vi "myRIO_BRig_RT_v0,71__PortC.vi"() -> ()   [LabVIEW 2014]
uses:
  <vilib>/Platform/TimedLoop/XDataNode/XDataNode.xnode
  <vilib>/Platform/TimedLoop/XDataNode/nitl_modes.ctl
  <vilib>/Platform/TimedLoop/XDataNode/XDNodeRunTimeDep.lvlib
  <vilib>/Platform/TimedLoop/XDataNode/wakeup.ctl
  <vilib>/Platform/TimedLoop/XDataNode/timing_clust.ctl
  <vilib>/rvi/interface/nirviReadWriteControl/nirviReadWriteControl.xnode
  <vilib>/rvi/interface/Simulation/niFpgaSimulationCallBeginRW.vi
  <vilib>/rvi/errors/niLvFpgaAdjustHostInterfaceError.vi
  <vilib>/rvi/interface/nirviCloseFPGA/nirviCloseFPGA.xnode
  <vilib>/myRIO/Instrument Drivers/Utilities/Utilities.lvlib
  <vilib>/rvi/interface/nirviOpenFPGA/nirviOpenFPGA.xnode
  myRIO_BRig_RT__Case_Exp_stateList.ctl
  <vilib>/WebDAVClient/Advanced/SessionHandle.ctl
  <vilib>/WebDAVClient/NI_WebDAV.lvlib
  myRIO_BRig_RT__Case_NonExp_stateList.ctl
  NiFpgaLv.dll
  <vilib>/Utility/error.llb/Error Cluster From Error Code.vi
  myRIO_BRig_FPGA_v3,60__PortC__build.lvbitx
  myRIO_BRig_FPGA_v3,60__PortC.vi
  <vilib>/FPGAPlugInAG/myRIO-1900/niLvFpga_Open_myRIO-1900.vi
  <vilib>/rvi/interface/common/dynamic/niFpgaDynamicAddResources.vi
  <vilib>/FPGAPlugInAG/Dynamic/niLvFpga_Close_Dynamic.vi
panel:
  out "I_connect_TCP":bool
  out "tempAI0":i16
  out "error out 5":errorcluster
  in  "get_countPerMS":bool
  in  "count_warmup_R_reset":bool
  in  "count_warmup_L_reset":bool
  out "count_warmup_R":u16
  out "count_warmup_L":u16
  out "SolenoidReward":bool
  in  "SolenoidProbability_L":u16=50 caption="Reward Time [ms]" min=1 max=1000 step=1
  in  "SolenoidProbability_R":u16=50 caption="Reward Time [ms]" min=1 max=1000 step=1
  out "output_PortA":dbl caption="LaserPower"
  out "error out 4":errorcluster
  in  "laser_power_step":dbl
  in  "laser_power_max":dbl
  in  "Recording":bool
  out "error out 3":errorcluster
  out "error out 2":errorcluster
  in  "laser_power_min":dbl
  in  "f_millisec2count":dbl=159.0
  in  "laser_Tshutter":dbl=2.0
  in  "laser_Freq":dbl=10.0
  in  "laser_Tpeak":dbl=2.0
  in  "laser_duration":u16
  out "error out":errorcluster
  in  "LC_Cue1_All_Count":u16
  in  "LC_Cue1_First_Count":u16
  in  "LC_Cue1_All_delayOpt":bool
  in  "LC_ENL1_All_delayOpt":bool
  in  "LC_ENL1_All_Count":u16
  in  "LC_ENL1_First_Count":u16
  in  "LC_Cue1_First_delayOpt":bool
  in  "LC_ENL1_First_delayOpt":bool
  in  "Tcycle_Cue_max":u16=1000 caption="Max" min=5 max=5000 step=5
  in  "Tcycle_Cue_min":u16=1000 caption="Min" min=5 max=5000 step=5
  in  "SendData":bool
  out "cSpout":enum16{"Left", "Right"}(ring) caption="Left or Right Spout"
  out "A4":u32 caption="LickCounter_Right"
  out "A2":u32 caption="LickCounter_Left"
  in  "laserResponse_wrong_LED":bool
  out "error_initTrial":errorcluster
  out "error_Selection_pre":errorcluster
  out "error_Selection":errorcluster
  out "SelectWrong":bool
  out "SelectReward":bool
  in  "Left(F)_or_Right(T)":bool
  in  "ignoreWrong":bool
  in  "SelectionState":bool
  in  "laserResponse_wrong":bool
  in  "laserResponse_reward":bool
  in  "laserResponse_reward_LED":bool
  out "nRewards_Right":u16 caption="# Rewards Total (Right)"
  out "nRewards_Left":u16 caption="# Rewards Total (Left)"
  out "nRewards_cur":u16 caption="# Rewards in Current Block"
  out "TpB_target":u16 caption="Target Trials Per Block"
  out "cState_NonExp":T1 caption="WarmUp State"
  out "iBlock":u16 caption="Current Block"
  out "cState":T2 caption="Experimental State"
  out "iTrial":u16 caption="Current Trial"
  in  "warmupType":u8(slide) max=2 step=1 scale=0.0..2.0
  in  "TestConnection":bool
  in  "warmup":bool caption="WarmUp"
  in  "Data Set Prefix":string="Exp1_TM2"
  out "Connected To Host?":bool
  in  "Host Password":string="sabalab"
  in  "Host UserName":string="Test2"
  in  "sp_RightSpout":u16(slide)=2 max=2 step=1 scale=0.0..2.0
  in  "sp_LeftSpout":u16(slide)=2 max=2 step=1 scale=0.0..2.0
  in  "BUR_max":u16 caption="Count Reward Structure  (0 = off)"
  in  "LC_Wrong_Probability":u16
  in  "LC_Wrong_Trial":u16(slide) max=2 step=1 scale=0.0..2.0
  in  "LC_Wrong_Block":u16(slide) max=2 step=1 scale=0.0..2.0
  in  "LC_Wrong_OnOff":bool
  in  "LC_Reward_Probability":u16
  in  "LC_Reward_Trial":u16(slide) max=2 step=1 scale=0.0..2.0
  in  "LC_Reward_Block":u16(slide) max=2 step=1 scale=0.0..2.0
  in  "LC_Reward_OnOff":bool
  in  "LC_Cue1_All_Probability":u16
  in  "LC_Cue1_All_Block":u16(slide) max=2 step=1 scale=0.0..2.0
  in  "LC_Cue1_All_OnOff":bool
  in  "LC_Cue1_First_Probability":u16
  in  "LC_Cue1_First_Block":u16(slide) max=2 step=1 scale=0.0..2.0
  in  "LC_Cue1_First_OnOff":bool
  in  "LC_ENL1_All_Probability":u16 max=100 step=1
  in  "LC_ENL1_All_Block":u16(slide) max=2 step=1 scale=0.0..2.0
  in  "LC_ENL1_All_OnOff":bool
  in  "LC_ENL1_First_Probability":u16 max=100 step=1
  in  "LC_ENL1_First_Block":u16(slide) max=2 step=1 scale=0.0..2.0
  in  "Tcycle_Timeout":u16=1000 caption="Timeout Time [ms]" min=10 max=10000 step=1
  in  "Tcycle_Wrong":u16=1000 caption="Wrong Time [ms]" min=10 max=10000 step=1
  in  "Tcycle_Selection":u16=1000 caption="Answer Time [ms]" min=1 max=10000 step=1
  in  "Tcycle_RewardPost":u16=1000 caption="Consumption Time [ms]" min=250 max=10000 step=250
  in  "Tcycle_Reward_L":u16=500 caption="Reward Time [ms]" min=1 max=1000 step=1
  in  "Tcycle_Reward_R":u16=500 caption="Reward Time [ms]" min=1 max=1000 step=1
  in  "TpB_Max_R":u16=4 caption="Max TrialsPerBlock" min=1 max=12 step=1
  in  "TpB_Min_R":u16=4 caption="Min TrialsPerBlock" min=1 max=12 step=1
  in  "TpB_Max_L":u16=4 caption="Max TrialsPerBlock" min=1 max=12 step=1
  in  "TpB_Min_L":u16=4 caption="Min TrialsPerBlock" min=1 max=12 step=1
  in  "BUR_min":u16 caption="Count Reward Structure\n(0 = off)"
  in  "TrialUntilReward":bool caption="Ignore Wrong Selection"
  in  "CueCycles":u16=1 caption="Cue Structure" min=1 max=1 step=1
  in  "MTrig_Laser_Tcycle":u16=10 caption="Time [ms]"
  in  "MTrig_Laser_trig":bool
  in  "MTrig_Audio_trig__R":bool caption="Trigger Audio"
  in  "MTrig_Audio_trig__L":bool caption="Trigger Audio"
  in  "RewCalib_Trig_R":bool caption="Calibrate_R"
  in  "RewCalib_Trig_L":bool caption="Calibrate_L"
  in  "MTrig_Solenoid_Tcycle__R":u16=300 caption="Time [ms]"
  in  "MTrig_Solenoid_Tcycle__L":u16=300 caption="Time [ms]"
  in  "MTrig_Solenoid_trig__R":bool caption="Solenoid"
  in  "MTrig_Solenoid_trig__L":bool caption="Solenoid"
  in  "STOP_abort":bool caption="Stop LabView\n(Stops myRio and FPGA)"
  in  "STOP_endBlock":bool caption="Stop Experiment\n@ End of Block"
  in  "STOP_endTrial":bool caption="Stop Experiment\n@ End of Trial"
  in  "START":bool caption="Start Experiment"
  in  "Tcycle_CuePenalty":u16=1000 caption="Penalty" min=1 max=10000 step=1
  in  "Audio_Amp__R":u16=100 caption="Amp"
  in  "Audio_Freq__R":u8=5 caption="Freq [kHz]" max=14 step=1
  in  "Audio_Amp__L":u16=100 caption="Amp"
  in  "Audio_Freq__L":u8=5 caption="Freq [kHz]" max=14 step=1
  in  "LC_Wrong_Tdelay":u16
  in  "LC_Cue1_All_Tdelay":u16
  in  "LC_ENL1_All_Tdelay":u16
  in  "LC_Reward_Tdelay":u16
  in  "LC_Cue1_First_Tdelay":u16
  in  "LC_ENL1_First_Tdelay":u16
  in  "LC_ENL1_First_OnOff":bool
  in  "Tcycle_ENLPenalty":u16=100 caption="Penalty" min=10 max=10000 step=10
  in  "Tcycle_ENL_max":u16=1000 caption="Max" min=250 max=10000 step=250
  in  "Tcycle_ENL_min":u16=1000 caption="Min" min=250 max=10000 step=250
  # "Experimental Run"
  # "Experiment Task Structure"
  # "Current State"
  # "Timing [ms]"
  # "Global Parameters\n \n   WarmUp State                                            Lick Counter"
  # "Min            Max            Penalty"
  # "(1) = Switching\n(2) = Two Choice"
  # "Enforced\nNonLick"
  # "Left                    Right"
  # "Cue"
  # "Experimental State"
  # "Communication (Host PC)"
  # "WarmUp"
  # "Selection\n \n \nReward\n    Dispense\n    Time\n \n    Dispense\n    Probability\n \n    Consumption\n    Time\n \nWrong Choice\n \n \nTimeout Penalty"
  # "Trial Parameters\n \n   Left/Right        Give Reward?        Laser Power [V]"
  # "Left                  Right"
  # "Min"
  # "Max"
  # "Block                   Trial            Target Trials       # Rewards \n                                                            Per Block             Current"
  # "Trial Per Block Structure \n               Left                        Right"
  # "Min"
  # "# Rewards Total\n                                                                  Left                    Right"
  # "Recording Rig"
  # "FPGA Conv."
  # "Cue then reward (no lick)\n \nLeft                    Right"
  # "Max"
  # "FPGA count per ms"
  # "Laser Control\n\n                               On/Off      Block        Probability [%]   Delay [ms]                              Count"
  # "Manual Control"
  # "Enforced\nNonLick\n      1"
  # "Solenoid\n \nLeft              Right"
  # "Speaker\n \nLeft                    Right"
  # "Laser"
  # "from end"
  # "Switch\nTrial"
  # "from start"
  # "from end"
  # "NonSwitch\nTrials"
  # "Time\n[ms]"
  # "Time\n[ms]"
  # "from start"
  # "Time = Cue Min"
  # "Cue 1"
  # "Power = Min"
  # "from end"
  # "Switch\nTrial"
  # "from start"
  # "Speaker Parameters"
  # "Laser Parameters"
  # "Left                  Right"
  # "from end"
  # "Frequency\n[Hz]"
  # "NonSwitch\nTrials"
  # "Frequency\n[kHz]"
  # "from start"
  # "Timing [ms]\n Duration     Peak Width   Shutter"
  # "Selection Reward"
  # "Amp\n(0 - 32,000)"
  # "Laser Power [V]\nMin          Max              Step"
  # "Speaker\nPattern\nDuring Cue"
  # "Selection Wrong"
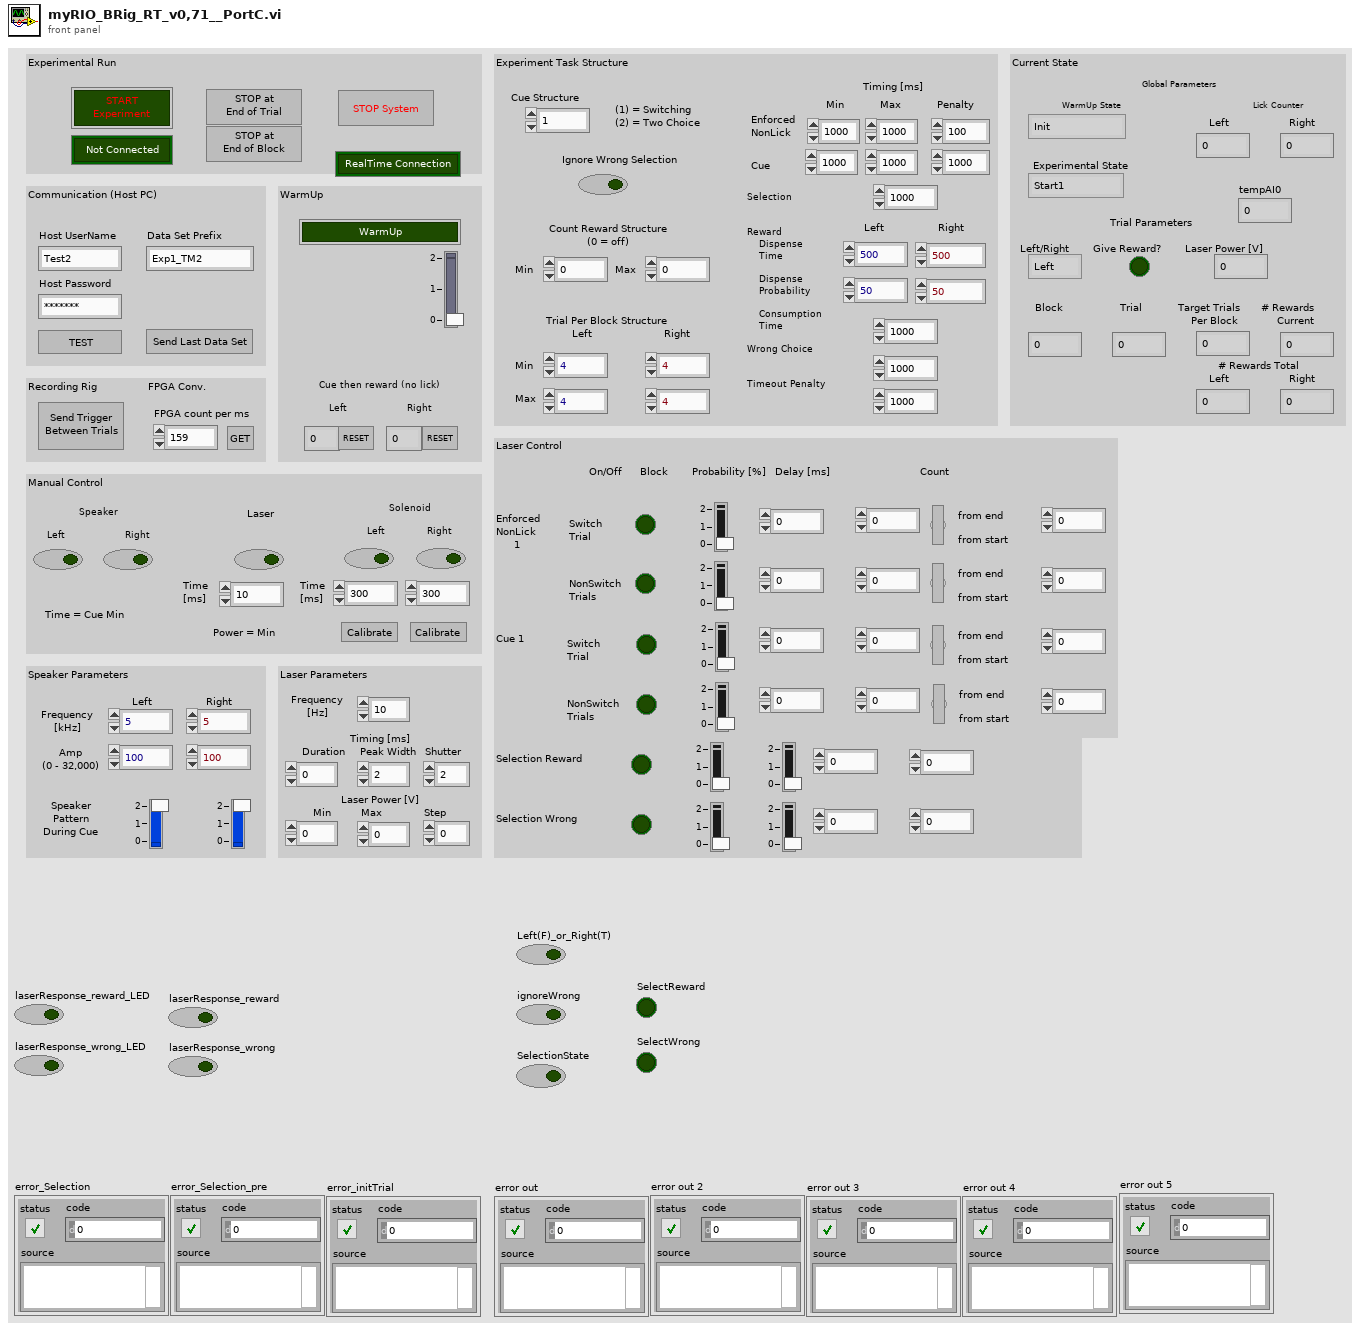
[diagram p1: front panel]
types:
  T1 = typedef "myRIO_BRig_RT__Case_NonExp_stateList.ctl" = enum16{"Init", "UploadSettings_pre", "UploadSettings_Read_dataExp", "UploadSettings_dataExp_1", "UploadSettings_Read_dataLC", "UploadSettings_dataLC_1", "UploadSettings_dataLC_2", "UploadSettings_Read_dataMTrig", "UploadSettings_dataMTrig_1", "UploadSettings_post", "Idle_pre", "IdleEmpty", "IdleEmpty2", "IdleEmpty3", "IdleEmpty4", "Idle", "Idle_2", "Idle_3", "Idle_4", "Idle_post", "Cue_pre__pre", "Cue_pre", "Cue", "Cue_post", "RewardCalibration_pre", "DispenseWater_pre__pre", "DispenseWater_pre", "DispenseWater", "DispenseWater_post", "TestConnection", "SendData", "Get_FPGA_count_per_ms", "End"}
  T2 = typedef "myRIO_BRig_RT__Case_Exp_stateList.ctl" = enum16{"Start1", "Start2", "Start3", "saveSettings1", "saveSettings2", "saveSettings3", "saveSettings4_LC_ENL", "saveSettings5_LC_Cue", "saveSettings6_LC_Other", "setSettings_Audio", "setSettings_Laser", "initBlock_pre", "initBlock", "initBlock2", "initBlock_post", "initTrial_pre", "initTrial", "initTrial2", "initTrial3", "initTrial4", "initTrial_LC_ENL1", "initTrial_LC_Cue1", "initTrial_LC_Sel", "initTrial_post", "ENL1_pre", "ENL1", "ENL1_post", "ENL1Penalty_pre", "ENL1Penalty", "ENL2_pre", "ENL2", "ENL2Penalty_pre", "ENL2Penalty", "Cue1_pre", "Cue1", "Cue1_post", "Cue1Penalty_pre", "Cue1Penalty", "Cue2_pre", "Cue2", "Cue2Penalty_pre", "Cue2Penalty", "Selection_pre", "Selection", "Select_post", "SelectReward_pre", "SelectReward", "SelectRewardPost_pre", "SelectRewardPost", "SelectWrong_pre", "SelectWrong", "SelectWrong_post", "SelectTimeout_pre", "SelectTimeout", "SelectTimeout_post", "endTrial_pre", "endTrial1", "endTrial2", "endTrial3", "endTrial_post", "endBlock_pre", "endBlock", "endBlock_post", "endExp", "commConnect", "commUpload_pre", "commUpload_dataBlock", "commUpload_dataCurrent", "commUpload_dataExp", "commUpload_dataLC", "commUpload_dataTrial", "commUpload_post", "saveData_pre", "saveData_dataBlock", "saveData_dataCurrent", "saveData_dataExp", "saveData_dataLC", "saveData_dataTrial", "saveData_post", "empty_endBlock1", "empty_endBlock2", "empty_endTrial1", "empty_endTrial2", "empty_endTrial3", "empty_endTrial4", "empty_endTrial5"}
  T3 = typedef "XDNodeRunTimeDep.lvlib/timing_clust.ctl" = cluster{"Expected End [f-1]":u64, "Actual End [f-1]":u64, "Finished Late? [f-1]":bool, "Expected End [i-1]":u64, "Actual End [i-1]":u64, "Finished Late? [i-1]":bool, "Expected Start [i]":u64, "Actual Start [i]":u64, "Expected Start [f]":u64, "Actual Start [f]":u64, "Source Name":string, "Structure Name":string, "Period":i64, "Deadline":i64, "Offset":i64, "Start":i64, "Priority":i32, "Timeout":i32, "Mode":T4, "Wakeup Reason":T5, "Error":errorcluster, "Source Type":string, "Secondary Source Type":string, "Global End Time":u64, "Global Start Time":u64, "Frame Duration":u64, "Iteration Duration":u64, "Assigned CPU":i32, "I/O Scan Engine Mode":u32}
  T4 = typedef "XDNodeRunTimeDep.lvlib/nitl_modes.ctl" = enum32{"No Change", "Process missed periods, maintain original phase", "Discard missed periods, maintain original phase", "Process missed periods, ignore original phase", "Discard missed periods, ignore original phase"}
  T5 = typedef "XDNodeRunTimeDep.lvlib/wakeup.ctl" = enum32{"Normal", "Aborted", "Asynchronous wakeup", "Timing source error", "Timed loop error", "Timeout"}
  T6 = typedef "NI_WebDAV.lvlib/SessionHandle.ctl" = refnum<k1>
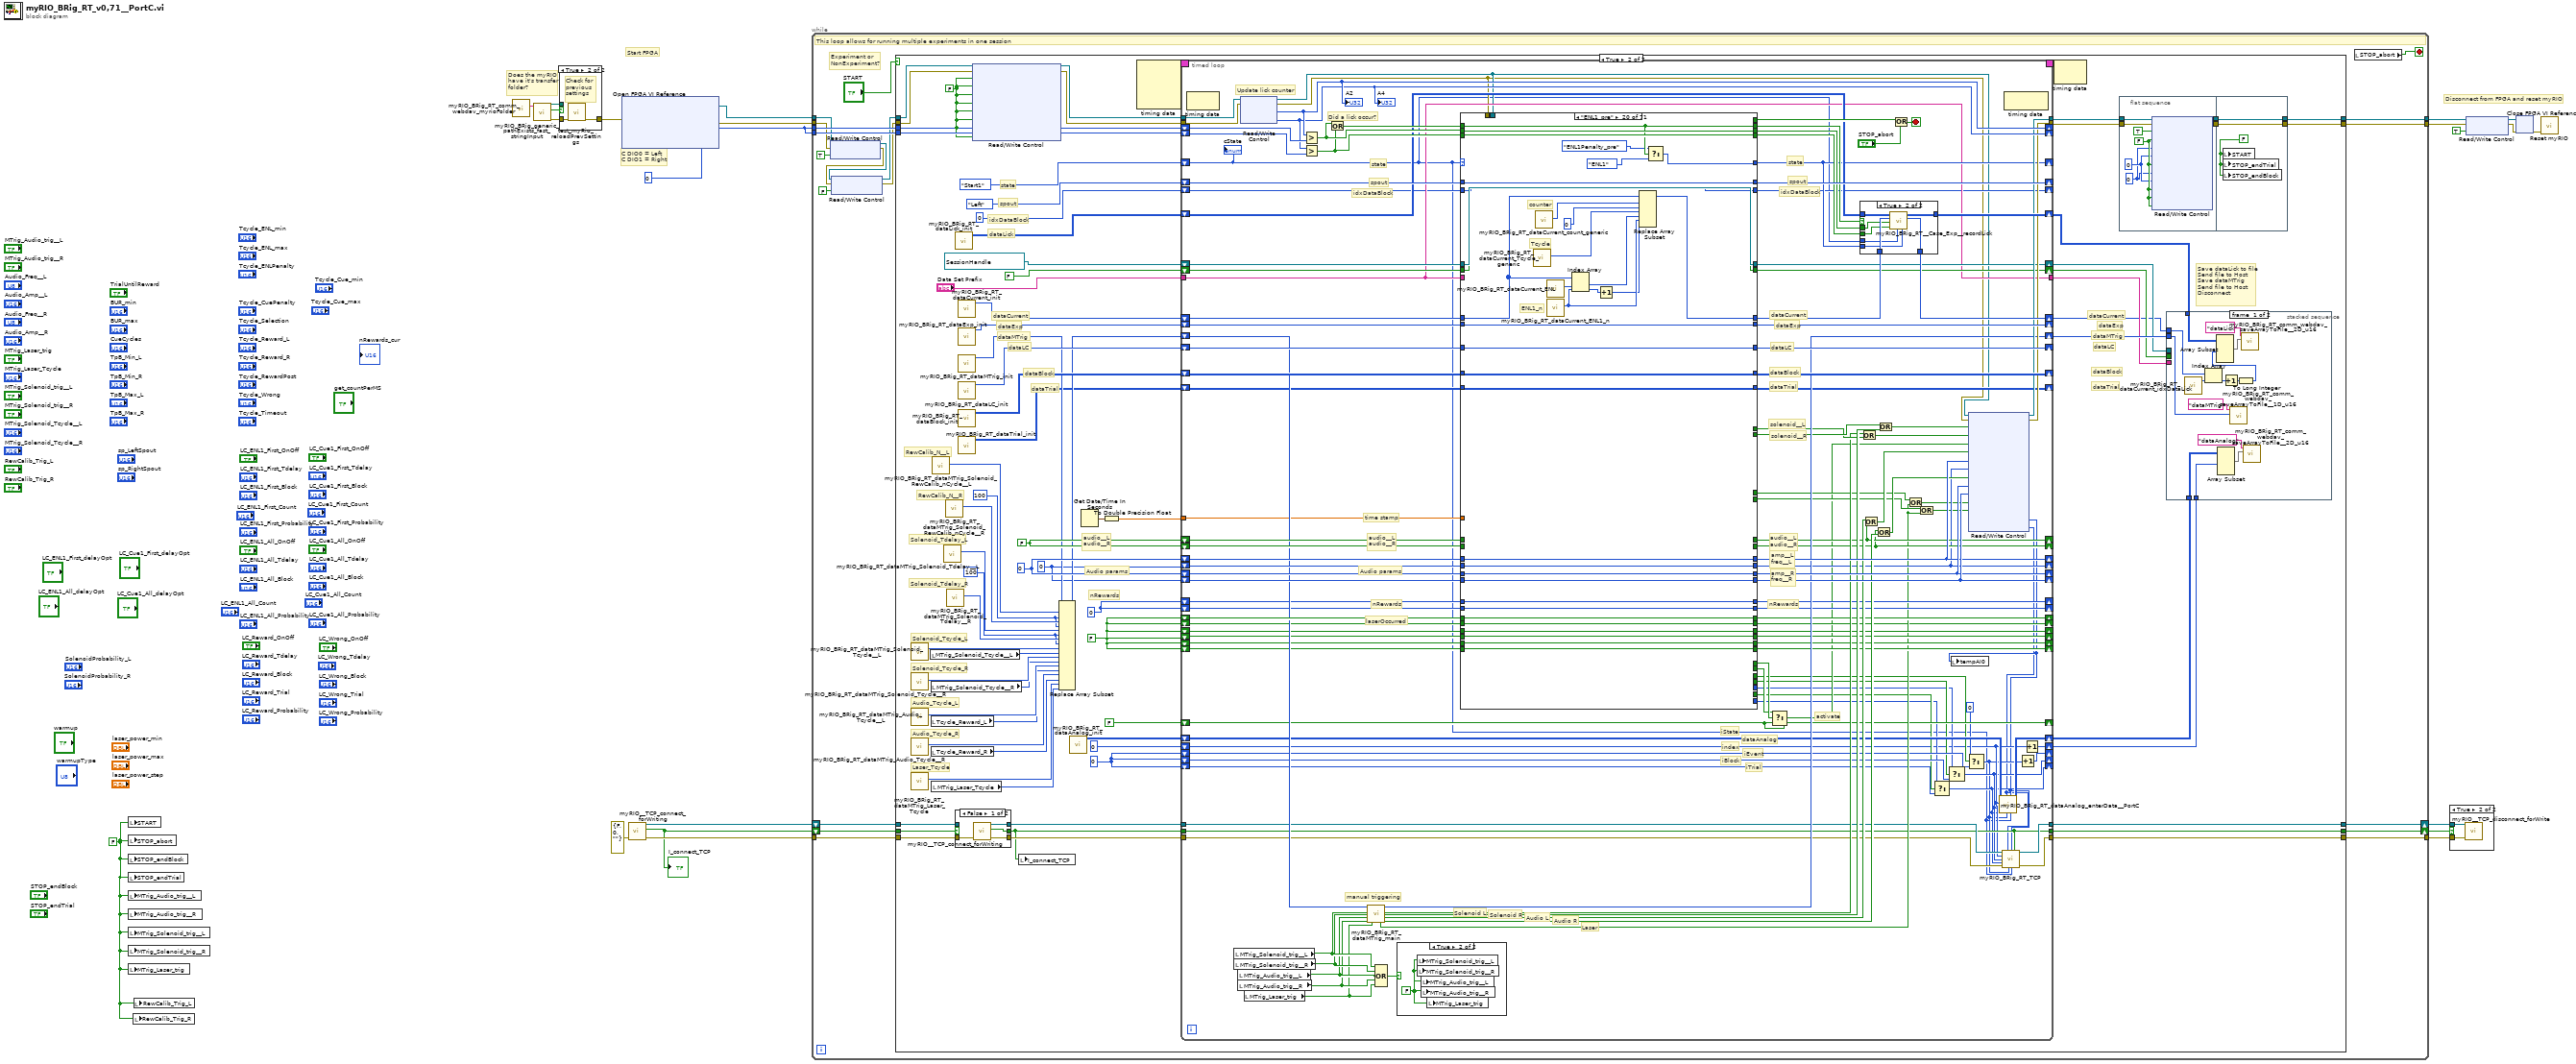
[diagram p0: block diagram]
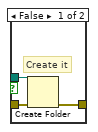
[diagram p3: hidden frame]
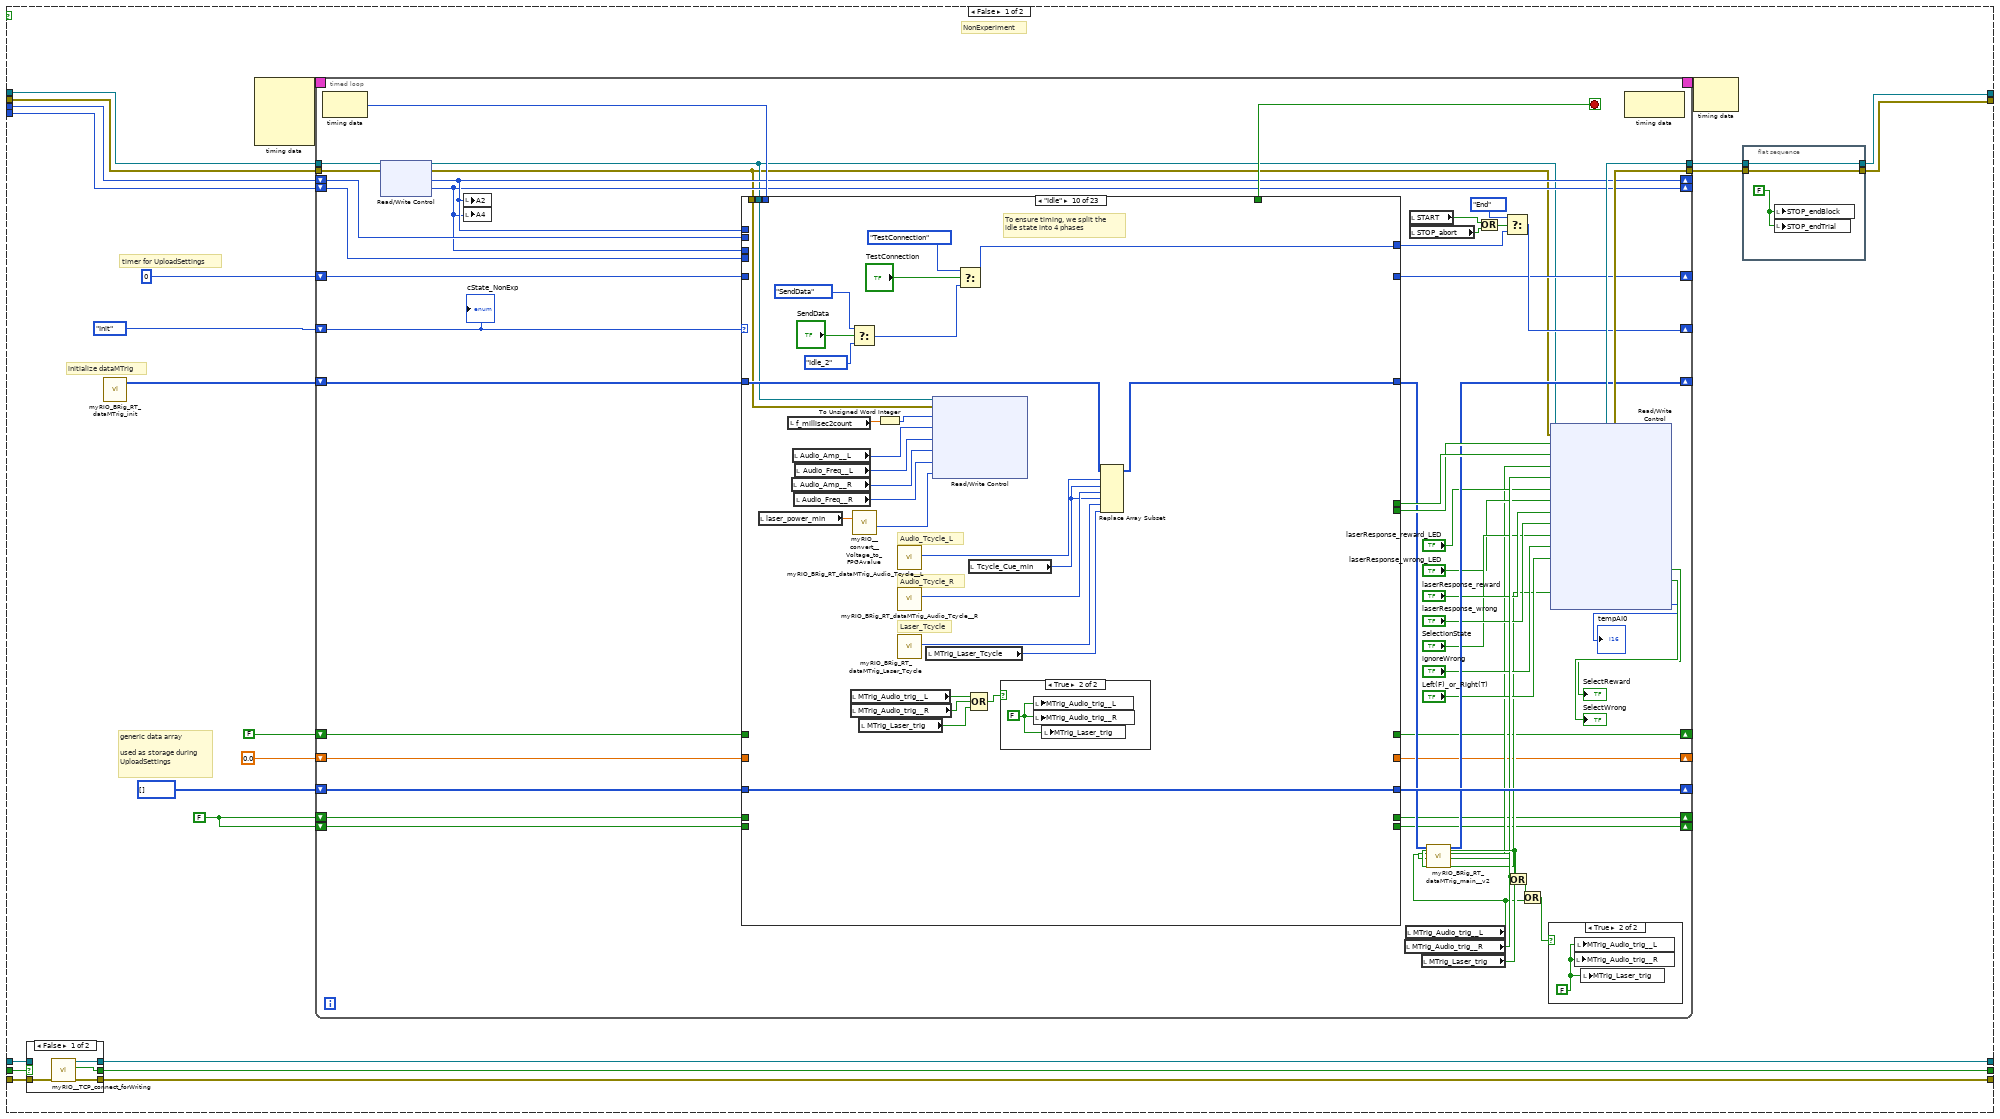
[diagram p4: hidden frame]
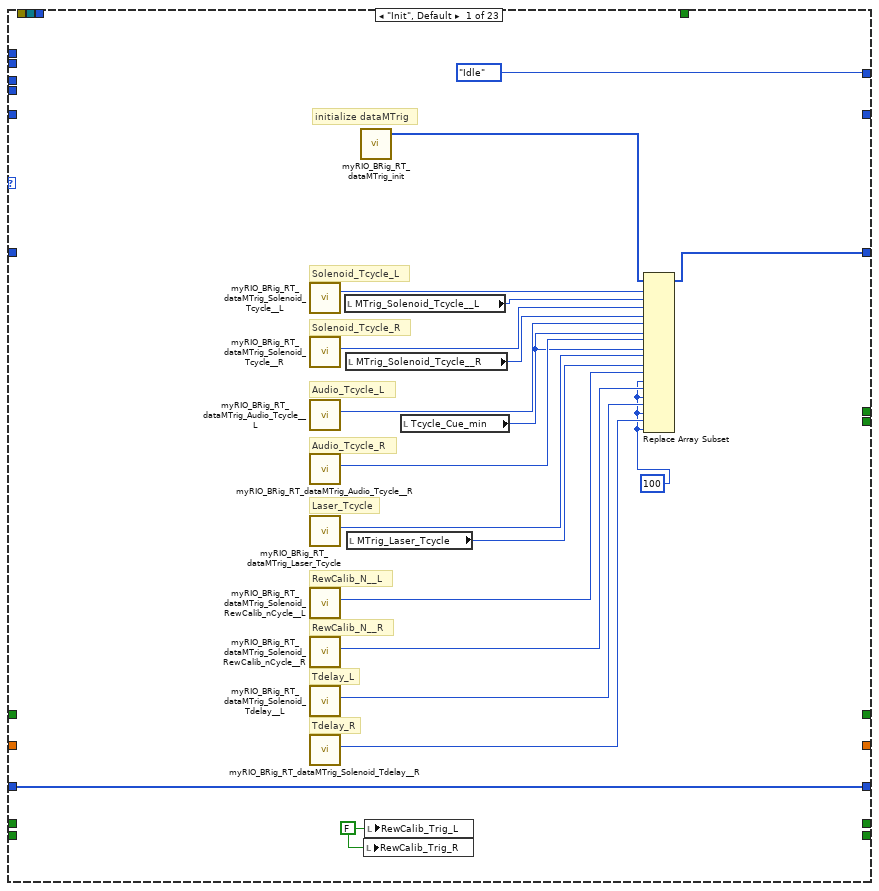
[diagram p7: hidden frame]
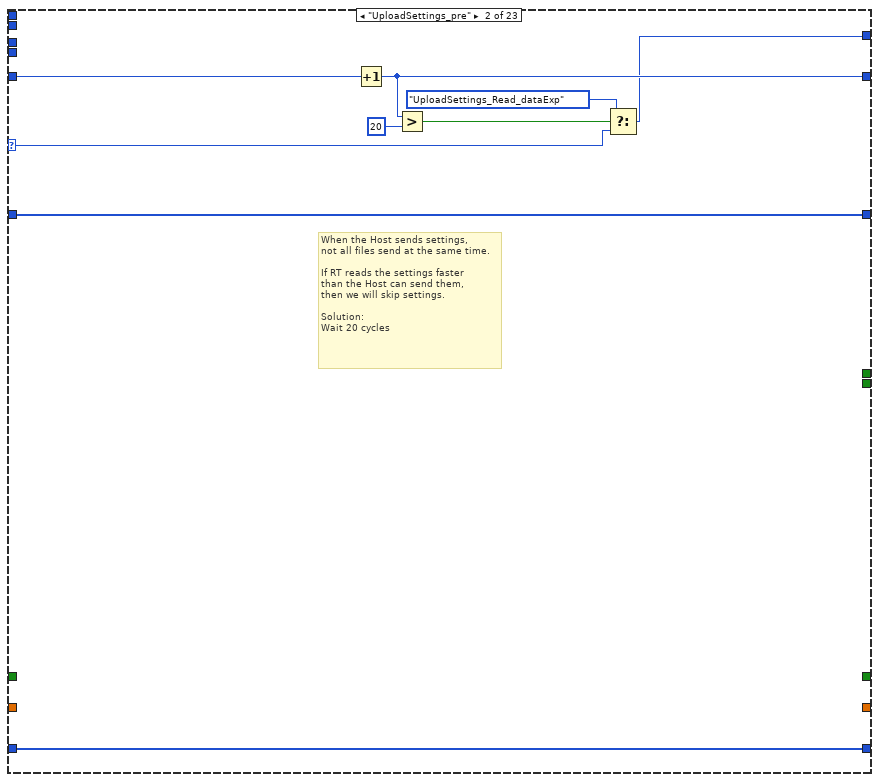
[diagram p8: hidden frame]
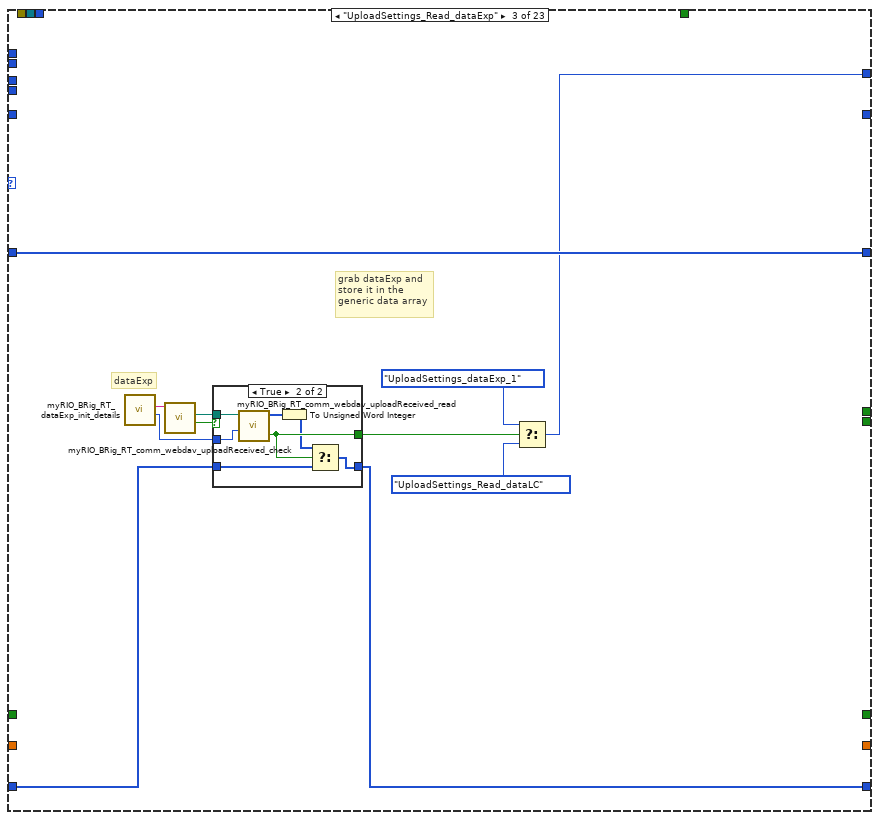
[diagram p9: hidden frame]
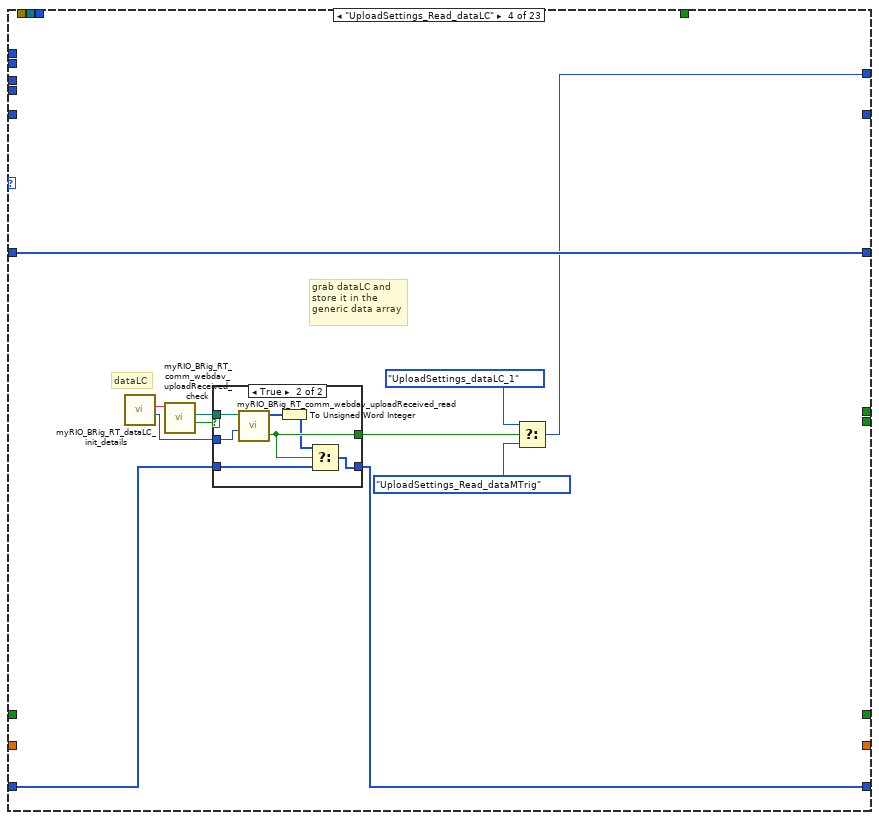
[diagram p11: hidden frame]
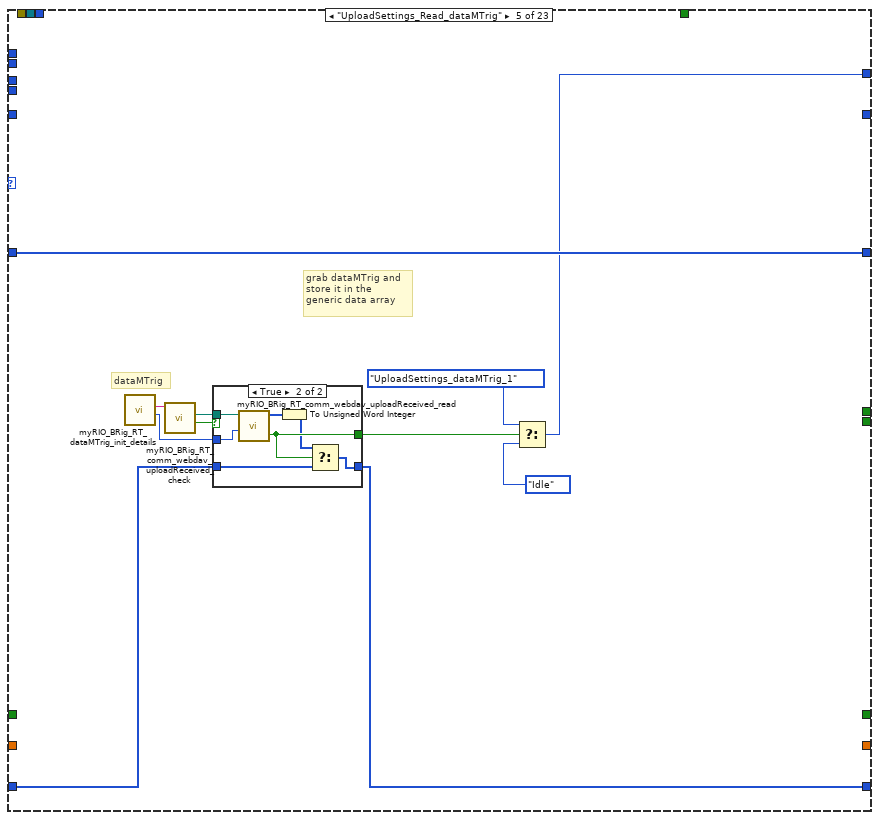
[diagram p13: hidden frame]
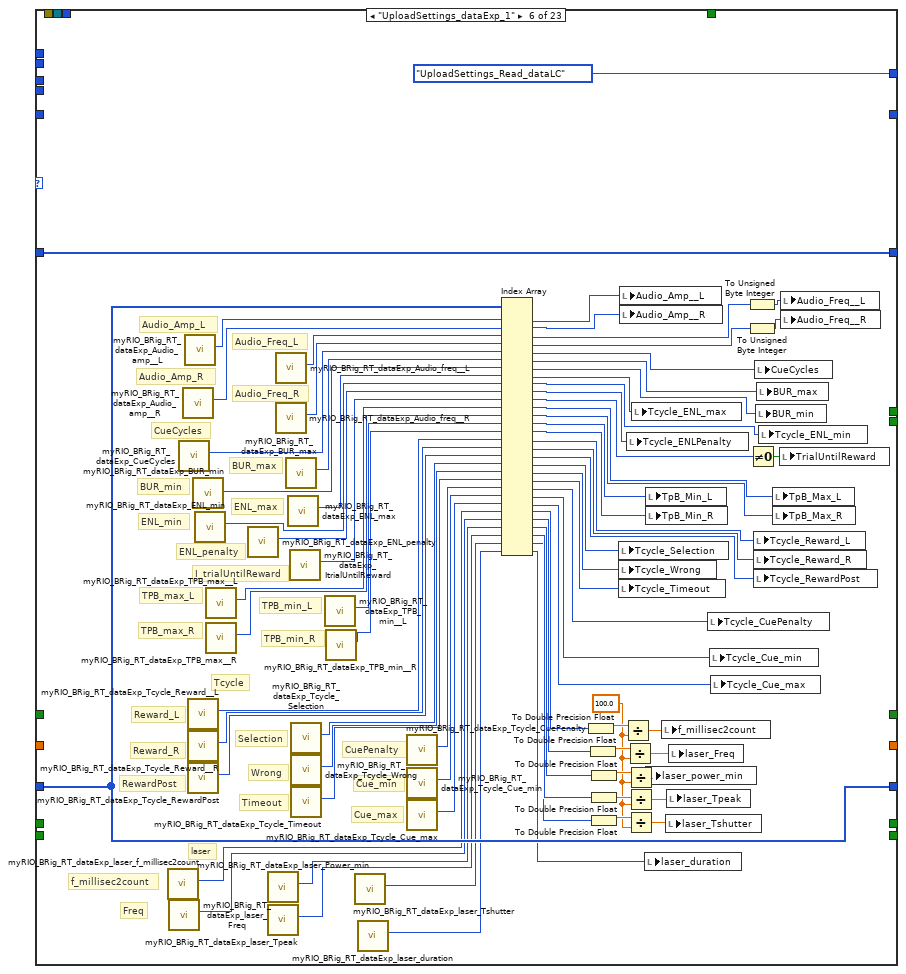
[diagram p15: hidden frame]
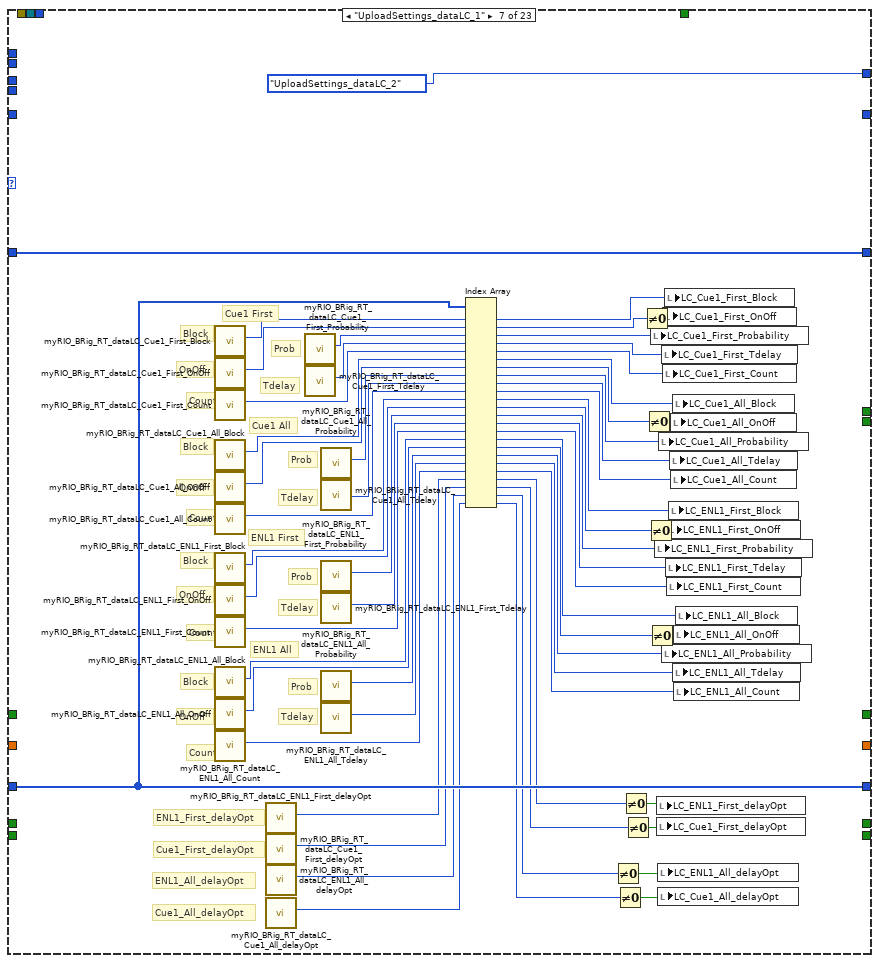
[diagram p16: hidden frame]
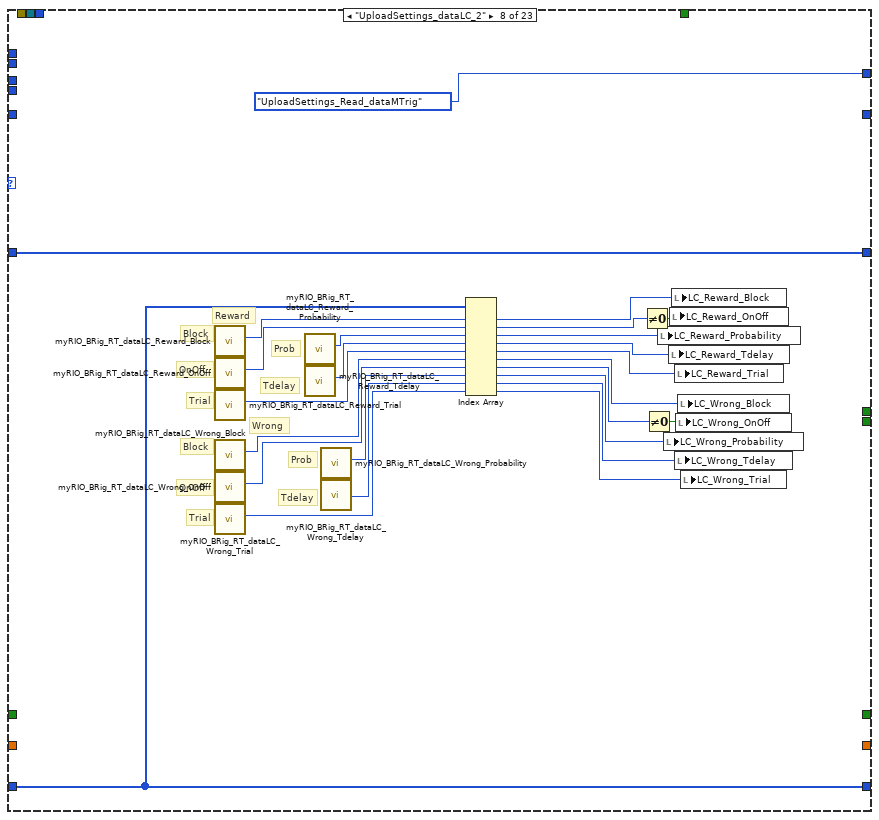
[diagram p17: hidden frame]
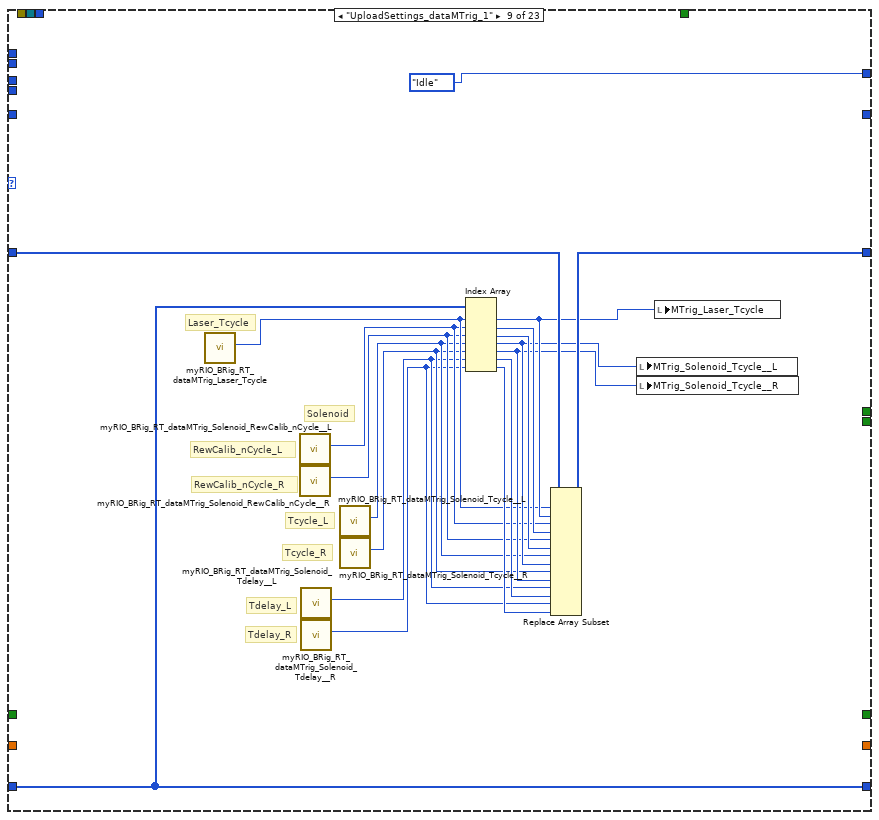
[diagram p18: hidden frame]
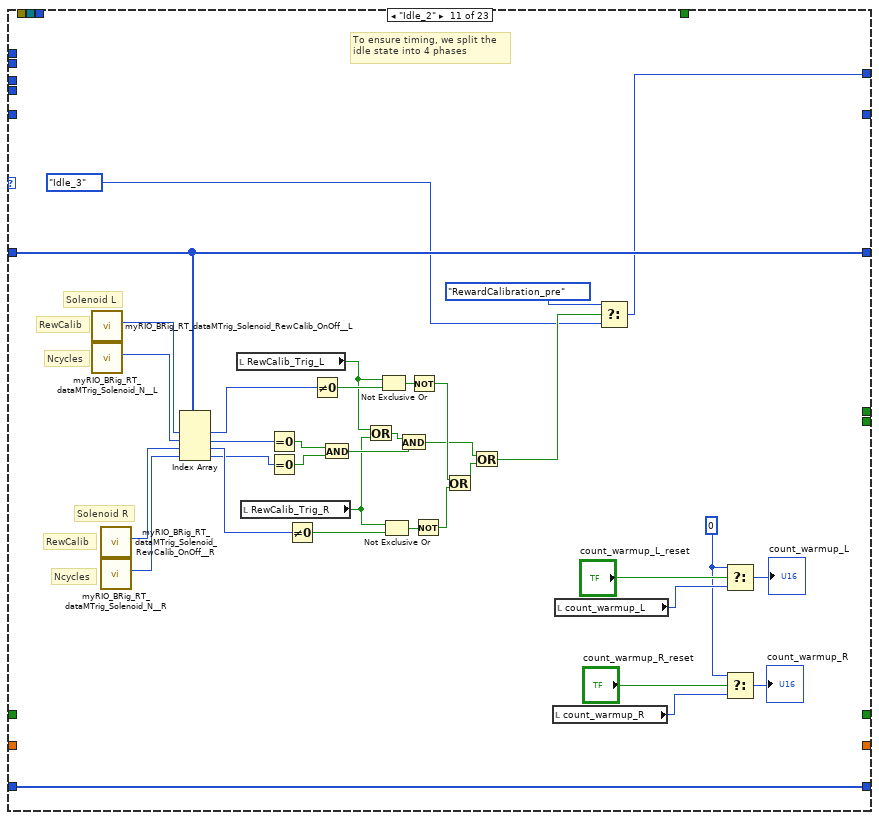
[diagram p20: hidden frame]
diagram:
  w16 = u32 0
  w13 = FALSE
  # "Does the myRIO\nhave it's transfer\nfolder?"
  # "C DIO0 = Left\nC DIO1 = Right"
  # "Start FPGA"
  # "Disconnect from FPGA and reset myRIO"
  n1 = local write "START"(w13) -> ()
  n2 = local write "STOP_abort"(w13) -> ()
  n3 = local write "STOP_endBlock"(w13) -> ()
  n4 = local write "STOP_endTrial"(w13) -> ()
  n5 = local write "MTrig_Audio_trig__L"(w13) -> ()
  n6 = local write "MTrig_Audio_trig__R"(w13) -> ()
  n7 = local write "MTrig_Solenoid_trig__L"(w13) -> ()
  n8 = local write "MTrig_Solenoid_trig__R"(w13) -> ()
  n9 = local write "MTrig_Laser_trig"(w13) -> ()
  n10 = local write "RewCalib_Trig_R"(w13) -> ()
  n11 = local write "RewCalib_Trig_L"(w13) -> ()
  n12 = call "myRIO_BRig_RT_comm_webdav_myrioFolder.vi"() -> ("output_myrioFolder"=w12:string)  [unwired: 11 in]
  n13 = call "myRIO_BRig_generic_pathExists_fast_stringInput.vi"("input_filePath"=w12) -> ("output_error"=w11:errorcluster, "output_Iexist"=w10:bool, "output_filePath"=w9:path)  [unwired: 8 in]
  n14 = case shown="True" w10 {
    tunnel: w9 -> [w25 _]
    tunnel: w11 -> [w24 w27]
    tunnel: [w23 w26] -> w7
    frame False {
      # "Create it"
      n15 = Create Folder(path (use dialog)=w25, error in=w24) -> (error out=w23:errorcluster)  [unwired: 1 in, 2 out]
    }
    frame True {
      # "Check for\nprevious\nsettings"
      n16 = call "test_myRio_reloadPrevSettings.vi"("input_error"=w27) -> ("output_error"=w26:errorcluster)  [unwired: 10 in]
    }
  }
  n17 = xnode "Open FPGA VI Reference"("error in"=w7) -> ("FPGA VI Reference Out"=w18:refnum<k20>, "error out"=w17:errorcluster)  [unwired: 1 in]
  n18 = call "myRIO__TCP_connect_forWriting.vi"("input_error"=errorcluster {"status"=FALSE, "code"=0, "source"=""}) -> ("output_error"=w5:errorcluster, "output_connected"=w4:bool, "output_hTCP"=w8:refnum<k5>)  [unwired: 8 in]
  "I_connect_TCP" <- w4
  n19 = while {
    tunnel: w18 -> [w37]
    tunnel: w17 -> [w42]
    tunnel: w16 -> [w45]
    tunnel: w16 -> [w44]
    tunnel: [w35] -> w15
    tunnel: [w34] -> w14
    shift-right: [w31] -> w3
    shift-left: w4 -> [w32]
    tunnel: w5 -> [w30]
    shift-right: [w29] -> w2
    shift-left: w8 -> [w33]
    tunnel: [w28] -> w1
    stop <- w43 stop-if-true
    # "Experiment or\nNonExperiment?"
    # "This loop allows for running multiple experiments in one session"
    n20 = xnode "Read/Write Control"("FPGA VI Reference In"=w37, "error in"=w42, "Counts_Reset"=TRUE) -> ("FPGA VI Reference Out"=w39:refnum<k20>, "error out"=w40:errorcluster)
    n21 = xnode "Read/Write Control"("FPGA VI Reference In"=w39, "error in"=w40, "Counts_Reset"=FALSE) -> ("FPGA VI Reference Out"=w36:refnum<k20>, "error out"=w38:errorcluster)
    n22 = case shown="True" "START" {
      tunnel: w45 -> [w66 w992]
      tunnel: w44 -> [w65 w991]
      tunnel: w38 -> [w63 w942]
      tunnel: w36 -> [w64 w941]
      tunnel: [w61 w988] -> w35
      tunnel: [w59 w983] -> w34
      tunnel: w33 -> [w52 w926]
      tunnel: [w50 w931] -> w29
      tunnel: w32 -> [w51 w929]
      tunnel: [w49 w930] -> w31
      tunnel: w30 -> [w53 w928]
      tunnel: [w48 w924] -> w28
      frame False {
        w56 = FALSE
        # "generic data array\n\nused as storage during\nUploadSettings"
        # "timer for UploadSettings"
        # "initialize dataMTrig"
        # "NonExperiment"
        n23 = case shown="False" w51 {
          selector: w51 -> [_ w75]
          tunnel: w53 -> [w72 w77]
          tunnel: [w73 w77] -> w48
          tunnel: w52 -> [_ w76]
          tunnel: [w74 w76] -> w50
          tunnel: [w71 w75] -> w49
          frame False {
            n24 = call "myRIO__TCP_connect_forWriting.vi"("input_error"=w72) -> ("output_error"=w73:errorcluster, "output_connected"=w71:bool, "output_hTCP"=w74:refnum<k5>)  [unwired: 8 in]
          }
          frame True {
          }
        }
        n25 = call "myRIO_BRig_RT_dataMTrig_init.vi"() -> ("output_dataMTrig"=w67:u16[])  [unwired: 5 in]
        n26 = node-c288() -> (w70:T3)  [unwired: 4 in]
        n27 = timed-loop {
          timing: w70 -> [_]
          timing-out: [_] -> w69
          shift-right: [w121] -> _
          shift-left: w67 -> [w133]
          shift-right: [w110] -> _
          shift-left: myRIO_BRig_RT__Case_NonExp_stateList."Init" ("Enum") -> [w127]
          shift-right: [w94] -> _
          shift-left: w66 -> [w95]
          shift-right: [w92] -> _
          shift-left: w65 -> [w93]
          tunnel: [w129] -> w62
          tunnel: [w128] -> w60
          tunnel: w63 -> [w131]
          tunnel: w64 -> [w130]
          shift-right: [w126] -> _
          shift-left: u16[] [] ("output_data") -> [w125]
          shift-right: [w96] -> _
          shift-left: u16 0 ("Audio_Amp__L") -> [w97]
          shift-right: [w89] -> _
          shift-left: w56 -> [w91]
          shift-right: [w88] -> _
          shift-left: w56 -> [w90]
          shift-right: [w84] -> _
          shift-left: FALSE -> [w85]
          shift-right: [w82] -> _
          shift-left: 0.0 -> [w83]
          stop <- w134 stop-if-true
          n28 = node-c288() -> (w132:i64)  [unwired: 1 in]
          n29 = xnode "Read/Write Control"("FPGA VI Reference In"=w130, "error in"=w131) -> ("FPGA VI Reference Out"=w87:refnum<k20>, "error out"=w86:errorcluster, "A2_LickL"=w94:u32, "A4_LickR"=w92:u32)
          n30 = local write "A2"(w94) -> ()
          n31 = local write "A4"(w92) -> ()
          n32 = case shown="\"Idle\"" w127 {
            selector: w127 -> [_ w159 _ _ _ _ _ _ _ _ _ _ _ _ w590 _ _ w798 _ _ _ w873 w917]
            tunnel: [myRIO_BRig_RT__Case_NonExp_stateList."Idle" ("Enum") w157 w164 w183 w202 myRIO_BRig_RT__Case_NonExp_stateList."UploadSettings_Read_dataLC" ("Enum") myRIO_BRig_RT__Case_NonExp_stateList."UploadSettings_dataLC_2" ("Enum") myRIO_BRig_RT__Case_NonExp_stateList."UploadSettings_Read_dataMTrig" ("f") myRIO_BRig_RT__Case_NonExp_stateList."Idle" ("Enum") w421 w438 w477 w558 myRIO_BRig_RT__Case_NonExp_stateList."Cue" ("t") w585 myRIO_BRig_RT__Case_NonExp_stateList."DispenseWater_pre" ("Enum") w743 w796 w819 myRIO_BRig_RT__Case_NonExp_stateList."Idle" ("Enum") myRIO_BRig_RT__Case_NonExp_stateList."Idle" ("Enum") w872 w917] -> w111
            tunnel: [w146 w156 w174 w193 w212 w297 w356 w381 w397 w425 w453 w482 w556 w574 w591 w653 w780 w803 w830 w865 w871 w884 w915] -> w122
            tunnel: [_ _ _ _ _ _ _ _ _ _ _ _ _ _ _ _ _ _ _ _ _ _ TRUE] -> w134
            tunnel: w133 -> [_ w156 w174 w193 w212 w297 w356 w381 w398 w424 w453 w483 w556 w575 w592 w639 w776 w804 w831 w865 w871 w884 w915]
            tunnel: w132 -> [_ _ _ _ _ _ _ _ _ _ _ _ _ _ _ _ _ w808 _ _ _ _ _]
            tunnel: [w139 w155 w165 w184 w203 w246 w312 w357 w382 w416 w437 w471 w555 w564 w599 w634 w728 w781 w812 w857 w869 w883 w914] -> w126
            tunnel: w125 -> [w139 w155 w166 w185 w204 w246 w312 w357 w382 w416 w437 w471 w555 w564 w599 w634 w728 w781 w812 w857 w869 w883 w914]
            tunnel: [_ _ _ _ _ _ _ _ _ _ _ _ _ _ _ _ _ w805 _ _ _ _ _] -> w124
            tunnel: [_ _ _ _ _ _ _ _ _ _ _ _ _ _ _ _ _ w787 _ _ _ _ _] -> w123
            tunnel: w97 -> [_ w163 _ _ _ _ _ _ _ _ _ _ _ _ _ _ _ _ _ _ _ _ _]
            tunnel: [_ w162 _ _ _ _ _ _ _ _ _ _ _ _ _ _ _ _ _ _ _ _ _] -> w96
            tunnel: w95 -> [_ _ _ _ _ _ _ _ _ _ _ _ _ _ w596 _ _ _ _ _ _ _ _]
            tunnel: w94 -> [_ _ _ _ _ _ _ _ _ _ _ _ _ _ w597 _ _ _ _ _ _ _ _]
            tunnel: w93 -> [_ _ _ _ _ _ _ _ _ _ _ _ _ _ w594 _ _ _ _ _ _ _ _]
            tunnel: w92 -> [_ _ _ _ _ _ _ _ _ _ _ _ _ _ w595 _ _ _ _ _ _ _ _]
            tunnel: w91 -> [_ _ _ _ _ _ _ _ _ _ _ _ _ _ w582 _ _ _ _ _ _ _ _]
            tunnel: w90 -> [_ _ _ _ _ _ _ _ _ _ _ _ _ _ w581 _ _ _ _ _ _ _ _]
            tunnel: [_ _ _ _ _ _ _ _ _ _ _ _ _ w563 w582 _ _ _ _ _ _ _ _] -> w89
            tunnel: [_ _ _ _ _ _ _ _ _ _ _ _ _ w562 w581 _ _ _ _ _ _ _ _] -> w88
            tunnel: w87 -> [_ _ _ _ _ _ _ _ _ w407 _ _ _ _ _ _ _ _ _ _ _ w878 _]
            tunnel: w86 -> [_ _ _ _ _ _ _ _ _ w406 _ _ _ _ _ _ _ _ _ _ _ w877 _]
            tunnel: w85 -> [_ _ _ _ _ _ _ _ _ _ _ _ _ _ _ _ _ _ _ _ _ w882 _]
            tunnel: [_ _ _ _ _ _ _ _ _ _ _ _ _ _ _ _ _ _ _ _ _ TRUE _] -> w84
            tunnel: w83 -> [_ _ _ _ _ _ _ _ _ _ _ _ _ _ _ _ _ _ _ _ _ w880 _]
            tunnel: [_ _ _ _ _ _ _ _ _ _ _ _ _ _ _ _ _ _ _ _ _ w879 _] -> w82
            frame "Init", Default {
              w140 = FALSE ("RewCalib_Trig_L")
              w136 = u16 100 ("new element/subarray")
              # "Tdelay_R"
              # "Tdelay_L"
              # "RewCalib_N__R"
              # "RewCalib_N__L"
              # "Solenoid_Tcycle_R"
              # "Solenoid_Tcycle_L"
              # "Laser_Tcycle"
              # "Audio_Tcycle_R"
              # "Audio_Tcycle_L"
              # "initialize dataMTrig"
              n33 = call "myRIO_BRig_RT_dataMTrig_Solenoid_Tcycle__L.vi"() -> ("output_Solenoid_Tcycle__L"=w148:i32)  [unwired: 11 in]
              n34 = call "myRIO_BRig_RT_dataMTrig_Solenoid_Tcycle__R.vi"() -> ("output_Solenoid_Tcycle__R"=w149:i32)  [unwired: 11 in]
              n35 = call "myRIO_BRig_RT_dataMTrig_Audio_Tcycle__L.vi"() -> ("output_Audio_Tcycle__L"=w150:i32)  [unwired: 11 in]
              n36 = call "myRIO_BRig_RT_dataMTrig_Audio_Tcycle__R.vi"() -> ("output_Audio_Tcycle__R"=w151:i32)  [unwired: 11 in]
              n37 = call "myRIO_BRig_RT_dataMTrig_Laser_Tcycle.vi"() -> ("output_Laser_Tcycle"=w152:i32)  [unwired: 11 in]
              n38 = call "myRIO_BRig_RT_dataMTrig_Solenoid_RewCalib_nCycle__L.vi"() -> ("output_Solenoid_RewCalib_nCycle__L"=w144:i32)  [unwired: 11 in]
              n39 = call "myRIO_BRig_RT_dataMTrig_Solenoid_RewCalib_nCycle__R.vi"() -> ("output_Solenoid_RewCalib_nCycle__R"=w143:i32)  [unwired: 11 in]
              n40 = call "myRIO_BRig_RT_dataMTrig_Solenoid_Tdelay__L.vi"() -> ("output_Solenoid_Tdelay__L"=w142:i32)  [unwired: 11 in]
              n41 = call "myRIO_BRig_RT_dataMTrig_Solenoid_Tdelay__R.vi"() -> ("output_Solenoid_Tdelay__R"=w141:i32)  [unwired: 11 in]
              n42 = local read "MTrig_Solenoid_Tcycle__L"() -> (w153:u16)
              n43 = local read "MTrig_Solenoid_Tcycle__R"() -> (w154:u16)
              n44 = local read "MTrig_Laser_Tcycle"() -> (w137:u16)
              n45 = call "myRIO_BRig_RT_dataMTrig_init.vi"() -> ("output_dataMTrig"=w147:u16[])  [unwired: 5 in]
              n46 = local write "RewCalib_Trig_R"(w140) -> ()
              n47 = local write "RewCalib_Trig_L"(w140) -> ()
              n48 = local read "Tcycle_Cue_min"() -> (w138:u16)
              n49 = Replace Array Subset(array=w147, new element #1=w153, index #1=w148, new element #2=w154, index #2=w149, new element #3=w138, index #3=w150, new element #4=w138, index #4=w151, new element #5=w137, index #5=w152, new element #6=w136, index #6=w144, new element #7=w136, index #7=w143, new element #8=w136, index #8=w142, new element #9=w136, index #9=w141) -> (w146:u16[])
            }
            frame "UploadSettings_pre" {
              # "When the Host sends settings,\nnot all files send at the same time.\n\nIf RT reads the settings faster\nthan the Host can send them,\nthen we will skip settings.\n\nSolution:\nWait 20 cycles"
              n50 = Increment(x=w163) -> (x+1=w162:u16)
              n51 = Greater?(x=w162, y=u16 20) -> (0:w160:bool)
              n52 = Select(t=myRIO_BRig_RT__Case_NonExp_stateList."UploadSettings_Read_dataExp", s=w160, f=w159) -> (s? t:f=w157:T1)
            }
            frame "UploadSettings_Read_dataExp" {
              # "grab dataExp and\nstore it in the\ngeneric data array"
              # "dataExp"
              n53 = call "myRIO_BRig_RT_dataExp_init_details.vi"() -> ("output_dataSize"=w170:i32, "output_dataName"=w173:string)  [unwired: 10 in]
              n54 = call "myRIO_BRig_RT_comm_webdav_uploadReceived_check.vi"("input_dataName"=w173) -> ("output_Iexist"=w172:bool, "output_dataPath"=w171:path)  [unwired: 9 in]
              n55 = case shown="True" w172 {
                tunnel: w171 -> [_ w182]
                tunnel: w170 -> [_ w181]
                tunnel: [_ w180] -> w169
                tunnel: w166 -> [w175 w179]
                tunnel: [w175 w176] -> w165
                frame False {
                }
                frame True {
                  n56 = call "myRIO_BRig_RT_comm_webdav_uploadReceived_read.vi"("input_dataSize"=w181, "input_filePath"=w182) -> ("output_Ivalid"=w180:bool, "output_data"=w178:i64[])  [unwired: 8 in]
                  n57 = To Unsigned Word Integer(number=w178) -> (unsigned 16bit integer=w177:u16[])
                  n58 = Select(t=w177, s=w180, f=w179) -> (s? t:f=w176:u16[])
                }
              }
              n59 = Select(t=myRIO_BRig_RT__Case_NonExp_stateList."UploadSettings_dataExp_1", s=w169, f=myRIO_BRig_RT__Case_NonExp_stateList."UploadSettings_Read_dataLC" ("t")) -> (s? t:f=w164:T1)
            }
            frame "UploadSettings_Read_dataLC" {
              # "grab dataLC and\nstore it in the\ngeneric data array"
              # "dataLC"
              n60 = call "myRIO_BRig_RT_dataLC_init_details.vi"() -> ("output_dataSize"=w189:i32, "output_dataName"=w192:string)  [unwired: 10 in]
              n61 = call "myRIO_BRig_RT_comm_webdav_uploadReceived_check.vi"("input_dataName"=w192) -> ("output_Iexist"=w191:bool, "output_dataPath"=w190:path)  [unwired: 9 in]
              n62 = case shown="True" w191 {
                tunnel: w190 -> [_ w201]
                tunnel: w189 -> [_ w200]
                tunnel: [_ w199] -> w188
                tunnel: w185 -> [w194 w198]
                tunnel: [w194 w195] -> w184
                frame False {
                }
                frame True {
                  n63 = call "myRIO_BRig_RT_comm_webdav_uploadReceived_read.vi"("input_dataSize"=w200, "input_filePath"=w201) -> ("output_Ivalid"=w199:bool, "output_data"=w197:i64[])  [unwired: 8 in]
                  n64 = To Unsigned Word Integer(number=w197) -> (unsigned 16bit integer=w196:u16[])
                  n65 = Select(t=w196, s=w199, f=w198) -> (s? t:f=w195:u16[])
                }
              }
              n66 = Select(t=myRIO_BRig_RT__Case_NonExp_stateList."UploadSettings_dataLC_1", s=w188, f=myRIO_BRig_RT__Case_NonExp_stateList."UploadSettings_Read_dataMTrig" ("t")) -> (s? t:f=w183:T1)
            }
            frame "UploadSettings_Read_dataMTrig" {
              # "grab dataMTrig and\nstore it in the\ngeneric data array"
              # "dataMTrig"
              n67 = call "myRIO_BRig_RT_dataMTrig_init_details.vi"() -> ("output_dataSize"=w208:i32, "output_dataName"=w211:string)  [unwired: 10 in]
              n68 = call "myRIO_BRig_RT_comm_webdav_uploadReceived_check.vi"("input_dataName"=w211) -> ("output_Iexist"=w210:bool, "output_dataPath"=w209:path)  [unwired: 9 in]
              n69 = case shown="True" w210 {
                tunnel: w209 -> [_ w220]
                tunnel: w208 -> [_ w219]
                tunnel: [_ w218] -> w207
                tunnel: w204 -> [w213 w217]
                tunnel: [w213 w214] -> w203
                frame False {
                }
                frame True {
                  n70 = call "myRIO_BRig_RT_comm_webdav_uploadReceived_read.vi"("input_dataSize"=w219, "input_filePath"=w220) -> ("output_Ivalid"=w218:bool, "output_data"=w216:i64[])  [unwired: 8 in]
                  n71 = To Unsigned Word Integer(number=w216) -> (unsigned 16bit integer=w215:u16[])
                  n72 = Select(t=w215, s=w218, f=w217) -> (s? t:f=w214:u16[])
                }
              }
              n73 = Select(t=myRIO_BRig_RT__Case_NonExp_stateList."UploadSettings_dataMTrig_1", s=w207, f=myRIO_BRig_RT__Case_NonExp_stateList."Idle" ("t")) -> (s? t:f=w202:T1)
            }
            frame "UploadSettings_dataExp_1" {
              w229 = 100.0 ("y")
              # "Freq"
              # "f_millisec2count"
              # "laser"
              # "Cue_max"
              # "Cue_min"
              # "CuePenalty"
              # "Timeout"
              # "Wrong"
              # "Selection"
              # "RewardPost"
              # "Reward_R"
              # "Reward_L"
              # "Tcycle"
              # "TPB_min_R"
              # "TPB_min_L"
              # "TPB_max_R"
              # "TPB_max_L"
              # "I_trialUntilReward"
              # "ENL_penalty"
              # "ENL_min"
              # "ENL_max"
              # "BUR_max"
              # "BUR_min"
              # "CueCycles"
              # "Audio_Freq_R"
              # "Audio_Freq_L"
              # "Audio_Amp_R"
              # "Audio_Amp_L"
              n74 = call "myRIO_BRig_RT_dataExp_laser_f_millisec2count.vi"() -> ("output_laser_f_millisec2count"=w243:i32)  [unwired: 11 in]
              n75 = call "myRIO_BRig_RT_dataExp_laser_Freq.vi"() -> ("output_laser_Freq"=w242:i32)  [unwired: 11 in]
              n76 = call "myRIO_BRig_RT_dataExp_CueCycles.vi"() -> ("output_CueCycles"=w289:i32)  [unwired: 11 in]
              n77 = call "myRIO_BRig_RT_dataExp_Audio_amp__R.vi"() -> ("output_Audio_amp__R"=w293:i32)  [unwired: 11 in]
              n78 = call "myRIO_BRig_RT_dataExp_Audio_amp__L.vi"() -> ("output_Audio_amp__L"=w295:i32)  [unwired: 11 in]
              n79 = call "myRIO_BRig_RT_dataExp_Tcycle_Reward__L.vi"() -> ("output_Tcycle_Reward__L"=w266:i32)  [unwired: 11 in]
              n80 = call "myRIO_BRig_RT_dataExp_Tcycle_Reward__R.vi"() -> ("output_Tcycle_Reward__R"=w265:i32)  [unwired: 11 in]
              n81 = call "myRIO_BRig_RT_dataExp_Tcycle_RewardPost.vi"() -> ("output_Tcycle_RewardPost"=w264:i32)  [unwired: 11 in]
              n82 = call "myRIO_BRig_RT_dataExp_BUR_min.vi"() -> ("output_BUR_min"=w286:i32)  [unwired: 11 in]
              n83 = call "myRIO_BRig_RT_dataExp_ENL_min.vi"() -> ("output_ENL_min"=w282:i32)  [unwired: 11 in]
              n84 = call "myRIO_BRig_RT_dataExp_TPB_max__L.vi"() -> ("output_TPB_max__L"=w274:i32)  [unwired: 11 in]
              n85 = call "myRIO_BRig_RT_dataExp_TPB_max__R.vi"() -> ("output_TPB_max__R"=w273:i32)  [unwired: 11 in]
              n86 = call "myRIO_BRig_RT_dataExp_ENL_penalty.vi"() -> ("output_ENL_penalty"=w281:i32)  [unwired: 11 in]
              n87 = call "myRIO_BRig_RT_dataExp_laser_Power_min.vi"() -> ("output_laser_Power_min"=w241:i32)  [unwired: 11 in]
              n88 = call "myRIO_BRig_RT_dataExp_laser_Tpeak.vi"() -> ("output_laser_Tpeak"=w240:i32)  [unwired: 11 in]
              n89 = call "myRIO_BRig_RT_dataExp_Audio_freq__L.vi"() -> ("output_Audio_freq__L"=w291:i32)  [unwired: 11 in]
              n90 = call "myRIO_BRig_RT_dataExp_Audio_freq__R.vi"() -> ("output_Audio_freq__R"=w290:i32)  [unwired: 11 in]
              n91 = call "myRIO_BRig_RT_dataExp_BUR_max.vi"() -> ("output_BUR_max"=w287:i32)  [unwired: 11 in]
              n92 = call "myRIO_BRig_RT_dataExp_ENL_max.vi"() -> ("output_ENL_max"=w283:i32)  [unwired: 11 in]
              n93 = call "myRIO_BRig_RT_dataExp_ItrialUntilReward.vi"() -> ("output_I_trialUntilReward"=w277:i32)  [unwired: 11 in]
              n94 = call "myRIO_BRig_RT_dataExp_Tcycle_Selection.vi"() -> ("output_Tcycle_Selection"=w263:i32)  [unwired: 11 in]
              n95 = call "myRIO_BRig_RT_dataExp_Tcycle_Wrong.vi"() -> ("output_Tcycle_Wrong"=w262:i32)  [unwired: 11 in]
              n96 = call "myRIO_BRig_RT_dataExp_Tcycle_Timeout.vi"() -> ("output_Tcycle_Timeout"=w261:i32)  [unwired: 11 in]
              n97 = call "myRIO_BRig_RT_dataExp_TPB_min__L.vi"() -> ("output_TPB_min__L"=w272:i32)  [unwired: 11 in]
              n98 = call "myRIO_BRig_RT_dataExp_TPB_min__R.vi"() -> ("output_TPB_min__R"=w271:i32)  [unwired: 11 in]
              n99 = call "myRIO_BRig_RT_dataExp_laser_Tshutter.vi"() -> ("output_laser_Tshutter"=w239:i32)  [unwired: 11 in]
              n100 = call "myRIO_BRig_RT_dataExp_laser_duration.vi"() -> ("output_laser_duration"=w238:i32)  [unwired: 11 in]
              n101 = call "myRIO_BRig_RT_dataExp_Tcycle_CuePenalty.vi"() -> ("output_Tcycle_CuePenalty"=w254:i32)  [unwired: 11 in]
              n102 = call "myRIO_BRig_RT_dataExp_Tcycle_Cue_min.vi"() -> ("output_Tcycle_Cue_min"=w253:i32)  [unwired: 11 in]
              n103 = call "myRIO_BRig_RT_dataExp_Tcycle_Cue_max.vi"() -> ("output_Tcycle_Cue_max"=w252:i32)  [unwired: 11 in]
              n104 = Index Array(array=w246, index #1=w295, index #2=w293, index #3=w291, index #4=w290, index #5=w289, index #6=w287, index #7=w286, index #8=w283, index #9=w282, index #10=w281, index #11=w277, index #12=w274, index #13=w273, index #14=w272, index #15=w271, index #16=w266, index #17=w265, index #18=w264, index #19=w263, index #20=w262, index #21=w261, index #22=w254, index #23=w253, index #24=w252, index #25=w243, index #26=w242, index #27=w241, index #28=w240, index #29=w239, index #30=w238) -> (element #1=w294:u16, element #2=w292:u16, element #3=w249:u16, element #4=w248:u16, element #5=w288:u16, element #6=w285:u16, element #7=w284:u16, element #8=w280:u16, element #9=w279:u16, element #10=w278:u16, element #11=w275:u16, element #12=w270:u16, element #13=w269:u16, element #14=w268:u16, element #15=w267:u16, element #16=w260:u16, element #17=w259:u16, element #18=w258:u16, element #19=w257:u16, element #20=w256:u16, element #21=w255:u16, element #22=w251:u16, element #23=w245:u16, element #24=w244:u16, element #25=w237:u16, element #26=w228:u16, element #27=w227:u16, element #28=w226:u16, element #29=w225:u16, element #30=w221:u16)
              n105 = To Double Precision Float(number=w237) -> (double precision float=w236:dbl)
              n106 = To Double Precision Float(number=w228) -> (double precision float=w234:dbl)
              n107 = To Double Precision Float(number=w227) -> (double precision float=w232:dbl)
              n108 = To Double Precision Float(number=w226) -> (double precision float=w231:dbl)
              n109 = To Double Precision Float(number=w225) -> (double precision float=w230:dbl)
              n110 = local write "Tcycle_Selection"(w257) -> ()
              n111 = local write "Tcycle_Wrong"(w256) -> ()
              n112 = local write "Tcycle_Timeout"(w255) -> ()
              n113 = local write "Audio_Amp__L"(w294) -> ()
              n114 = local write "Audio_Amp__R"(w292) -> ()
              n115 = Divide(x=w236, y=w229) -> (x/y=w235:dbl)
              n116 = Divide(x=w234, y=w229) -> (x/y=w233:dbl)
              n117 = Divide(x=w232, y=w229) -> (x/y=w224:dbl)
              n118 = Divide(x=w231, y=w229) -> (x/y=w223:dbl)
              n119 = Divide(x=w230, y=w229) -> (x/y=w222:dbl)
              n120 = local write "Tcycle_ENLPenalty"(w278) -> ()
              n121 = local write "Tcycle_ENL_max"(w280) -> ()
              n122 = local write "laser_duration"(w221) -> ()
              n123 = local write "TpB_Min_L"(w268) -> ()
              n124 = local write "TpB_Min_R"(w267) -> ()
              n125 = local write "laser_power_min"(w224) -> ()
              n126 = local write "f_millisec2count"(w235) -> ()
              n127 = local write "laser_Tshutter"(w222) -> ()
              n128 = local write "laser_Tpeak"(w223) -> ()
              n129 = local write "laser_Freq"(w233) -> ()
              n130 = local write "Tcycle_CuePenalty"(w251) -> ()
              n131 = local write "Tcycle_Cue_min"(w245) -> ()
              n132 = local write "Tcycle_Cue_max"(w244) -> ()
              n133 = To Unsigned Byte Integer(number=w249) -> (unsigned 8bit integer=w250:u8)
              n134 = To Unsigned Byte Integer(number=w248) -> (unsigned 8bit integer=w247:u8)
              n135 = Not Equal To 0?(x=w275) -> (x != 0?=w276:bool)
              n136 = local write "Tcycle_Reward_L"(w260) -> ()
              n137 = local write "Tcycle_Reward_R"(w259) -> ()
              n138 = local write "Tcycle_RewardPost"(w258) -> ()
              n139 = local write "CueCycles"(w288) -> ()
              n140 = local write "BUR_min"(w284) -> ()
              n141 = local write "BUR_max"(w285) -> ()
              n142 = local write "Tcycle_ENL_min"(w279) -> ()
              n143 = local write "TpB_Max_L"(w270) -> ()
              n144 = local write "TpB_Max_R"(w269) -> ()
              n145 = local write "TrialUntilReward"(w276) -> ()
              n146 = local write "Audio_Freq__L"(w250) -> ()
              n147 = local write "Audio_Freq__R"(w247) -> ()
            }
            frame "UploadSettings_dataLC_1" {
              # "Cue1_All_delayOpt"
              # "ENL1_All_delayOpt"
              # "Cue1_First_delayOpt"
              # "ENL1_First_delayOpt"
              # "ENL1 First"
              # "Cue1 All"
              # "Cue1 First"
              # "Count"
              # "Tdelay"
              # "Prob"
              # "OnOff"
              # "Block"
              # "ENL1 All"
              # "Count"
              # "Tdelay"
              # "Prob"
              # "OnOff"
              # "Block"
              # "Count"
              # "Tdelay"
              # "Prob"
              # "Block"
              # "OnOff"
              # "Count"
              # "Tdelay"
              # "Prob"
              # "OnOff"
              # "Block"
              n148 = call "myRIO_BRig_RT_dataLC_Cue1_First_Block.vi"() -> ("output_Cue1_First_Block"=w354:i32)  [unwired: 11 in]
              n149 = call "myRIO_BRig_RT_dataLC_Cue1_First_OnOff.vi"() -> ("output_Cue1_First_OnOff"=w352:i32)  [unwired: 11 in]
              n150 = call "myRIO_BRig_RT_dataLC_Cue1_First_Count.vi"() -> ("output_Cue1_First_Count"=w349:i32)  [unwired: 11 in]
              n151 = call "myRIO_BRig_RT_dataLC_Cue1_All_Block.vi"() -> ("output_Cue1_All_Block"=w336:i32)  [unwired: 11 in]
              n152 = call "myRIO_BRig_RT_dataLC_Cue1_All_OnOff.vi"() -> ("output_Cue1_All_OnOff"=w335:i32)  [unwired: 11 in]
              n153 = call "myRIO_BRig_RT_dataLC_Cue1_All_Count.vi"() -> ("output_Cue1_All_Count"=w346:i32)  [unwired: 11 in]
              n154 = call "myRIO_BRig_RT_dataLC_ENL1_First_Block.vi"() -> ("output_ENL1_First_Block"=w334:i32)  [unwired: 11 in]
              n155 = call "myRIO_BRig_RT_dataLC_ENL1_First_OnOff.vi"() -> ("output_ENL1_First_OnOff"=w345:i32)  [unwired: 11 in]
              n156 = call "myRIO_BRig_RT_dataLC_ENL1_First_Count.vi"() -> ("output_ENL1_First_Count"=w342:i32)  [unwired: 11 in]
              n157 = call "myRIO_BRig_RT_dataLC_ENL1_All_Block.vi"() -> ("output_ENL1_All_Block"=w341:i32)  [unwired: 11 in]
              n158 = call "myRIO_BRig_RT_dataLC_ENL1_All_OnOff.vi"() -> ("output_ENL1_All_OnOff"=w340:i32)  [unwired: 11 in]
              n159 = call "myRIO_BRig_RT_dataLC_ENL1_All_Count.vi"() -> ("output_ENL1_All_Count"=w337:i32)  [unwired: 11 in]
              n160 = call "myRIO_BRig_RT_dataLC_ENL1_First_delayOpt.vi"() -> ("output_ENL1_First_delayOpt"=w311:i32)  [unwired: 11 in]
              n161 = call "myRIO_BRig_RT_dataLC_Cue1_First_delayOpt.vi"() -> ("output_Cue1_First_delayOpt"=w310:i32)  [unwired: 11 in]
              n162 = call "myRIO_BRig_RT_dataLC_ENL1_All_delayOpt.vi"() -> ("output_ENL1_All_delayOpt"=w303:i32)  [unwired: 11 in]
              n163 = call "myRIO_BRig_RT_dataLC_Cue1_All_delayOpt.vi"() -> ("output_Cue1_All_delayOpt"=w302:i32)  [unwired: 11 in]
              n164 = call "myRIO_BRig_RT_dataLC_Cue1_First_Probability.vi"() -> ("output_Cue1_First_Probability"=w351:i32)  [unwired: 11 in]
              n165 = call "myRIO_BRig_RT_dataLC_Cue1_First_Tdelay.vi"() -> ("output_Cue1_First_Tdelay"=w350:i32)  [unwired: 11 in]
              n166 = call "myRIO_BRig_RT_dataLC_Cue1_All_Probability.vi"() -> ("output_Cue1_All_Probability"=w348:i32)  [unwired: 11 in]
              n167 = call "myRIO_BRig_RT_dataLC_Cue1_All_Tdelay.vi"() -> ("output_Cue1_All_Tdelay"=w347:i32)  [unwired: 11 in]
              n168 = call "myRIO_BRig_RT_dataLC_ENL1_First_Probability.vi"() -> ("output_ENL1_First_Probability"=w344:i32)  [unwired: 11 in]
              n169 = call "myRIO_BRig_RT_dataLC_ENL1_First_Tdelay.vi"() -> ("output_ENL1_First_Tdelay"=w343:i32)  [unwired: 11 in]
              n170 = call "myRIO_BRig_RT_dataLC_ENL1_All_Probability.vi"() -> ("output_ENL1_All_Probability"=w339:i32)  [unwired: 11 in]
              n171 = call "myRIO_BRig_RT_dataLC_ENL1_All_Tdelay.vi"() -> ("output_ENL1_All_Tdelay"=w338:i32)  [unwired: 11 in]
              n172 = Index Array(array=w312, index #1=w354, index #2=w352, index #3=w351, index #4=w350, index #5=w349, index #6=w336, index #7=w335, index #8=w348, index #9=w347, index #10=w346, index #11=w334, index #12=w345, index #13=w344, index #14=w343, index #15=w342, index #16=w341, index #17=w340, index #18=w339, index #19=w338, index #20=w337, index #21=w311, index #22=w310, index #23=w303, index #24=w302) -> (element #1=w353:u16, element #2=w332:u16, element #3=w331:u16, element #4=w330:u16, element #5=w329:u16, element #6=w325:u16, element #7=w324:u16, element #8=w323:u16, element #9=w322:u16, element #10=w321:u16, element #11=w320:u16, element #12=w319:u16, element #13=w318:u16, element #14=w317:u16, element #15=w304:u16, element #16=w316:u16, element #17=w315:u16, element #18=w314:u16, element #19=w313:u16, element #20=w305:u16, element #21=w308:u16, element #22=w306:u16, element #23=w299:u16, element #24=w298:u16)
              n173 = Not Equal To 0?(x=w299) -> (x != 0?=w301:bool)
              n174 = Not Equal To 0?(x=w298) -> (x != 0?=w300:bool)
              n175 = Not Equal To 0?(x=w308) -> (x != 0?=w309:bool)
              n176 = Not Equal To 0?(x=w306) -> (x != 0?=w307:bool)
              n177 = Not Equal To 0?(x=w332) -> (x != 0?=w333:bool)
              n178 = Not Equal To 0?(x=w324) -> (x != 0?=w328:bool)
              n179 = Not Equal To 0?(x=w319) -> (x != 0?=w327:bool)
              n180 = Not Equal To 0?(x=w315) -> (x != 0?=w326:bool)
              n181 = local write "LC_Cue1_First_Probability"(w331) -> ()
              n182 = local write "LC_ENL1_First_Probability"(w318) -> ()
              n183 = local write "LC_ENL1_First_delayOpt"(w309) -> ()
              n184 = local write "LC_Cue1_First_delayOpt"(w307) -> ()
              n185 = local write "LC_ENL1_All_delayOpt"(w301) -> ()
              n186 = local write "LC_Cue1_All_delayOpt"(w300) -> ()
              n187 = local write "LC_Cue1_All_Probability"(w323) -> ()
              n188 = local write "LC_Cue1_First_Tdelay"(w330) -> ()
              n189 = local write "LC_ENL1_All_Probability"(w314) -> ()
              n190 = local write "LC_Cue1_First_OnOff"(w333) -> ()
              n191 = local write "LC_Cue1_First_Count"(w329) -> ()
              n192 = local write "LC_Cue1_First_Block"(w353) -> ()
              n193 = local write "LC_ENL1_First_Tdelay"(w317) -> ()
              n194 = local write "LC_ENL1_First_OnOff"(w327) -> ()
              n195 = local write "LC_ENL1_First_Count"(w304) -> ()
              n196 = local write "LC_ENL1_First_Block"(w320) -> ()
              n197 = local write "LC_Cue1_All_Tdelay"(w322) -> ()
              n198 = local write "LC_Cue1_All_OnOff"(w328) -> ()
              n199 = local write "LC_Cue1_All_Count"(w321) -> ()
              n200 = local write "LC_Cue1_All_Block"(w325) -> ()
              n201 = local write "LC_ENL1_All_Tdelay"(w313) -> ()
              n202 = local write "LC_ENL1_All_OnOff"(w326) -> ()
              n203 = local write "LC_ENL1_All_Count"(w305) -> ()
              n204 = local write "LC_ENL1_All_Block"(w316) -> ()
            }
            frame "UploadSettings_dataLC_2" {
              # "Wrong"
              # "Reward"
              # "Trial"
              # "Tdelay"
              # "Prob"
              # "Block"
              # "OnOff"
              # "Trial"
              # "Tdelay"
              # "Prob"
              # "OnOff"
              # "Block"
              n205 = call "myRIO_BRig_RT_dataLC_Reward_Block.vi"() -> ("output_Reward_Block"=w379:i32)  [unwired: 11 in]
              n206 = call "myRIO_BRig_RT_dataLC_Reward_OnOff.vi"() -> ("output_Reward_OnOff"=w377:i32)  [unwired: 11 in]
              n207 = call "myRIO_BRig_RT_dataLC_Reward_Trial.vi"() -> ("output_Reward_Trial"=w374:i32)  [unwired: 11 in]
              n208 = call "myRIO_BRig_RT_dataLC_Wrong_Block.vi"() -> ("output_Wrong_Block"=w370:i32)  [unwired: 11 in]
              n209 = call "myRIO_BRig_RT_dataLC_Wrong_OnOff.vi"() -> ("output_Wrong_OnOff"=w369:i32)  [unwired: 11 in]
              n210 = call "myRIO_BRig_RT_dataLC_Wrong_Trial.vi"() -> ("output_Wrong_Trial"=w371:i32)  [unwired: 11 in]
              n211 = call "myRIO_BRig_RT_dataLC_Reward_Probability.vi"() -> ("output_Reward_Probability"=w376:i32)  [unwired: 11 in]
              n212 = call "myRIO_BRig_RT_dataLC_Reward_Tdelay.vi"() -> ("output_Reward_Tdelay"=w375:i32)  [unwired: 11 in]
              n213 = call "myRIO_BRig_RT_dataLC_Wrong_Probability.vi"() -> ("output_Wrong_Probability"=w373:i32)  [unwired: 11 in]
              n214 = call "myRIO_BRig_RT_dataLC_Wrong_Tdelay.vi"() -> ("output_Wrong_Tdelay"=w372:i32)  [unwired: 11 in]
              n215 = Index Array(array=w357, index #1=w379, index #2=w377, index #3=w376, index #4=w375, index #5=w374, index #6=w370, index #7=w369, index #8=w373, index #9=w372, index #10=w371) -> (element #1=w378:u16, element #2=w367:u16, element #3=w366:u16, element #4=w365:u16, element #5=w364:u16, element #6=w362:u16, element #7=w361:u16, element #8=w360:u16, element #9=w359:u16, element #10=w358:u16)
              n216 = Not Equal To 0?(x=w367) -> (x != 0?=w368:bool)
              n217 = Not Equal To 0?(x=w361) -> (x != 0?=w363:bool)
              n218 = local write "LC_Reward_Probability"(w366) -> ()
              n219 = local write "LC_Wrong_Probability"(w360) -> ()
              n220 = local write "LC_Reward_Tdelay"(w365) -> ()
              n221 = local write "LC_Reward_OnOff"(w368) -> ()
              n222 = local write "LC_Reward_Block"(w378) -> ()
              n223 = local write "LC_Reward_Trial"(w364) -> ()
              n224 = local write "LC_Wrong_Tdelay"(w359) -> ()
              n225 = local write "LC_Wrong_OnOff"(w363) -> ()
              n226 = local write "LC_Wrong_Block"(w362) -> ()
              n227 = local write "LC_Wrong_Trial"(w358) -> ()
            }
            frame "UploadSettings_dataMTrig_1" {
              # "Tdelay_R"
              # "Tdelay_L"
              # "Tcycle_R"
              # "Tcycle_L"
              # "RewCalib_nCycle_R"
              # "RewCalib_nCycle_L"
              # "Solenoid"
              # "Laser_Tcycle"
              n228 = call "myRIO_BRig_RT_dataMTrig_Laser_Tcycle.vi"() -> ("output_Laser_Tcycle"=w389:i32)  [unwired: 11 in]
              n229 = call "myRIO_BRig_RT_dataMTrig_Solenoid_RewCalib_nCycle__L.vi"() -> ("output_Solenoid_RewCalib_nCycle__L"=w388:i32)  [unwired: 11 in]
              n230 = call "myRIO_BRig_RT_dataMTrig_Solenoid_RewCalib_nCycle__R.vi"() -> ("output_Solenoid_RewCalib_nCycle__R"=w387:i32)  [unwired: 11 in]
              n231 = call "myRIO_BRig_RT_dataMTrig_Solenoid_Tdelay__L.vi"() -> ("output_Solenoid_Tdelay__L"=w384:i32)  [unwired: 11 in]
              n232 = call "myRIO_BRig_RT_dataMTrig_Solenoid_Tdelay__R.vi"() -> ("output_Solenoid_Tdelay__R"=w383:i32)  [unwired: 11 in]
              n233 = call "myRIO_BRig_RT_dataMTrig_Solenoid_Tcycle__L.vi"() -> ("output_Solenoid_Tcycle__L"=w386:i32)  [unwired: 11 in]
              n234 = call "myRIO_BRig_RT_dataMTrig_Solenoid_Tcycle__R.vi"() -> ("output_Solenoid_Tcycle__R"=w385:i32)  [unwired: 11 in]
              n235 = Index Array(array=w382, index #1=w389, index #2=w388, index #3=w387, index #4=w386, index #5=w385, index #6=w384, index #7=w383) -> (element #1=w396:u16, element #2=w395:u16, element #3=w394:u16, element #4=w393:u16, element #5=w392:u16, element #6=w391:u16, element #7=w390:u16)
              n236 = Replace Array Subset(array=w398, new element #1=w396, index #1=w389, new element #2=w395, index #2=w388, new element #3=w394, index #3=w387, new element #4=w393, index #4=w386, new element #5=w392, index #5=w385, new element #6=w391, index #6=w384, new element #7=w390, index #7=w383) -> (w397:u16[])
              n237 = local write "MTrig_Solenoid_Tcycle__L"(w393) -> ()
              n238 = local write "MTrig_Solenoid_Tcycle__R"(w392) -> ()
              n239 = local write "MTrig_Laser_Tcycle"(w396) -> ()
            }
            frame "Idle" {
              # "To ensure timing, we split the\nidle state into 4 phases"
              # "Laser_Tcycle"
              # "Audio_Tcycle_R"
              # "Audio_Tcycle_L"
              n240 = local read "laser_power_min"() -> (w401:dbl)
              n241 = local read "f_millisec2count"() -> (w409:dbl)
              n242 = local read "Audio_Amp__R"() -> (w403:u16)
              n243 = local read "Audio_Amp__L"() -> (w405:u16)
              n244 = local read "Audio_Freq__R"() -> (w402:u8)
              n245 = local read "Audio_Freq__L"() -> (w404:u8)
              n246 = local read "MTrig_Audio_trig__L"() -> (w417:bool)
              n247 = local read "MTrig_Audio_trig__R"() -> (w419:bool)
              n248 = Select(t=myRIO_BRig_RT__Case_NonExp_stateList."SendData" ("Enum"), s="SendData", f=myRIO_BRig_RT__Case_NonExp_stateList."Idle_2" ("Enum")) -> (s? t:f=w412:T1)
              n249 = call "myRIO__convert__Voltage_to_FPGAvalue.vi"("input_voltage"=w401) -> ("output_PortC"=w400:i16)  [unwired: 9 in, 1 out]
              n250 = local read "MTrig_Laser_trig"() -> (w418:bool)
              n251 = To Unsigned Word Integer(number=w409) -> (unsigned 16bit integer=w408:u16)
              n252 = call "myRIO_BRig_RT_dataMTrig_Audio_Tcycle__L.vi"() -> ("output_Audio_Tcycle__L"=w428:i32)  [unwired: 11 in]
              n253 = call "myRIO_BRig_RT_dataMTrig_Audio_Tcycle__R.vi"() -> ("output_Audio_Tcycle__R"=w427:i32)  [unwired: 11 in]
              n254 = call "myRIO_BRig_RT_dataMTrig_Laser_Tcycle.vi"() -> ("output_Laser_Tcycle"=w426:i32)  [unwired: 11 in]
              n255 = local read "MTrig_Laser_Tcycle"() -> (w410:u16)
              n256 = xnode "Read/Write Control"("FPGA VI Reference In"=w407, "error in"=w406, "k1__counter_per_ms"=w408, "audioAmp_L"=w405, "audioFreq_L_kHz"=w404, "audioAmp_R"=w403, "audioFreq_R_kHz"=w402, "AnaOut_0"=w400) -> ()  [unwired: 2 out]
              n257 = Select(t=myRIO_BRig_RT__Case_NonExp_stateList."TestConnection" ("Enum"), s="TestConnection", f=w412) -> (s? t:f=w421:T1)
              n258 = local read "Tcycle_Cue_min"() -> (w411:u16)
              n259 = Compound Arithmetic op=OR(w417, w419, w418) -> (w420:bool)
              n260 = case shown="True" w420 {
                frame False {
                }
                frame True {
                  w429 = FALSE
                  n261 = local write "MTrig_Audio_trig__L"(w429) -> ()
                  n262 = local write "MTrig_Audio_trig__R"(w429) -> ()
                  n263 = local write "MTrig_Laser_trig"(w429) -> ()
                }
              }
              n264 = Replace Array Subset(array=w424, new element #1=w411, index #1=w428, new element #2=w411, index #2=w427, new element #3=w410, index #3=w426) -> (w425:u16[])
            }
            frame "Idle_2" {
              w431 = u16 0 ("t")
              # "To ensure timing, we split the\nidle state into 4 phases"
              # "Ncycles"
              # "Ncycles"
              # "RewCalib"
              # "RewCalib"
              # "Solenoid R"
              # "Solenoid L"
              n265 = call "myRIO_BRig_RT_dataMTrig_Solenoid_RewCalib_OnOff__L.vi"() -> ("output_Solenoid_RewCalib_OnOff__L"=w462:i32)  [unwired: 11 in]
              n266 = call "myRIO_BRig_RT_dataMTrig_Solenoid_N__L.vi"() -> ("output_Solenoid_N__L"=w450:i32)  [unwired: 11 in]
              n267 = call "myRIO_BRig_RT_dataMTrig_Solenoid_RewCalib_OnOff__R.vi"() -> ("output_Solenoid_RewCalib_OnOff__R"=w447:i32)  [unwired: 11 in]
              n268 = call "myRIO_BRig_RT_dataMTrig_Solenoid_N__R.vi"() -> ("output_Solenoid_N__R"=w446:i32)  [unwired: 11 in]
              n269 = Index Array(array=w453, index #1=w462, index #2=w450, index #3=w447, index #4=w446) -> (element #1=w449:u16, element #2=w444:u16, element #3=w445:u16, element #4=w443:u16)
              n270 = local read "RewCalib_Trig_L"() -> (w442:bool)
              n271 = local read "RewCalib_Trig_R"() -> (w441:bool)
              n272 = Equal To 0?(x=w444) -> (x = 0?=w452:bool)
              n273 = Equal To 0?(x=w443) -> (x = 0?=w451:bool)
              n274 = Not Equal To 0?(x=w445) -> (x != 0?=w463:bool)
              n275 = Not Equal To 0?(x=w449) -> (x != 0?=w464:bool)
              n276 = And(x=w452, y=w451) -> (x .and. y?=w456:bool)
              n277 = Or(x=w442, y=w441) -> (x .or. y?=w457:bool)
              n278 = Not Exclusive Or(1:w464, 2:w442) -> (0:w459:bool)
              n279 = Not Exclusive Or(1:w463, 2:w441) -> (0:w461:bool)
              n280 = And(x=w457, y=w456) -> (x .and. y?=w439:bool)
              n281 = Not(x=w459) -> (.not. x?=w458:bool)
              n282 = Not(x=w461) -> (.not. x?=w460:bool)
              n283 = Or(x=w458, y=w460) -> (x .or. y?=w440:bool)
              n284 = Or(x=w439, y=w440) -> (x .or. y?=w455:bool)
              n285 = local read "count_warmup_R"() -> (w430:u16)
              n286 = local read "count_warmup_L"() -> (w435:u16)
              n287 = Select(t=myRIO_BRig_RT__Case_NonExp_stateList."RewardCalibration_pre" ("Enum"), s=w455, f=myRIO_BRig_RT__Case_NonExp_stateList."Idle_3" ("Enum")) -> (s? t:f=w438:T1)
              n288 = Select(t=w431, s="count_warmup_L_reset", f=w435) -> (s? t:f=→"count_warmup_L":u16)
              n289 = Select(t=w431, s="count_warmup_R_reset", f=w430) -> (s? t:f=→"count_warmup_R":u16)
            }
            frame "Idle_3" {
              w487 = u8 0 ("f")
              # "To ensure timing, we split the\nidle state into 4 phases"
              n290 = local read "MTrig_Solenoid_trig__L"() -> (w478:bool)
              n291 = local read "MTrig_Solenoid_trig__R"() -> (w488:bool)
              n292 = local read "warmupType"() -> (w470:u8)
              n293 = local read "warmup"() -> (w480:bool)
              n294 = Not Equal To 0?(x=w470) -> (x != 0?=w469:bool)
              n295 = Not(x=w469) -> (.not. x?=w481:bool)
              n296 = Select(t=u8 1, s=w478, f=w487) -> (s? t:f=w486:u8)
              n297 = Select(t=u8 2, s=w488, f=w487) -> (s? t:f=w485:u8)
              n298 = And(x=w480, y=w481) -> (x .and. y?=w479:bool)
              n299 = And(x=w480, y=w469) -> (x .and. y?=w474:bool)
              n300 = Add(x=w486, y=w485) -> (x+y=w484:u8)
              n301 = case shown="3" w484 {
                tunnel: w483 -> [w491 w495 w513 w531]
                tunnel: [w491 w494 w512 w530] -> w482
                tunnel: w479 -> [_ w493 w511 w529]
                tunnel: [_ TRUE TRUE TRUE] -> w476
                frame 0, Default {
                }
                frame 1 {
                  n302 = case shown="True" w493 {
                    tunnel: w495 -> [w504 w509]
                    tunnel: [w503 w508] -> w494
                    frame True {
                      # "Audio_L"
                      # "Solenoid_L"
                      n303 = call "myRIO_BRig_RT_dataMTrig_Solenoid_N__L.vi"() -> ("output_Solenoid_N__L"=w500:i32)  [unwired: 11 in]
                      n304 = call "myRIO_BRig_RT_dataMTrig_Audio_N__L.vi"() -> ("output_Audio_N__L"=w498:i32)  [unwired: 11 in]
                      n305 = Index Array(array=w504, index #1=w500, index #2=w498) -> (element #1=w502:u16, element #2=w501:u16)
                      n306 = Increment(x=w502) -> (x+1=w499:u16)
                      n307 = Increment(x=w501) -> (x+1=w497:u16)
                      n308 = Replace Array Subset(array=w504, new element #1=w499, index #1=w500, new element #2=w497, index #2=w498) -> (w503:u16[])
                    }
                    frame False {
                      # "Solenoid_L"
                      n309 = call "myRIO_BRig_RT_dataMTrig_Solenoid_N__L.vi"() -> ("output_Solenoid_N__L"=w506:i32)  [unwired: 11 in]
                      n310 = Index Array(array=w509, index=w506) -> (element=w507:u16)
                      n311 = Increment(x=w507) -> (x+1=w505:u16)
                      n312 = Replace Array Subset(array=w509, new element=w505, index=w506) -> (w508:u16[])
                    }
                  }
                  n313 = local write "MTrig_Solenoid_trig__L"(FALSE) -> ()
                }
                frame 2 {
                  n314 = case shown="True" w511 {
                    tunnel: w513 -> [w522 w527]
                    tunnel: [w521 w526] -> w512
                    frame True {
                      # "Audio_R"
                      # "Solenoid_R"
                      n315 = call "myRIO_BRig_RT_dataMTrig_Solenoid_N__R.vi"() -> ("output_Solenoid_N__R"=w518:i32)  [unwired: 11 in]
                      n316 = call "myRIO_BRig_RT_dataMTrig_Audio_N__R.vi"() -> ("output_Audio_N__R"=w517:i32)  [unwired: 11 in]
                      n317 = Index Array(array=w522, index #1=w518, index #2=w517) -> (element #1=w520:u16, element #2=w519:u16)
                      n318 = Increment(x=w519) -> (x+1=w515:u16)
                      n319 = Increment(x=w520) -> (x+1=w516:u16)
                      n320 = Replace Array Subset(array=w522, new element #1=w516, index #1=w518, new element #2=w515, index #2=w517) -> (w521:u16[])
                    }
                    frame False {
                      # "Solenoid_R"
                      n321 = call "myRIO_BRig_RT_dataMTrig_Solenoid_N__R.vi"() -> ("output_Solenoid_N__R"=w523:i32)  [unwired: 11 in]
                      n322 = Index Array(array=w527, index=w523) -> (element=w525:u16)
                      n323 = Increment(x=w525) -> (x+1=w524:u16)
                      n324 = Replace Array Subset(array=w527, new element=w524, index=w523) -> (w526:u16[])
                    }
                  }
                  n325 = local write "MTrig_Solenoid_trig__R"(FALSE) -> ()
                }
                frame 3 {
                  w532 = FALSE
                  n326 = case shown="True" w529 {
                    tunnel: w531 -> [w546 w554]
                    tunnel: [w545 w553] -> w530
                    frame True {
                      # "Audio_R"
                      # "Solenoid_R"
                      # "Audio_L"
                      # "Solenoid_L"
                      n327 = call "myRIO_BRig_RT_dataMTrig_Solenoid_N__L.vi"() -> ("output_Solenoid_N__L"=w540:i32)  [unwired: 11 in]
                      n328 = call "myRIO_BRig_RT_dataMTrig_Audio_N__L.vi"() -> ("output_Audio_N__L"=w538:i32)  [unwired: 11 in]
                      n329 = call "myRIO_BRig_RT_dataMTrig_Solenoid_N__R.vi"() -> ("output_Solenoid_N__R"=w536:i32)  [unwired: 11 in]
                      n330 = call "myRIO_BRig_RT_dataMTrig_Audio_N__R.vi"() -> ("output_Audio_N__R"=w535:i32)  [unwired: 11 in]
                      n331 = Index Array(array=w546, index #1=w540, index #2=w538, index #3=w536, index #4=w535) -> (element #1=w544:u16, element #2=w543:u16, element #3=w542:u16, element #4=w541:u16)
                      n332 = Increment(x=w541) -> (x+1=w533:u16)
                      n333 = Increment(x=w544) -> (x+1=w539:u16)
                      n334 = Increment(x=w543) -> (x+1=w537:u16)
                      n335 = Increment(x=w542) -> (x+1=w534:u16)
                      n336 = Replace Array Subset(array=w546, new element #1=w539, index #1=w540, new element #2=w537, index #2=w538, new element #3=w534, index #3=w536, new element #4=w533, index #4=w535) -> (w545:u16[])
                    }
                    frame False {
                      # "Solenoid_R"
                      # "Solenoid_L"
                      n337 = call "myRIO_BRig_RT_dataMTrig_Solenoid_N__L.vi"() -> ("output_Solenoid_N__L"=w550:i32)  [unwired: 11 in]
                      n338 = call "myRIO_BRig_RT_dataMTrig_Solenoid_N__R.vi"() -> ("output_Solenoid_N__R"=w547:i32)  [unwired: 11 in]
                      n339 = Index Array(array=w554, index #1=w550, index #2=w547) -> (element #1=w552:u16, element #2=w551:u16)
                      n340 = Increment(x=w552) -> (x+1=w549:u16)
                      n341 = Increment(x=w551) -> (x+1=w548:u16)
                      n342 = Replace Array Subset(array=w554, new element #1=w549, index #1=w550, new element #2=w548, index #2=w547) -> (w553:u16[])
                    }
                  }
                  n343 = local write "MTrig_Solenoid_trig__L"(w532) -> ()
                  n344 = local write "MTrig_Solenoid_trig__R"(w532) -> ()
                }
              }
              n345 = local read "get_countPerMS"() -> (w468:bool)
              n346 = Select(t=myRIO_BRig_RT__Case_NonExp_stateList."Get_FPGA_count_per_ms" ("Enum"), s=w468, f=myRIO_BRig_RT__Case_NonExp_stateList."Idle_4" ("Enum")) -> (s? t:f=w466:T1)
              n347 = Select(t=myRIO_BRig_RT__Case_NonExp_stateList."Cue_pre", s=w474, f=myRIO_BRig_RT__Case_NonExp_stateList."DispenseWater_pre" ("Enum")) -> (s? t:f=w472:T1)
              n348 = Select(t=w472, s=w476, f=w466) -> (s? t:f=w477:T1)
            }
            frame "Idle_4" {
              # "use dataMTrig as it is one of the last to transfer"
              # "To ensure timing, we split the\nidle state into 4 phases"
              n349 = call "myRIO_BRig_RT_comm_webdav_uploadReceived_check_v2,0.vi"("input_dataName"="dataMTrig") -> ("output_Iexist"=w560:bool)  [unwired: 9 in, 1 out]
              n350 = Select(t=myRIO_BRig_RT__Case_NonExp_stateList."UploadSettings_pre" ("Enum"), s=w560, f=myRIO_BRig_RT__Case_NonExp_stateList."Idle") -> (s? t:f=w558:T1)
            }
            frame "Cue_pre" {
              w570 = u16 1 ("t")
              w569 = u16 0 ("new element/subarray")
              w566 = u16 0 ("new element/subarray")
              # "Ncycle"
              # "count"
              # "Audio_R"
              # "Solenoid_R"
              # "Solenoid_L"
              # "Ncycle"
              # "count"
              # "Audio_L"
              n351 = call "myRIO_BRig_RT_dataMTrig_Solenoid_N__L.vi"() -> ("output_Solenoid_N__L"=w579:i32)  [unwired: 11 in]
              n352 = call "myRIO_BRig_RT_dataMTrig_Solenoid_N__R.vi"() -> ("output_Solenoid_N__R"=w578:i32)  [unwired: 11 in]
              n353 = Index Array(array=w575, index #1=w579, index #2=w578) -> (element #1=w577:u16, element #2=w576:u16)
              n354 = Not Equal To 0?(x=w576) -> (x != 0?=w562:bool)
              n355 = Not Equal To 0?(x=w577) -> (x != 0?=w563:bool)
              n356 = Select(t=w570, s=w563, f=w569) -> (s? t:f=w571:u16)
              n357 = Select(t=w570, s=w562, f=w569) -> (s? t:f=w565:u16)
              n358 = call "myRIO_BRig_RT_dataMTrig_Audio_c__L.vi"() -> ("output_Audio_c__L"=w573:i32)  [unwired: 11 in]
              n359 = call "myRIO_BRig_RT_dataMTrig_Audio_N__L.vi"() -> ("output_Audio_N__L"=w572:i32)  [unwired: 11 in]
              n360 = call "myRIO_BRig_RT_dataMTrig_Audio_c__R.vi"() -> ("output_Audio_c__R"=w568:i32)  [unwired: 11 in]
              n361 = call "myRIO_BRig_RT_dataMTrig_Audio_N__R.vi"() -> ("output_Audio_N__R"=w567:i32)  [unwired: 11 in]
              n362 = Replace Array Subset(array=w575, new element #1=w566, index #1=w573, new element #2=w571, index #2=w572, new element #3=w566, index #3=w568, new element #4=w565, index #4=w567) -> (w574:u16[])
            }
            frame "Cue" {
              # "lick did not occur or warmupType==1"
              # "lick occurred?"
              # "Ncycle"
              # "Audio_R"
              # "Ncycle"
              # "Audio_L"
              n363 = local read "warmupType"() -> (w589:u8)
              n364 = Greater?(x=w595, y=w594) -> (0:w598:bool)
              n365 = Greater?(x=w597, y=w596) -> (0:w593:bool)
              n366 = Or(x=w593, y=w598) -> (x .or. y?=w587:bool)
              n367 = Equal?(x=w589, y=u8 1) -> (x = y?=w583:bool)
              n368 = Not(x=w587) -> (.not. x?=w586:bool)
              n369 = call "myRIO_BRig_RT_dataMTrig_Audio_N__L.vi"() -> ("output_Audio_N__L"=w601:i32)  [unwired: 11 in]
              n370 = call "myRIO_BRig_RT_dataMTrig_Audio_N__R.vi"() -> ("output_Audio_N__R"=w600:i32)  [unwired: 11 in]
              n371 = Or(x=w586, y=w583) -> (x .or. y?=w584:bool)
              n372 = case shown="True" w584 {
                tunnel: w601 -> [w607 w625]
                tunnel: w600 -> [w606 w624]
                tunnel: w592 -> [w609 w619]
                tunnel: [w608 w619] -> w591
                tunnel: w590 -> [_ w617]
                tunnel: [myRIO_BRig_RT__Case_NonExp_stateList."Idle" ("t") w616] -> w585
                tunnel: w583 -> [_ w615]
                tunnel: w582 -> [_ w611]
                tunnel: w581 -> [_ w610]
                frame False {
                  w602 = u16 0 ("new element/subarray")
                  # "lick occurred and warmupType==2"
                  n373 = call "myRIO_BRig_RT_dataMTrig_Solenoid_N__R.vi"() -> ("output_Solenoid_N__R"=w603:i32)  [unwired: 11 in]
                  n374 = call "myRIO_BRig_RT_dataMTrig_Solenoid_N__L.vi"() -> ("output_Solenoid_N__L"=w604:i32)  [unwired: 11 in]
                  n375 = Replace Array Subset(array=w609, new element #1=w602, index #1=w607, new element #2=w602, index #2=w606, new element #3=w602, index #3=w604, new element #4=w602, index #4=w603) -> (w608:u16[])
                }
                frame True {
                  n376 = Not(x=w615) -> (.not. x?=w614:bool)
                  n377 = Index Array(array=w619, index #1=w625, index #2=w624) -> (element #1=w623:u16, element #2=w622:u16)
                  n378 = Equal To 0?(x=w623) -> (x = 0?=w621:bool)
                  n379 = Equal To 0?(x=w622) -> (x = 0?=w620:bool)
                  n380 = And(x=w621, y=w620) -> (x .and. y?=w613:bool)
                  n381 = And(x=w613, y=w614) -> (x .and. y?=w612:bool)
                  n382 = case shown="True" w612 {
                    tunnel: w611 -> [_ w633]
                    tunnel: w610 -> [_ w628]
                    frame False {
                    }
                    frame True {
                      n383 = local read "count_warmup_R"() -> (w626:u16)
                      n384 = local read "count_warmup_L"() -> (w631:u16)
                      n385 = Increment(x=w626) -> (x+1=w629:u16)
                      n386 = Increment(x=w631) -> (x+1=w632:u16)
                      n387 = Select(t=w629, s=w628, f=w626) -> (s? t:f=w627:u16)
                      n388 = Select(t=w632, s=w633, f=w631) -> (s? t:f=w630:u16)
                      n389 = local write "count_warmup_R"(w627) -> ()
                      n390 = local write "count_warmup_L"(w630) -> ()
                    }
                  }
                  n391 = Select(t=myRIO_BRig_RT__Case_NonExp_stateList."DispenseWater_pre", s=w613, f=w617) -> (s? t:f=w616:T1)
                }
              }
            }
            frame "RewardCalibration_pre" {
              (unwired) FALSE
              w635 = FALSE
              w646 = u8 0
              w662 = u8 0
              # "Are we starting a RewardCalibration?\nOr are we stopping a RewardCalibration?\nOr is a RewardCalibration over?"
              # "RewCalib\nOnOff"
              # "N"
              # "Solenoid R"
              # "RewCalib\nOnOff"
              # "N"
              # "Solenoid L"
              n392 = local read "RewCalib_Trig_L"() -> (w669:bool)
              n393 = local read "RewCalib_Trig_R"() -> (w638:bool)
              n394 = call "myRIO_BRig_RT_dataMTrig_Solenoid_N__R.vi"() -> ("output_Solenoid_N__R"=w640:i32)  [unwired: 11 in]
              n395 = call "myRIO_BRig_RT_dataMTrig_Solenoid_RewCalib_OnOff__R.vi"() -> ("output_Solenoid_RewCalib_OnOff__R"=w637:i32)  [unwired: 11 in]
              n396 = call "myRIO_BRig_RT_dataMTrig_Solenoid_N__L.vi"() -> ("output_Solenoid_N__L"=w655:i32)  [unwired: 11 in]
              n397 = call "myRIO_BRig_RT_dataMTrig_Solenoid_RewCalib_OnOff__L.vi"() -> ("output_Solenoid_RewCalib_OnOff__L"=w656:i32)  [unwired: 11 in]
              n398 = Index Array(array=w639, index #1=w640, index #2=w637) -> (element #1=w650:u16, element #2=w645:u16)
              n399 = Index Array(array=w639, index #1=w655, index #2=w656) -> (element #1=w666:u16, element #2=w661:u16)
              n400 = Equal To 0?(x=w650) -> (x = 0?=w651:bool)
              n401 = Not Equal To 0?(x=w645) -> (x != 0?=w648:bool)
              n402 = Equal To 0?(x=w666) -> (x = 0?=w667:bool)
              n403 = Not Equal To 0?(x=w661) -> (x != 0?=w664:bool)
              n404 = local write "MTrig_Solenoid_trig__L"(w635) -> ()
              n405 = local write "MTrig_Solenoid_trig__R"(w635) -> ()
              n406 = Select(t=u8 1, s=w638, f=w646) -> (s? t:f=w642:u8)
              n407 = Select(t=u8 1, s=w669, f=w662) -> (s? t:f=w658:u8)
              n408 = Select(t=u8 2, s=w651, f=w646) -> (s? t:f=w643:u8)
              n409 = Select(t=u8 4, s=w648, f=w646) -> (s? t:f=w644:u8)
              n410 = Select(t=u8 2, s=w667, f=w662) -> (s? t:f=w659:u8)
              n411 = Select(t=u8 4, s=w664, f=w662) -> (s? t:f=w660:u8)
              n412 = Compound Arithmetic op=ADD(w642, w643, w644) -> (w641:u8)
              n413 = Compound Arithmetic op=ADD(w658, w659, w660) -> (w657:u8)
              n414 = case shown="7" w657 {
                tunnel: w639 -> [w699 w704 w706 w711 w716 w718 w721 w726]
                tunnel: [w699 w705 w706 w712 w717 w718 w722 w727] -> w654
                tunnel: w656 -> [_ w702 _ w709 w714 _ w720 w725]
                tunnel: w655 -> [_ w703 _ w710 w715 _ _ _]
                frame 0, Default {
                }
                frame 1 {
                  n415 = Replace Array Subset(array=w704, new element #1=u16 100 ("new element/subarray"), index #1=w703, new element #2=u16 1 ("new element/subarray"), index #2=w702) -> (w705:u16[])
                }
                frame 2 {
                }
                frame 3 {
                  n416 = Replace Array Subset(array=w711, new element #1=u16 100 ("new element/subarray"), index #1=w710, new element #2=u16 1 ("new element/subarray"), index #2=w709) -> (w712:u16[])
                }
                frame 4 {
                  w713 = u16 0 ("new element/subarray")
                  n417 = Replace Array Subset(array=w716, new element #1=w713, index #1=w715, new element #2=w713, index #2=w714) -> (w717:u16[])
                }
                frame 5 {
                }
                frame 6 {
                  n418 = Replace Array Subset(array=w721, new element=u16 0 ("new element/subarray"), index=w720) -> (w722:u16[])
                }
                frame 7 {
                  n419 = local write "RewCalib_Trig_L"(FALSE ("RewCalib_Trig_L")) -> ()
                  n420 = Replace Array Subset(array=w726, new element=u16 0 ("new element/subarray"), index=w725) -> (w727:u16[])
                }
              }
              n421 = case shown="7" w641 {
                tunnel: w654 -> [w670 w675 w677 w682 w687 w689 w692 w697]
                tunnel: [w670 w676 w677 w683 w688 w689 w693 w698] -> w653
                tunnel: w637 -> [_ w673 _ w680 w685 _ w691 w696]
                tunnel: w640 -> [_ w674 _ w681 w686 _ _ _]
                frame 0, Default {
                }
                frame 1 {
                  n422 = Replace Array Subset(array=w675, new element #1=u16 100 ("new element/subarray"), index #1=w674, new element #2=u16 1 ("new element/subarray"), index #2=w673) -> (w676:u16[])
                }
                frame 2 {
                }
                frame 3 {
                  n423 = Replace Array Subset(array=w682, new element #1=u16 100 ("new element/subarray"), index #1=w681, new element #2=u16 1 ("new element/subarray"), index #2=w680) -> (w683:u16[])
                }
                frame 4 {
                  w684 = u16 0 ("new element/subarray")
                  n424 = Replace Array Subset(array=w687, new element #1=w684, index #1=w686, new element #2=w684, index #2=w685) -> (w688:u16[])
                }
                frame 5 {
                }
                frame 6 {
                  n425 = Replace Array Subset(array=w692, new element=u16 0 ("new element/subarray"), index=w691) -> (w693:u16[])
                }
                frame 7 {
                  n426 = local write "RewCalib_Trig_R"(FALSE ("RewCalib_Trig_L")) -> ()
                  n427 = Replace Array Subset(array=w697, new element=u16 0 ("new element/subarray"), index=w696) -> (w698:u16[])
                }
              }
            }
            frame "DispenseWater_pre" {
              w734 = u16 0 ("t")
              w777 = u16 0 ("new element/subarray")
              # "just trust me on this one"
              # "RewCalib\nOnOff"
              # "RewCalib\nOnOff"
              # "nCycle"
              # "Solenoid__R"
              # "Tdelay"
              # "delay"
              # "nCycle"
              # "Solenoid__L"
              # "Tdelay"
              # "delay"
              # "Solenoid__R"
              # "count"
              # "Solenoid_Tcycle_R"
              # "Solenoid_Tcycle_L"
              # "Solenoid__L"
              # "count"
              n428 = call "myRIO_BRig_RT_dataMTrig_Solenoid_RewCalib_OnOff__L.vi"() -> ("output_Solenoid_RewCalib_OnOff__L"=w741:i32)  [unwired: 11 in]
              n429 = call "myRIO_BRig_RT_dataMTrig_Solenoid_N__L.vi"() -> ("output_Solenoid_N__L"=w732:i32)  [unwired: 11 in]
              n430 = call "myRIO_BRig_RT_dataMTrig_Solenoid_delay__L.vi"() -> ("output_Solenoid_delay__L"=w775:i32)  [unwired: 11 in]
              n431 = call "myRIO_BRig_RT_dataMTrig_Solenoid_Tdelay__L.vi"() -> ("output_Solenoid_Tdelay__L"=w774:i32)  [unwired: 11 in]
              n432 = call "myRIO_BRig_RT_dataMTrig_Solenoid_N__R.vi"() -> ("output_Solenoid_N__R"=w730:i32)  [unwired: 11 in]
              n433 = call "myRIO_BRig_RT_dataMTrig_Solenoid_delay__R.vi"() -> ("output_Solenoid_delay__R"=w764:i32)  [unwired: 11 in]
              n434 = call "myRIO_BRig_RT_dataMTrig_Solenoid_Tdelay__R.vi"() -> ("output_Solenoid_Tdelay__R"=w763:i32)  [unwired: 11 in]
              n435 = call "myRIO_BRig_RT_dataMTrig_Solenoid_RewCalib_OnOff__R.vi"() -> ("output_Solenoid_RewCalib_OnOff__R"=w737:i32)  [unwired: 11 in]
              n436 = Index Array(array=w776, index #1=w732, index #2=w775, index #3=w774, index #4=w730, index #5=w764, index #6=w763, index #7=w741, index #8=w737) -> (element #1=w733:u16, element #2=w773:u16, element #3=w768:u16, element #4=w736:u16, element #5=w758:u16, element #6=w757:u16, element #7=w742:u16, element #8=w739:u16)
              n437 = Equal To 0?(x=w773) -> (x = 0?=w772:bool)
              n438 = Equal To 0?(x=w758) -> (x = 0?=w762:bool)
              n439 = local read "RewCalib_Trig_L"() -> (w753:bool)
              n440 = local read "RewCalib_Trig_R"() -> (w748:bool)
              n441 = Not Equal To 0?(x=w733) -> (x != 0?=w771:bool)
              n442 = Not Equal To 0?(x=w736) -> (x != 0?=w761:bool)
              n443 = local read "MTrig_Solenoid_Tcycle__L"() -> (w770:u16)
              n444 = local read "MTrig_Solenoid_Tcycle__R"() -> (w756:u16)
              n445 = Not Equal To 0?(x=w742) -> (x != 0?=w752:bool)
              n446 = Not Equal To 0?(x=w739) -> (x != 0?=w750:bool)
              n447 = Not(x=w753) -> (.not. x?=w751:bool)
              n448 = Not(x=w748) -> (.not. x?=w749:bool)
              n449 = And(x=w752, y=w751) -> (x .and. y?=w747:bool)
              n450 = And(x=w750, y=w749) -> (x .and. y?=w746:bool)
              n451 = call "myRIO_BRig_RT_dataMTrig_Solenoid_c__L.vi"() -> ("output_Solenoid_c__L"=w779:i32)  [unwired: 11 in]
              n452 = call "myRIO_BRig_RT_dataMTrig_Solenoid_c__R.vi"() -> ("output_Solenoid_c__R"=w778:i32)  [unwired: 11 in]
              n453 = Select(t=w770, s=w771, f=u16 0) -> (s? t:f=w767:u16)
              n454 = Or(x=w747, y=w746) -> (x .or. y?=w735:bool)
              n455 = Select(t=w756, s=w761, f=u16 0) -> (s? t:f=w759:u16)
              n456 = Select(t=w767, s=w772, f=w768) -> (s? t:f=w765:u16)
              n457 = Select(t=w759, s=w762, f=w757) -> (s? t:f=w754:u16)
              n458 = call "myRIO_BRig_RT_dataMTrig_Solenoid_Tcycle__L.vi"() -> ("output_Solenoid_Tcycle__L"=w766:i32)  [unwired: 11 in]
              n459 = call "myRIO_BRig_RT_dataMTrig_Solenoid_Tcycle__R.vi"() -> ("output_Solenoid_Tcycle__R"=w755:i32)  [unwired: 11 in]
              n460 = Select(t=w734, s=w735, f=w733) -> (s? t:f=w731:u16)
              n461 = Select(t=w734, s=w735, f=w736) -> (s? t:f=w729:u16)
              n462 = Select(t=myRIO_BRig_RT__Case_NonExp_stateList."Idle" ("Enum"), s=w735, f=myRIO_BRig_RT__Case_NonExp_stateList."DispenseWater" ("Enum")) -> (s? t:f=w743:T1)
              n463 = Select(t=w734, s=w735, f=w742) -> (s? t:f=w740:u16)
              n464 = Select(t=w734, s=w735, f=w739) -> (s? t:f=w738:u16)
              n465 = Replace Array Subset(array=w776, new element #1=w777, index #1=w779, new element #2=w777, index #2=w778, new element #3=w765, index #3=w766, new element #4=w754, index #4=w755, new element #5=w740, index #5=w741, new element #6=w738, index #6=w737, new element #7=w731, index #7=w732, new element #8=w729, index #8=w730) -> (w780:u16[])
            }
            frame "DispenseWater" {
              # "D"
              # "C"
              # "B"
              # "A"
              # "(A) Add COUNT and INCREMENT\n(B) Is (A) smaller than Tcycle?\n(C) Are we dispensing water or in the delay phase?\n(D) If (A) is smaller than Tcycle   AND   if we are dispensing water\n      then send TRUE to solenoid"
              # "delay"
              # "Tcycle"
              # "Solenoid__R"
              # "count"
              # "delay"
              # "Tcycle"
              # "Solenoid__L"
              # "count"
              n466 = To Unsigned Word Integer(number=w808) -> (unsigned 16bit integer=w790:u16)
              n467 = call "myRIO_BRig_RT_dataMTrig_Solenoid_delay__R.vi"() -> ("output_Solenoid_delay__R"=w794:i32)  [unwired: 11 in]
              n468 = call "myRIO_BRig_RT_dataMTrig_Solenoid_c__R.vi"() -> ("output_Solenoid_c__R"=w793:i32)  [unwired: 11 in]
              n469 = call "myRIO_BRig_RT_dataMTrig_Solenoid_Tcycle__R.vi"() -> ("output_Solenoid_Tcycle__R"=w795:i32)  [unwired: 11 in]
              n470 = call "myRIO_BRig_RT_dataMTrig_Solenoid_delay__L.vi"() -> ("output_Solenoid_delay__L"=w810:i32)  [unwired: 11 in]
              n471 = call "myRIO_BRig_RT_dataMTrig_Solenoid_c__L.vi"() -> ("output_Solenoid_c__L"=w802:i32)  [unwired: 11 in]
              n472 = call "myRIO_BRig_RT_dataMTrig_Solenoid_Tcycle__L.vi"() -> ("output_Solenoid_Tcycle__L"=w811:i32)  [unwired: 11 in]
              n473 = Index Array(array=w804, index #1=w802, index #2=w811, index #3=w810, index #4=w793, index #5=w795, index #6=w794) -> (element #1=w809:u16, element #2=w799:u16, element #3=w807:u16, element #4=w789:u16, element #5=w786:u16, element #6=w785:u16)
              n474 = Add(x=w809, y=w790) -> (x+y=w800:u16)
              n475 = Add(x=w789, y=w790) -> (x+y=w791:u16)
              n476 = Less?(x=w800, y=w799) -> (x < y?=w783:bool)
              n477 = Equal To 0?(x=w807) -> (x = 0?=w806:bool)
              n478 = Less?(x=w791, y=w786) -> (x < y?=w784:bool)
              n479 = Equal To 0?(x=w785) -> (x = 0?=w792:bool)
              n480 = And(x=w783, y=w806) -> (x .and. y?=w805:bool)
              n481 = Or(x=w783, y=w784) -> (x .or. y?=w782:bool)
              n482 = And(x=w784, y=w792) -> (x .and. y?=w787:bool)
              n483 = Select(t=w800, s=w783, f=w799) -> (s? t:f=w801:u16)
              n484 = Select(t=w791, s=w784, f=w786) -> (s? t:f=w788:u16)
              n485 = Replace Array Subset(array=w804, new element #1=w801, index #1=w802, new element #2=w788, index #2=w793) -> (w803:u16[])
              n486 = Select(t=w798, s=w782, f=myRIO_BRig_RT__Case_NonExp_stateList."DispenseWater_post" ("Enum")) -> (s? t:f=w796:T1)
            }
            frame "DispenseWater_post" {
              # "nCycle"
              # "delay"
              # "Solenoid__R"
              # "nCycle"
              # "delay"
              # "Solenoid__L"
              n487 = call "myRIO_BRig_RT_dataMTrig_Solenoid_N__L.vi"() -> ("output_Solenoid_N__L"=w829:i32)  [unwired: 11 in]
              n488 = call "myRIO_BRig_RT_dataMTrig_Solenoid_delay__L.vi"() -> ("output_Solenoid_delay__L"=w828:i32)  [unwired: 11 in]
              n489 = call "myRIO_BRig_RT_dataMTrig_Solenoid_N__R.vi"() -> ("output_Solenoid_N__R"=w825:i32)  [unwired: 11 in]
              n490 = call "myRIO_BRig_RT_dataMTrig_Solenoid_delay__R.vi"() -> ("output_Solenoid_delay__R"=w824:i32)  [unwired: 11 in]
              n491 = Index Array(array=w831, index #1=w829, index #2=w828, index #3=w825, index #4=w824) -> (element #1=w833:u16, element #2=w832:u16, element #3=w816:u16, element #4=w818:u16)
              n492 = Not Equal To 0?(x=w833) -> (x != 0?=w834:bool)
              n493 = Not Equal To 0?(x=w816) -> (x != 0?=w817:bool)
              n494 = case shown="True" w817 {
                selector: w817 -> [_ w838]
                tunnel: w816 -> [w836 w844]
                tunnel: w818 -> [_ w845]
                tunnel: [w836 w842] -> w815
                tunnel: [u16 0 w841] -> w814
                tunnel: [_ w838] -> w813
                frame False {
                }
                frame True {
                  n495 = Equal To 0?(x=w845) -> (x = 0?=w837:bool)
                  n496 = Decrement(x=w844) -> (x-1=w843:u16)
                  n497 = Select(t=w843, s=w837, f=w844) -> (s? t:f=w842:u16)
                  n498 = Select(t=u16 1, s=w837, f=u16 0) -> (s? t:f=w841:u16)
                }
              }
              n499 = case shown="True" w834 {
                selector: w834 -> [_ w849]
                tunnel: w833 -> [w847 w855]
                tunnel: w832 -> [_ w856]
                tunnel: [w847 w853] -> w827
                tunnel: [u16 0 w852] -> w826
                tunnel: [_ w849] -> w823
                frame False {
                }
                frame True {
                  n500 = Equal To 0?(x=w856) -> (x = 0?=w848:bool)
                  n501 = Decrement(x=w855) -> (x-1=w854:u16)
                  n502 = Select(t=w854, s=w848, f=w855) -> (s? t:f=w853:u16)
                  n503 = Select(t=u16 1, s=w848, f=u16 0) -> (s? t:f=w852:u16)
                }
              }
              n504 = Or(x=w823, y=w813) -> (x .or. y?=w822:bool)
              n505 = Replace Array Subset(array=w831, new element #1=w827, index #1=w829, new element #2=w826, index #2=w828, new element #3=w815, index #3=w825, new element #4=w814, index #4=w824) -> (w830:u16[])
              n506 = Select(t=myRIO_BRig_RT__Case_NonExp_stateList."DispenseWater_pre" ("Enum"), s=w822, f=myRIO_BRig_RT__Case_NonExp_stateList."Idle" ("Enum")) -> (s? t:f=w819:T1)
            }
            frame "TestConnection" {
              n507 = local read "Host Password"() -> (w863:string)
              n508 = local read "Host UserName"() -> (w864:string)
              n509 = call "myRIO_BRig_RT_comm_webdav_testConnect.vi"("input_password"=w863, "input_username"=w864) -> ("output_Iconnected"=w861:bool)  [unwired: 9 in]
              n510 = Select(t="Connection accepted!" ("message"), s=w861, f="Error!") -> (s? t:f=w859:string)
              n511 = One Button Dialog(message=w859) -> ()  [unwired: 1 in, 1 out]
            }
            frame "SendData" {
              n512 = local read "Data Set Prefix"() -> (w866:string)
              n513 = local read "Host Password"() -> (w867:string)
              n514 = local read "Host UserName"() -> (w868:string)
              n515 = call "myRIO_BRig_RT_comm_webdav_sendData_all.vi"("Host Filename Prefix"=w866, "Host Password"=w867, "Host UserName"=w868) -> ()  [unwired: 9 in]
            }
            frame "Get_FPGA_count_per_ms" {
              n516 = case shown="False" w882 {
                selector: w882 -> [w885 _]
                tunnel: w880 -> [_ w898]
                tunnel: [w889 w898] -> w879
                tunnel: w878 -> [w888 w896]
                tunnel: w877 -> [w887 w895]
                tunnel: [w886 w893] -> w876
                tunnel: [w885 w892] -> w875
                frame False {
                  n517 = Get Date/Time In Seconds() -> (seconds since 1Jan1904=w890:timestamp)
                  n518 = xnode "Read/Write Control"("FPGA VI Reference In"=w888, "error in"=w887, "timeTrial"=TRUE) -> ("error out"=w886:errorcluster)  [unwired: 1 out]
                  n519 = To Double Precision Float(number=w890) -> (double precision float=w889:dbl)
                  n520 = local write "get_countPerMS"(w885) -> ()
                }
                frame True {
                  w894 = 1.0
                  n521 = Get Date/Time In Seconds() -> (seconds since 1Jan1904=w899:timestamp)
                  n522 = To Double Precision Float(number=w899) -> (double precision float=w900:dbl)
                  n523 = Subtract(x=w900, y=w898) -> (x-y=w897:dbl)
                  n524 = Less Or Equal?(x=w894, y=w897) -> (x <= y?=w892:bool)
                  n525 = case shown="True" w892 {
                    tunnel: w896 -> [_ w913]
                    tunnel: w895 -> [w901 w912]
                    tunnel: w894 -> [_ w903]
                    tunnel: [w901 w902] -> w893
                    frame False {
                    }
                    frame True {
                      n526 = xnode "Read/Write Control"("FPGA VI Reference In"=w913, "error in"=w912) -> ("FPGA VI Reference Out"=w910:refnum<k20>, "error out"=w909:errorcluster, "count_timeTrial"=w904:u32)
                      n527 = Multiply(x=w903, y=1000.0) -> (x*y=w907:dbl)
                      n528 = To Double Precision Float(number=w904) -> (double precision float=w906:dbl)
                      n529 = Divide(x=w906, y=w907) -> (x/y=w908:dbl)
                      n530 = local write "f_millisec2count"(w908) -> ()
                      n531 = xnode "Read/Write Control"("FPGA VI Reference In"=w910, "error in"=w909, "timeTrial"=FALSE) -> ("error out"=w902:errorcluster)  [unwired: 1 out]
                    }
                  }
                }
              }
              "error out 5" <- w876
              n532 = Select(t=myRIO_BRig_RT__Case_NonExp_stateList."Idle" ("Enum"), s=w875, f=w873) -> (s? t:f=w872:T1)
            }
            frame "End" {
            }
          }
          n533 = local read "MTrig_Audio_trig__R"() -> (w119:bool)
          n534 = local read "MTrig_Audio_trig__L"() -> (w118:bool)
          n535 = local read "START"() -> (w114:bool)
          n536 = local read "STOP_abort"() -> (w113:bool)
          n537 = local read "MTrig_Laser_trig"() -> (w120:bool)
          n538 = call "myRIO_BRig_RT_dataMTrig_main__v2.vi"("input_dataMTrig"=w122, "input_Audio_trig_L"=w118, "input_Audio_trig_R"=w119, "input_Laser_trig"=w120) -> ("output_dataMTrig"=w121:u16[], "output_Audio_L"=w98:bool, "output_Audio_R"=w109:bool, "output_Laser"=w101:bool)  [unwired: 12 in]
          n539 = Or(x=w114, y=w113) -> (x .or. y?=w112:bool)
          n540 = Select(t=myRIO_BRig_RT__Case_NonExp_stateList."End" ("Enum"), s=w112, f=w111) -> (s? t:f=w110:T1)
          n541 = Or(x=w119, y=w120) -> (x .or. y?=w117:bool)
          n542 = Or(x=w117, y=w118) -> (x .or. y?=w116:bool)
          n543 = case shown="True" w116 {
            frame False {
            }
            frame True {
              w135 = FALSE
              n544 = local write "MTrig_Audio_trig__R"(w135) -> ()
              n545 = local write "MTrig_Audio_trig__L"(w135) -> ()
              n546 = local write "MTrig_Laser_trig"(w135) -> ()
            }
          }
          n547 = xnode "Read/Write Control"("FPGA VI Reference In"=w87, "error in"=w86, "A1_SR"=w123, "A3_SL"=w124, "audioTrigger_L"=w98, "audioTrigger_R"=w109, "laserResponse_reward_LED"="laserResponse_reward_LED", "laserResponse_wrong_LED"="laserResponse_wrong_LED", "laserResponse_reward"="laserResponse_reward", "laserResponse_wrong"="laserResponse_wrong", "SelectionState"="SelectionState", "ignoreWrong"="ignoreWrong", "Left(F)_or_Right(T)"="Left(F)_or_Right(T)", "laserMTrig"=w101) -> ("FPGA VI Reference Out"=w129:refnum<k20>, "error out"=w128:errorcluster, "SelectReward"=→"SelectReward":bool, "SelectWrong"=→"SelectWrong":bool, "AnaIn_0"=→"tempAI0":i16)
          n548 = node-c288() -> ()  [unwired: 1 in, 1 out]
          "cState_NonExp" <- w127
        }
        n549 = node-c288(w69) -> ()  [unwired: 1 out]
        n550 = flat-sequence {
          tunnel: w62 -> [w80]
          tunnel: [w80] -> w61
          tunnel: w60 -> [w79]
          tunnel: [w79] -> w59
          frame #0 {
            w78 = FALSE
            n551 = local write "STOP_endBlock"(w78) -> ()
            n552 = local write "STOP_endTrial"(w78) -> ()
          }
        }
      }
      frame True {
        w935 = u16 0
        w938 = u8 0
        w940 = FALSE ("SelectionState")
        w945 = u16 0 ("idxDataBlock")
        w947 = u16 100 ("new element/subarray")
        w948 = u16 100 ("new element/subarray")
        w968 = T6 refnum items=["Session NI_WebDAV"] ("output_hSession")
        w977 = FALSE
        w978 = u16 0
        w939 = FALSE
        # "audio__L\naudio__R"
        # "Audio params"
        # "nRewards"
        # "idxDataBlock"
        # "Solenoid_Tdelay_R"
        # "Solenoid_Tdelay_L"
        # "RewCalib_N__R"
        # "RewCalib_N__L"
        # "Save dataLick to file\nSend file to Host\nSave dataMTrig\nSend file to Host\nDisconnect"
        # "dataTrial"
        # "dataTrial"
        # "Solenoid_Tcycle_R"
        # "Solenoid_Tcycle_L"
        # "Laser_Tcycle"
        # "Audio_Tcycle_R"
        # "Audio_Tcycle_L"
        # "dataLick"
        # "dataLC"
        # "dataLC"
        # "dataBlock"
        # "dataBlock"
        # "dataMTrig"
        # "dataMTrig"
        # "dataExp"
        # "dataCurrent"
        # "dataExp"
        # "dataCurrent"
        # "spout"
        # "state"
        n553 = call "myRIO_BRig_RT_dataMTrig_Solenoid_Tcycle__L.vi"() -> ("output_Solenoid_Tcycle__L"=w974:i32)  [unwired: 11 in]
        n554 = call "myRIO_BRig_RT_dataMTrig_Solenoid_Tcycle__R.vi"() -> ("output_Solenoid_Tcycle__R"=w973:i32)  [unwired: 11 in]
        n555 = call "myRIO_BRig_RT_dataMTrig_Audio_Tcycle__L.vi"() -> ("output_Audio_Tcycle__L"=w972:i32)  [unwired: 11 in]
        n556 = call "myRIO_BRig_RT_dataMTrig_Audio_Tcycle__R.vi"() -> ("output_Audio_Tcycle__R"=w971:i32)  [unwired: 11 in]
        n557 = call "myRIO_BRig_RT_dataMTrig_Laser_Tcycle.vi"() -> ("output_Laser_Tcycle"=w970:i32)  [unwired: 11 in]
        n558 = local read "MTrig_Solenoid_Tcycle__L"() -> (w953:u16)
        n559 = local read "MTrig_Solenoid_Tcycle__R"() -> (w952:u16)
        n560 = local read "Tcycle_Reward_L"() -> (w949:u16)
        n561 = local read "Tcycle_Reward_R"() -> (w950:u16)
        n562 = local read "MTrig_Laser_Tcycle"() -> (w951:u16)
        n563 = call "myRIO_BRig_RT_dataMTrig_Solenoid_RewCalib_nCycle__L.vi"() -> ("output_Solenoid_RewCalib_nCycle__L"=w956:i32)  [unwired: 11 in]
        n564 = call "myRIO_BRig_RT_dataMTrig_Solenoid_Tdelay__L.vi"() -> ("output_Solenoid_Tdelay__L"=w958:i32)  [unwired: 11 in]
        n565 = call "myRIO_BRig_RT_dataMTrig_Solenoid_RewCalib_nCycle__R.vi"() -> ("output_Solenoid_RewCalib_nCycle__R"=w957:i32)  [unwired: 11 in]
        n566 = call "myRIO_BRig_RT_dataMTrig_Solenoid_Tdelay__R.vi"() -> ("output_Solenoid_Tdelay__R"=w959:i32)  [unwired: 11 in]
        n567 = case shown="False" w929 {
          selector: w929 -> [_ w1000]
          tunnel: w928 -> [w997 w1002]
          tunnel: [w998 w1002] -> w927
          tunnel: w926 -> [_ w1001]
          tunnel: [w999 w1001] -> w925
          tunnel: [w996 w1000] -> w923
          frame False {
            n568 = call "myRIO__TCP_connect_forWriting.vi"("input_error"=w997) -> ("output_error"=w998:errorcluster, "output_connected"=w996:bool, "output_hTCP"=w999:refnum<k5>)  [unwired: 8 in]
          }
          frame True {
          }
        }
        n569 = call "myRIO_BRig_RT_dataLick_init.vi"() -> ("output_dataLick"=w980:u16[][])  [unwired: 11 in]
        n570 = call "myRIO_BRig_RT_dataCurrent_init.vi"() -> ("output_dataCurrent"=w987:u16[])  [unwired: 11 in]
        n571 = call "myRIO_BRig_RT_dataExp_init.vi"() -> ("output_dataExp"=w986:u16[])  [unwired: 11 in]
        n572 = call "myRIO_BRig_RT_dataMTrig_init.vi"() -> ("output_dataMTrig"=w976:u16[])  [unwired: 5 in]
        n573 = call "myRIO_BRig_RT_dataLC_init.vi"() -> ("output_dataLC"=w984:u16[])  [unwired: 11 in]
        n574 = call "myRIO_BRig_RT_dataBlock_init.vi"() -> ("output_dataBlock"=w985:u16[][])  [unwired: 11 in]
        n575 = call "myRIO_BRig_RT_dataTrial_init.vi"() -> ("output_dataTrial"=w969:u16[][])  [unwired: 11 in]
        n576 = xnode "Read/Write Control"("FPGA VI Reference In"=w941, "error in"=w942, "SelectionState"=w940, "laserResponse_reward"=w940, "laserResponse_wrong"=w940, "laserResponse_reward_LED"=w940, "laserResponse_wrong_LED"=w940, "Left(F)_or_Right(T)"=w940, "ignoreWrong"=w940, "SelectionState"=w940) -> ("FPGA VI Reference Out"=w943:refnum<k20>, "error out"=w944:errorcluster)
        n577 = local write "I_connect_TCP"(w923) -> ()
        n578 = Replace Array Subset(array=w976, new element #1=w948, index #1=w956, new element #2=w948, index #2=w957, new element #3=w947, index #3=w958, new element #4=w947, index #4=w959, new element #5=w953, index #5=w974, new element #6=w952, index #6=w973, new element #7=w949, index #7=w972, new element #8=w950, index #8=w971, new element #9=w951, index #9=w970) -> (w975:u16[])
        n579 = call "myRIO_BRig_RT_dataAnalog_init.vi"() -> ("output_dataAnalog"=w934:u16[][])  [unwired: 11 in]
        n580 = Get Date/Time In Seconds() -> (seconds since 1Jan1904=w955:timestamp)
        n581 = To Double Precision Float(number=w955) -> (double precision float=w954:dbl)
        n582 = node-c288() -> (w995:T3)  [unwired: 4 in]
        n583 = timed-loop {
          timing: w995 -> [_]
          timing-out: [_] -> w994
          shift-right: [w1113] -> _
          shift-left: myRIO_BRig_RT__Case_Exp_stateList."Start1" ("Enum") -> [w1046]
          shift-right: [w1164] -> _
          shift-left: enum16{"Left", "Right"}."Left" -> [w1166]
          tunnel: w943 -> [w1163]
          tunnel: w944 -> [w1162]
          shift-right: [w1157] -> _
          shift-left: w992 -> [w1161]
          shift-right: [w1156] -> _
          shift-left: w991 -> [w1160]
          tunnel: [w1138] -> w989
          tunnel: [w1139] -> w990
          shift-right: [w1140] -> w960
          shift-left: w987 -> [w1105]
          shift-right: [w1155] -> _
          shift-left: w986 -> [w1100]
          shift-right: [w1127] -> w964
          shift-left: w975 -> [w1128]
          shift-right: [w1153] -> _
          shift-left: w985 -> [w1154]
          shift-right: [w1151] -> _
          shift-left: w984 -> [w1152]
          shift-right: [w1086] -> _
          shift-left: w939 -> [w1150]
          shift-right: [w1142] -> w966
          shift-left: w980 -> [w1143]
          shift-right: [w1129] -> _
          shift-left: w978 -> [w1137]
          shift-right: [w1097] -> _
          shift-left: w938 -> [w1136]
          shift-right: [w1130] -> _
          shift-left: w978 -> [w1135]
          shift-right: [w1131] -> _
          shift-left: w938 -> [w1134]
          shift-right: [w1098] -> _
          shift-left: w977 -> [w1132]
          shift-right: [w1099] -> _
          shift-left: w977 -> [w1133]
          shift-right: [w1111] -> _
          shift-left: w969 -> [w1112]
          shift-right: [w1110] -> w962
          shift-left: w968 -> [w1108]
          shift-right: [w1109] -> w963
          shift-left: FALSE ("output_Iconnected") -> [w1107]
          tunnel: "Data Set Prefix" -> [w1106]
          tunnel: [w1106] -> w961
          shift-right: [w1081] -> _
          shift-left: w939 -> [w1104]
          tunnel: w954 -> [w1101]
          shift-right: [w1095] -> _
          shift-left: 0 ("idxDataBlock") -> [w1096]
          shift-right: [w1092] -> _
          shift-left: w945 -> [w1094]
          shift-right: [w1091] -> _
          shift-left: w945 -> [w1093]
          shift-right: [w1080] -> _
          shift-left: w939 -> [w1087]
          shift-right: [w1083] -> _
          shift-left: w939 -> [w1085]
          shift-right: [w1082] -> _
          shift-left: w939 -> [w1084]
          shift-right: [w1073] -> _
          shift-left: w939 -> [w1074]
          shift-right: [w1066] -> w932
          shift-left: 0 -> [w1050]
          shift-right: [w1049] -> _
          shift-left: w935 -> [w1061]
          shift-right: [w1048] -> _
          shift-left: w935 -> [w1057]
          shift-right: [w1070] -> _
          shift-left: FALSE -> [w1070]
          shift-right: [w1056] -> _
          shift-left: w935 -> [w1064]
          shift-right: [w1067] -> w933
          shift-left: w934 -> [w1068]
          tunnel: w925 -> [w1055]
          tunnel: [w1054] -> w931
          tunnel: w923 -> [w1051]
          tunnel: [w1051] -> w930
          tunnel: w927 -> [w1053]
          tunnel: [w1052] -> w924
          stop <- w1149 stop-if-true
          # "iState"
          # "dataAnalog"
          # "index"
          # "iEvent"
          # "iBlock"
          # "iTrial"
          # "Laser"
          # "Audio R"
          # "Audio L"
          # "Solenoid R"
          # "Solenoid L"
          # "manual triggering"
          # "dataTrial"
          # "dataBlock"
          # "nRewards"
          # "laserOccurred"
          # "dataExp"
          # "dataCurrent"
          # "audio__L\naudio__R"
          # "time stamp"
          # "Audio params"
          # "nRewards"
          # "idxDataBlock"
          # "idxDataBlock"
          # "activate"
          # "audio__L\naudio__R"
          # "amp__R\nfreq__R"
          # "amp__L\nfreq__L"
          # "dataLC"
          # "solenoid__R"
          # "solenoid__L"
          # "Did a lick occur?"
          # "Update lick counter"
          # "spout"
          # "spout"
          # "state"
          # "state"
          n584 = node-c288() -> ()  [unwired: 1 in, 1 out]
          n585 = local read "MTrig_Solenoid_trig__L"() -> (w1125:bool)
          n586 = local read "MTrig_Solenoid_trig__R"() -> (w1124:bool)
          n587 = local read "MTrig_Audio_trig__L"() -> (w1123:bool)
          n588 = local read "MTrig_Audio_trig__R"() -> (w1122:bool)
          n589 = xnode "Read/Write Control"("FPGA VI Reference In"=w1163, "error in"=w1162) -> ("FPGA VI Reference Out"=w1090:refnum<k20>, "error out"=w1089:errorcluster, "A2_LickL"=w1157:u32, "A4_LickR"=w1156:u32)
          "A2" <- w1157
          "A4" <- w1156
          n590 = local read "MTrig_Laser_trig"() -> (w1121:bool)
          n591 = Greater?(x=w1157, y=w1161) -> (0:w1159:bool)
          n592 = Greater?(x=w1156, y=w1160) -> (0:w1158:bool)
          n593 = Or(x=w1159, y=w1158) -> (x .or. y?=w1165:bool)
          n594 = call "myRIO_BRig_RT_dataMTrig_main.vi"("input_dataMTrig"=w1128, "input_Solenoid_trig_L"=w1125, "input_Solenoid_trig_R"=w1124, "input_Audio_trig_L"=w1123, "input_Audio_trig_R"=w1122, "input_Laser_trig"=w1121) -> ("output_Laser"=w1078:bool, "output_dataMTrig"=w1127:u16[], "output_Solenoid_L"=w1115:bool, "output_Solenoid_R"=w1117:bool, "output_Audio_L"=w1119:bool, "output_Audio_R"=w1120:bool)  [unwired: 8 in]
          n595 = Compound Arithmetic op=OR(w1125, w1124, w1123, w1122, w1121) -> (w1126:bool)
          n596 = case shown="True" w1126 {
            frame False {
            }
            frame True {
              w1167 = FALSE
              n597 = local write "MTrig_Solenoid_trig__L"(w1167) -> ()
              n598 = local write "MTrig_Solenoid_trig__R"(w1167) -> ()
              n599 = local write "MTrig_Audio_trig__L"(w1167) -> ()
              n600 = local write "MTrig_Audio_trig__R"(w1167) -> ()
              n601 = local write "MTrig_Laser_trig"(w1167) -> ()
            }
          }
          n602 = case shown="\"ENL1_pre\"" w1046 {
            selector: w1046 -> [_ _ _ _ _ _ _ _ _ _ _ _ _ _ _ _ _ _ _ _ w1908 _ w1973 _ _ _ _ _ w2115 _ w2190 _ _ _ _ _ w2319 _ w2395 _ w2459 _ w2503 _ _ w2573 _ _ _ _ _ w2745 _ _ _ _ _ _ _ _ _ _ _ _ _ _ _ _ _ _ _]
            tunnel: [myRIO_BRig_RT__Case_Exp_stateList."Start2" ("Enum") myRIO_BRig_RT__Case_Exp_stateList."Start3" ("Enum") myRIO_BRig_RT__Case_Exp_stateList."saveSettings1" ("Enum") myRIO_BRig_RT__Case_Exp_stateList."saveSettings2" ("Enum") myRIO_BRig_RT__Case_Exp_stateList."saveSettings3" ("Enum") myRIO_BRig_RT__Case_Exp_stateList."saveSettings4_LC_ENL" ("Enum") myRIO_BRig_RT__Case_Exp_stateList."saveSettings5_LC_Cue" ("Enum") myRIO_BRig_RT__Case_Exp_stateList."saveSettings6_LC_Other" ("Enum") myRIO_BRig_RT__Case_Exp_stateList."setSettings_Audio" ("Enum") myRIO_BRig_RT__Case_Exp_stateList."setSettings_Laser" ("Enum") myRIO_BRig_RT__Case_Exp_stateList."commConnect" ("Enum") w1666 myRIO_BRig_RT__Case_Exp_stateList."initTrial" ("Enum") w1711 myRIO_BRig_RT__Case_Exp_stateList."initTrial3" ("Enum") myRIO_BRig_RT__Case_Exp_stateList."initTrial_LC_ENL1" ("Enum") myRIO_BRig_RT__Case_Exp_stateList."ENL1_pre" ("Enum") myRIO_BRig_RT__Case_Exp_stateList."initTrial_LC_Cue1" ("Enum") myRIO_BRig_RT__Case_Exp_stateList."initTrial4" ("Enum") w1867 w1905 myRIO_BRig_RT__Case_Exp_stateList."ENL1Penalty" ("Enum") w1974 myRIO_BRig_RT__Case_Exp_stateList."endExp" ("Enum") myRIO_BRig_RT__Case_Exp_stateList."endExp" ("Enum") myRIO_BRig_RT__Case_Exp_stateList."endExp" ("Enum") myRIO_BRig_RT__Case_Exp_stateList."endExp" ("Enum") w2069 w2114 myRIO_BRig_RT__Case_Exp_stateList."Cue1Penalty" ("Enum") w2188 myRIO_BRig_RT__Case_Exp_stateList."endExp" ("Enum") myRIO_BRig_RT__Case_Exp_stateList."endExp" ("Enum") myRIO_BRig_RT__Case_Exp_stateList."endExp" ("Enum") myRIO_BRig_RT__Case_Exp_stateList."endExp" ("Enum") w2276 w2327 myRIO_BRig_RT__Case_Exp_stateList."SelectReward" ("Enum") w2396 myRIO_BRig_RT__Case_Exp_stateList."SelectRewardPost" ("Enum") w2460 myRIO_BRig_RT__Case_Exp_stateList."SelectWrong" ("Enum") w2499 myRIO_BRig_RT__Case_Exp_stateList."endTrial1" ("Enum") myRIO_BRig_RT__Case_Exp_stateList."SelectTimeout" ("Enum") w2575 myRIO_BRig_RT__Case_Exp_stateList."endTrial1" ("Enum") myRIO_BRig_RT__Case_Exp_stateList."endTrial2" ("Enum") myRIO_BRig_RT__Case_Exp_stateList."saveData_dataBlock" ("Enum") w2658 w2728 w2745 myRIO_BRig_RT__Case_Exp_stateList."initBlock" ("Enum") w2772 myRIO_BRig_RT__Case_Exp_stateList."commUpload_dataCurrent" ("Enum") myRIO_BRig_RT__Case_Exp_stateList."commUpload_dataExp" ("Enum") myRIO_BRig_RT__Case_Exp_stateList."commUpload_dataLC" ("Enum") myRIO_BRig_RT__Case_Exp_stateList."commUpload_dataTrial" ("Enum") myRIO_BRig_RT__Case_Exp_stateList."endTrial3" ("Enum") myRIO_BRig_RT__Case_Exp_stateList."saveData_dataCurrent" ("Enum") myRIO_BRig_RT__Case_Exp_stateList."saveData_dataExp" ("Enum") myRIO_BRig_RT__Case_Exp_stateList."saveData_dataLC" ("Enum") myRIO_BRig_RT__Case_Exp_stateList."saveData_dataTrial" ("Enum") myRIO_BRig_RT__Case_Exp_stateList."commUpload_pre" ("Enum") myRIO_BRig_RT__Case_Exp_stateList."empty_endBlock2" ("Enum") myRIO_BRig_RT__Case_Exp_stateList."initBlock" ("Enum") myRIO_BRig_RT__Case_Exp_stateList."empty_endTrial2" ("Enum") myRIO_BRig_RT__Case_Exp_stateList."empty_endTrial3" ("Enum") myRIO_BRig_RT__Case_Exp_stateList."empty_endTrial4" ("Enum") myRIO_BRig_RT__Case_Exp_stateList."empty_endTrial5" ("Enum") myRIO_BRig_RT__Case_Exp_stateList."initTrial" ("Enum")] -> w1113
            tunnel: [w1193 w1212 w1234 w1289 w1337 w1404 w1456 w1508 w1552 w1578 w1637 w1643 w1674 w1693 w1727 w1757 w1790 w1815 w1842 w1883 w1921 w1951 w1978 w1994 w2016 w2035 w2054 w2088 w2136 w2161 w2187 w2208 w2229 w2248 w2267 w2287 w2345 w2370 w2393 w2407 w2457 w2481 w2513 w2534 w2554 w2586 w2609 w2621 w2640 w2682 w2701 w2744 w2761 w2775 w2809 w2830 w2851 w2872 w2893 w2921 w2941 w2968 w2988 w3013 w3032 w3051 w3070 w3089 w3108 w3127 w3146] -> w1164
            tunnel: w1166 -> [w1193 w1212 w1234 w1289 w1337 w1404 w1456 w1508 w1552 w1578 w1637 w1665 w1674 w1693 w1727 w1757 w1790 w1815 w1842 w1883 w1921 w1951 w1978 w1994 w2016 w2035 w2054 w2088 w2136 w2161 w2187 w2208 w2229 w2248 w2267 w2287 w2345 w2370 w2393 w2407 w2457 w2481 w2513 w2534 w2554 w2586 w2609 w2621 w2640 w2682 w2701 w2744 w2761 w2775 w2809 w2830 w2851 w2872 w2893 w2921 w2941 w2968 w2988 w3013 w3032 w3051 w3070 w3089 w3108 w3127 w3146]
            tunnel: w1165 -> [w1196 w1215 w1231 w1292 w1340 w1407 w1459 w1511 w1555 w1581 w1640 w1659 w1685 w1712 w1745 w1773 w1804 w1828 w1855 w1870 w1902 w1954 w1981 w2000 w2019 w2038 w2057 w2068 w2113 w2169 w2194 w2213 w2232 w2251 w2270 w2285 w2343 w2380 w2403 w2438 w2465 w2492 w2516 w2533 w2566 w2591 w2606 w2629 w2639 w2693 w2727 w2748 w2758 w2784 w2812 w2833 w2854 w2875 w2896 w2924 w2944 w2971 w2991 w3016 w3035 w3054 w3073 w3092 w3111 w3130 w3149]
            tunnel: w1159 -> [w1195 w1214 w1232 w1291 w1339 w1406 w1458 w1510 w1554 w1580 w1639 w1658 w1684 w1713 w1744 w1774 w1805 w1829 w1856 w1893 w1923 w1953 w1980 w1999 w2018 w2037 w2056 w2102 w2137 w2168 w2193 w2212 w2231 w2250 w2269 w2286 w2342 w2379 w2402 w2437 w2464 w2491 w2515 w2532 w2565 w2590 w2607 w2630 w2638 w2692 w2726 w2747 w2759 w2785 w2811 w2832 w2853 w2874 w2895 w2923 w2943 w2970 w2990 w3015 w3034 w3053 w3072 w3091 w3110 w3129 w3148]
            tunnel: w1158 -> [w1194 w1213 w1233 w1290 w1338 w1405 w1457 w1509 w1553 w1579 w1638 w1657 w1683 w1714 w1743 w1775 w1806 w1830 w1857 w1892 w1922 w1952 w1979 w1998 w2017 w2036 w2055 w2101 w2138 w2167 w2192 w2211 w2230 w2249 w2268 w2305 w2346 w2378 w2401 w2436 w2463 w2490 w2514 w2531 w2564 w2589 w2608 w2631 w2637 w2691 w2725 w2746 w2760 w2786 w2810 w2831 w2852 w2873 w2894 w2922 w2942 w2969 w2989 w3014 w3033 w3052 w3071 w3090 w3109 w3128 w3147]
            tunnel: [w1196 w1215 w1231 w1292 w1340 w1407 w1459 w1511 w1555 w1581 w1640 w1659 w1685 w1712 w1745 w1773 w1804 w1828 w1855 w1870 w1902 w1954 w1981 w2000 w2019 w2038 w2057 w2068 w2113 w2169 w2194 w2213 w2232 w2251 w2270 w2285 w2343 w2380 w2403 w2438 w2465 w2492 w2516 w2533 w2566 w2591 w2606 w2629 w2639 w2693 w2727 w2748 w2758 w2784 w2812 w2833 w2854 w2875 w2896 w2924 w2944 w2971 w2991 w3016 w3035 w3054 w3073 w3092 w3111 w3130 w3149] -> w1146
            tunnel: [w1195 w1214 w1232 w1291 w1339 w1406 w1458 w1510 w1554 w1580 w1639 w1658 w1684 w1713 w1744 w1774 w1805 w1829 w1856 w1893 w1923 w1953 w1980 w1999 w2018 w2037 w2056 w2102 w2137 w2168 w2193 w2212 w2231 w2250 w2269 w2286 w2342 w2379 w2402 w2437 w2464 w2491 w2515 w2532 w2565 w2590 w2607 w2630 w2638 w2692 w2726 w2747 w2759 w2785 w2811 w2832 w2853 w2874 w2895 w2923 w2943 w2970 w2990 w3015 w3034 w3053 w3072 w3091 w3110 w3129 w3148] -> w1145
            tunnel: [w1194 w1213 w1233 w1290 w1338 w1405 w1457 w1509 w1553 w1579 w1638 w1657 w1683 w1714 w1743 w1775 w1806 w1830 w1857 w1892 w1922 w1952 w1979 w1998 w2017 w2036 w2055 w2101 w2138 w2167 w2192 w2211 w2230 w2249 w2268 w2305 w2346 w2378 w2401 w2436 w2463 w2490 w2514 w2531 w2564 w2589 w2608 w2631 w2637 w2691 w2725 w2746 w2760 w2786 w2810 w2831 w2852 w2873 w2894 w2922 w2942 w2969 w2989 w3014 w3033 w3052 w3071 w3090 w3109 w3128 w3147] -> w1144
            tunnel: w1105 -> [w1192 w1211 w1230 w1256 w1313 w1381 w1455 w1507 w1551 w1576 w1597 w1664 w1673 w1710 w1716 w1758 w1785 w1812 w1841 w1882 w1907 w1945 w1977 w1995 w2015 w2034 w2053 w2072 w2133 w2160 w2191 w2209 w2228 w2247 w2266 w2296 w2323 w2362 w2398 w2409 w2462 w2482 w2512 w2530 w2555 w2588 w2605 w2618 w2642 w2662 w2699 w2743 w2762 w2787 w2806 w2827 w2848 w2869 w2880 w2910 w2929 w2953 w2985 w3002 w3022 w3041 w3060 w3079 w3098 w3117 w3136]
            tunnel: w1100 -> [w1191 w1210 w1229 w1287 w1335 w1401 w1453 w1505 w1549 w1569 w1633 w1663 w1682 w1709 w1724 w1756 w1792 w1818 w1845 w1885 w1920 w1944 w1975 w1997 w2014 w2033 w2052 w2090 w2135 w2158 w2186 w2210 w2227 w2246 w2265 w2298 w2344 w2376 w2400 w2430 w2458 w2483 w2510 w2529 w2557 w2585 w2604 w2628 w2645 w2661 w2718 w2742 w2763 w2788 w2805 w2826 w2847 w2868 w2881 w2918 w2938 w2949 w2984 w3010 w3029 w3048 w3067 w3086 w3105 w3124 w3143]
            tunnel: [w1192 w1211 w1230 w1256 w1313 w1380 w1455 w1507 w1551 w1576 w1619 w1648 w1673 w1698 w1716 w1758 w1785 w1811 w1840 w1886 w1906 w1946 w1976 w1995 w2015 w2034 w2053 w2097 w2132 w2159 w2189 w2209 w2228 w2247 w2266 w2299 w2318 w2377 w2397 w2431 w2461 w2484 w2511 w2530 w2558 w2587 w2605 w2617 w2641 w2662 w2697 w2743 w2762 w2787 w2806 w2827 w2848 w2869 w2880 w2910 w2929 w2953 w2985 w3002 w3022 w3041 w3060 w3079 w3098 w3117 w3136] -> w1141
            tunnel: [w1191 w1210 w1229 w1286 w1334 w1396 w1453 w1505 w1549 w1569 w1633 w1662 w1682 w1708 w1724 w1756 w1792 w1818 w1845 w1885 w1920 w1944 w1975 w1997 w2014 w2033 w2052 w2090 w2135 w2158 w2186 w2210 w2227 w2246 w2265 w2298 w2344 w2376 w2400 w2430 w2458 w2483 w2510 w2529 w2557 w2585 w2604 w2628 w2645 w2661 w2718 w2742 w2763 w2788 w2805 w2826 w2847 w2868 w2881 w2918 w2938 w2952 w2984 w3010 w3029 w3048 w3067 w3086 w3105 w3124 w3143] -> w1155
            tunnel: [_ _ _ _ _ _ _ _ _ _ _ _ _ _ _ _ _ _ _ _ _ _ _ _ _ _ _ _ _ _ _ _ _ _ _ _ _ _ w2391 _ _ _ _ _ _ _ _ _ _ _ _ _ _ _ _ _ _ _ _ _ _ _ _ _ _ _ _ _ _ _ _] -> w1116
            tunnel: [_ _ _ _ _ _ _ _ _ _ _ _ _ _ _ _ _ _ _ _ _ _ _ _ _ _ _ _ _ _ _ _ _ _ _ _ _ _ w2392 _ _ _ _ _ _ _ _ _ _ _ _ _ _ _ _ _ _ _ _ _ _ _ _ _ _ _ _ _ _ _ _] -> w1118
            tunnel: w1154 -> [w1189 w1208 w1227 w1258 w1315 w1402 w1454 w1506 w1550 w1574 w1634 w1660 w1675 w1706 w1736 w1771 w1802 w1808 w1837 w1884 w1919 w1941 w1971 w1996 w2012 w2031 w2050 w2096 w2134 w2157 w2184 w2206 w2225 w2244 w2263 w2297 w2340 w2368 w2399 w2411 w2455 w2480 w2508 w2527 w2556 w2584 w2602 w2620 w2647 w2689 w2710 w2740 w2765 w2790 w2803 w2824 w2845 w2866 w2890 w2904 w2931 w2959 w2978 w3004 w3023 w3042 w3061 w3080 w3099 w3118 w3137]
            tunnel: [w1189 w1208 w1227 w1258 w1315 w1402 w1454 w1506 w1550 w1574 w1634 w1660 w1672 w1706 w1736 w1771 w1802 w1808 w1837 w1884 w1919 w1941 w1971 w1996 w2012 w2031 w2050 w2096 w2134 w2157 w2184 w2206 w2225 w2244 w2263 w2297 w2340 w2368 w2399 w2410 w2455 w2480 w2508 w2527 w2556 w2584 w2602 w2619 w2647 w2689 w2710 w2740 w2765 w2790 w2803 w2824 w2845 w2866 w2890 w2904 w2931 w2959 w2978 w3004 w3023 w3042 w3061 w3080 w3099 w3118 w3137] -> w1153
            tunnel: w1152 -> [w1190 w1209 w1228 w1257 w1314 w1403 w1451 w1503 w1547 w1575 w1635 w1661 w1681 w1707 w1715 w1772 w1803 w1816 w1843 w1881 w1901 w1942 w1972 w1993 w2013 w2032 w2051 w2095 w2112 w2156 w2185 w2207 w2226 w2245 w2264 w2295 w2341 w2369 w2394 w2428 w2456 w2479 w2509 w2528 w2553 w2582 w2603 w2627 w2646 w2690 w2717 w2741 w2764 w2789 w2804 w2825 w2846 w2867 w2891 w2917 w2937 w2965 w2976 w3009 w3028 w3047 w3066 w3085 w3104 w3123 w3142]
            tunnel: [w1190 w1209 w1228 w1257 w1314 w1403 w1452 w1504 w1548 w1575 w1635 w1661 w1681 w1707 w1715 w1772 w1803 w1816 w1843 w1881 w1901 w1942 w1972 w1993 w2013 w2032 w2051 w2095 w2112 w2156 w2185 w2207 w2226 w2245 w2264 w2295 w2341 w2369 w2394 w2428 w2456 w2479 w2509 w2528 w2553 w2582 w2603 w2627 w2646 w2690 w2717 w2741 w2764 w2789 w2804 w2825 w2846 w2867 w2891 w2917 w2937 w2965 w2976 w3009 w3028 w3047 w3066 w3085 w3104 w3123 w3142] -> w1151
            tunnel: w1150 -> [_ _ _ _ _ _ _ _ _ _ _ _ _ _ _ _ _ _ _ w1866 w1894 w1927 w1960 _ _ _ _ _ w2106 w2143 _ _ _ _ _ _ _ _ _ _ _ _ _ _ _ w2583 _ _ _ _ _ _ _ _ _ _ _ _ _ _ _ _ _ _ _ _ _ _ _ _ _]
            tunnel: [_ _ _ _ _ _ _ _ _ _ _ _ _ _ _ _ _ _ _ _ _ _ _ _ _ _ _ _ _ _ _ _ _ _ _ _ _ _ _ _ _ _ _ _ _ _ _ _ _ _ _ TRUE _ _ _ _ _ _ _ _ _ _ _ _ _ _ _ _ _ _ _] -> w1147
            tunnel: w1137 -> [w1187 w1206 w1225 w1248 w1308 w1391 w1438 w1490 w1519 _ w1625 w1656 w1680 w1705 w1735 w1770 w1801 w1827 w1854 w1880 w1918 w1939 w1970 w1991 w2010 w2029 w2048 w2094 w2129 w2154 w2183 w2204 w2223 w2242 w2261 w2294 w2339 w2358 w2390 w2426 w2454 w2477 w2507 w2526 w2551 w2581 w2601 w2625 w2651 w2688 w2714 w2738 w2756 w2783 w2801 w2822 w2843 w2864 w2888 w2915 w2935 w2963 w2982 w3008 w3027 w3046 w3065 w3084 w3103 w3122 w3141]
            tunnel: w1136 -> [w1186 w1205 w1224 w1247 w1307 w1390 w1437 w1489 w1520 _ w1624 w1655 w1679 w1704 w1734 w1769 w1800 w1826 w1853 w1879 w1917 w1938 w1969 w1990 w2009 w2028 w2047 w2093 w2128 w2153 w2182 w2203 w2222 w2241 w2260 w2293 w2338 w2357 w2389 w2425 w2453 w2476 w2506 w2525 w2550 w2580 w2600 w2624 w2650 w2687 w2713 w2737 w2755 w2782 w2800 w2821 w2842 w2863 w2887 w2914 w2934 w2962 w2981 w3007 w3026 w3045 w3064 w3083 w3102 w3121 w3140]
            tunnel: w1135 -> [w1185 w1204 w1223 w1246 w1306 w1389 w1436 w1488 w1521 _ w1623 w1654 w1678 w1703 w1733 w1768 w1799 w1825 w1852 w1878 w1916 w1937 w1968 w1989 w2008 w2027 w2046 w2092 w2127 w2152 w2181 w2202 w2221 w2240 w2259 w2292 w2337 w2356 w2388 w2424 w2452 w2475 w2505 w2524 w2549 w2579 w2599 w2623 w2649 w2686 w2712 w2736 w2754 w2781 w2799 w2820 w2841 w2862 w2886 w2913 w2933 w2961 w2980 w3006 w3025 w3044 w3063 w3082 w3101 w3120 w3139]
            tunnel: w1134 -> [w1184 w1203 w1222 w1245 w1305 w1388 w1435 w1487 w1522 _ w1622 w1653 w1677 w1702 w1732 w1767 w1798 w1824 w1851 w1877 w1915 w1936 w1967 w1988 w2007 w2026 w2045 w2091 w2126 w2151 w2180 w2201 w2220 w2239 w2258 w2291 w2336 w2355 w2387 w2423 w2451 w2474 w2504 w2523 w2548 w2578 w2598 w2622 w2648 w2685 w2711 w2735 w2753 w2780 w2798 w2819 w2840 w2861 w2885 w2912 w2932 w2960 w2979 w3005 w3024 w3043 w3062 w3081 w3100 w3119 w3138]
            tunnel: w1133 -> [_ _ _ _ _ _ _ _ _ _ _ _ _ _ _ _ _ _ _ _ _ _ _ _ _ _ _ _ w2131 _ _ _ _ _ _ _ _ _ _ _ _ _ _ _ _ _ _ _ _ _ _ _ _ _ _ _ _ _ _ _ _ _ _ _ _ _ _ _ _ _ _]
            tunnel: w1132 -> [_ _ _ _ _ _ _ _ _ _ _ _ _ _ _ _ _ _ _ _ _ _ _ _ _ _ _ _ w2130 _ _ _ _ _ _ _ _ _ _ _ _ _ _ _ _ _ _ _ _ _ _ _ _ _ _ _ _ _ _ _ _ _ _ _ _ _ _ _ _ _ _]
            tunnel: [w1187 w1206 w1225 w1248 w1308 w1391 w1438 w1490 w1519 w1568 w1625 w1656 w1680 w1705 w1735 w1770 w1801 w1827 w1854 w1880 w1918 w1939 w1970 w1991 w2010 w2029 w2048 w2094 w2129 w2154 w2183 w2204 w2223 w2242 w2261 w2294 w2339 w2358 w2390 w2426 w2454 w2477 w2507 w2526 w2551 w2581 w2601 w2625 w2651 w2688 w2714 w2738 w2756 w2783 w2801 w2822 w2843 w2864 w2888 w2915 w2935 w2963 w2982 w3008 w3027 w3046 w3065 w3084 w3103 w3122 w3141] -> w1129
            tunnel: [w1186 w1205 w1224 w1247 w1307 w1390 w1437 w1489 w1520 w1559 w1624 w1655 w1679 w1704 w1734 w1769 w1800 w1826 w1853 w1879 w1917 w1938 w1969 w1990 w2009 w2028 w2047 w2093 w2128 w2153 w2182 w2203 w2222 w2241 w2260 w2293 w2338 w2357 w2389 w2425 w2453 w2476 w2506 w2525 w2550 w2580 w2600 w2624 w2650 w2687 w2713 w2737 w2755 w2782 w2800 w2821 w2842 w2863 w2887 w2914 w2934 w2962 w2981 w3007 w3026 w3045 w3064 w3083 w3102 w3121 w3140] -> w1097
            tunnel: [w1185 w1204 w1223 w1246 w1306 w1389 w1436 w1488 w1521 w1567 w1623 w1654 w1678 w1703 w1733 w1768 w1799 w1825 w1852 w1878 w1916 w1937 w1968 w1989 w2008 w2027 w2046 w2092 w2127 w2152 w2181 w2202 w2221 w2240 w2259 w2292 w2337 w2356 w2388 w2424 w2452 w2475 w2505 w2524 w2549 w2579 w2599 w2623 w2649 w2686 w2712 w2736 w2754 w2781 w2799 w2820 w2841 w2862 w2886 w2913 w2933 w2961 w2980 w3006 w3025 w3044 w3063 w3082 w3101 w3120 w3139] -> w1130
            tunnel: [w1184 w1203 w1222 w1245 w1305 w1388 w1435 w1487 w1522 w1557 w1622 w1653 w1677 w1702 w1732 w1767 w1798 w1824 w1851 w1877 w1915 w1936 w1967 w1988 w2007 w2026 w2045 w2091 w2126 w2151 w2180 w2201 w2220 w2239 w2258 w2291 w2336 w2355 w2387 w2423 w2451 w2474 w2504 w2523 w2548 w2578 w2598 w2622 w2648 w2685 w2711 w2735 w2753 w2780 w2798 w2819 w2840 w2861 w2885 w2912 w2932 w2960 w2979 w3005 w3024 w3043 w3062 w3081 w3100 w3119 w3138] -> w1131
            tunnel: [_ _ _ _ _ _ _ _ _ _ _ _ _ _ _ _ _ _ _ _ _ _ _ _ _ _ _ w2081 w2131 _ _ _ _ _ _ _ _ _ _ _ _ _ _ _ _ _ _ _ _ _ _ _ _ _ _ _ _ _ _ _ _ _ _ _ _ _ _ _ _ _ _] -> w1099
            tunnel: [_ _ _ _ _ _ _ _ _ _ _ _ _ _ _ _ _ _ _ _ _ _ _ _ _ _ _ w2080 w2130 _ _ _ _ _ _ _ _ _ _ _ _ _ _ _ _ _ _ _ _ _ _ _ _ _ _ _ _ _ _ _ _ _ _ _ _ _ _ _ _ _ _] -> w1098
            tunnel: w1112 -> [w1183 w1202 w1221 w1244 w1304 w1387 w1434 w1486 w1518 w1566 w1632 w1652 w1676 w1701 w1718 w1760 w1784 w1810 w1839 w1876 w1914 w1935 w1966 w1987 w2006 w2025 w2044 w2079 w2125 w2150 w2179 w2200 w2219 w2238 w2257 w2290 w2335 w2352 w2386 w2422 w2450 w2471 w2498 w2522 w2545 w2572 w2597 w2616 w2644 w2678 w2709 w2734 w2766 w2791 w2802 w2823 w2844 w2865 w2889 w2916 w2936 w2964 w2983 w2999 w3021 w3040 w3059 w3078 w3097 w3116 w3135]
            tunnel: [w1183 w1202 w1221 w1244 w1304 w1387 w1434 w1486 w1518 w1566 w1632 w1652 w1676 w1701 w1717 w1759 w1777 w1809 w1838 w1876 w1914 w1935 w1966 w1987 w2006 w2025 w2044 w2079 w2125 w2150 w2179 w2200 w2219 w2238 w2257 w2290 w2335 w2352 w2386 w2422 w2450 w2471 w2498 w2522 w2545 w2572 w2597 w2616 w2643 w2678 w2709 w2734 w2766 w2791 w2802 w2823 w2844 w2865 w2889 w2916 w2936 w2964 w2983 w2999 w3021 w3040 w3059 w3078 w3097 w3116 w3135] -> w1111
            tunnel: [w1182 w1201 w1220 w1243 w1303 w1386 w1433 w1485 w1517 w1565 w1631 w1651 w1687 w1700 w1738 w1766 w1797 w1823 w1850 w1875 w1913 w1934 w1965 w1986 w2005 w2024 w2043 w2078 w2124 w2149 w2178 w2199 w2218 w2237 w2256 w2289 w2334 w2351 w2385 w2421 w2449 w2470 w2497 w2521 w2544 w2571 w2596 w2615 w2636 w2684 w2708 w2732 w2767 w2777 w2797 w2818 w2839 w2860 w2884 w2920 w2940 w2967 w2987 w3012 w3031 w3050 w3069 w3088 w3107 w3126 w3145] -> w1110
            tunnel: [w1181 w1200 w1219 w1242 w1302 w1385 w1432 w1484 w1516 w1564 w1630 w1650 w1686 w1699 w1737 w1765 w1796 w1822 w1849 w1874 w1912 w1933 w1964 w1985 w2004 w2023 w2042 w2077 w2123 w2148 w2177 w2198 w2217 w2236 w2255 w2288 w2333 w2350 w2384 w2420 w2448 w2469 w2496 w2520 w2543 w2570 w2595 w2614 w2635 w2683 w2707 w2733 w2749 w2774 w2807 w2828 w2849 w2870 w2892 w2919 w2939 w2966 w2986 w3011 w3030 w3049 w3068 w3087 w3106 w3125 w3144] -> w1109
            tunnel: w1108 -> [w1182 w1201 w1220 w1243 w1303 w1386 w1433 w1485 w1517 w1565 w1631 w1651 w1687 w1700 w1738 w1766 w1797 w1823 w1850 w1875 w1913 w1934 w1965 w1986 w2005 w2024 w2043 w2078 w2124 w2149 w2178 w2199 w2218 w2237 w2256 w2289 w2334 w2351 w2385 w2421 w2449 w2470 w2497 w2521 w2544 w2571 w2596 w2615 w2636 w2684 w2708 w2732 _ w2777 w2797 w2818 w2839 w2860 w2884 w2920 w2940 w2967 w2987 w3012 w3031 w3050 w3069 w3088 w3107 w3126 w3145]
            tunnel: w1107 -> [w1181 w1200 w1219 w1242 w1302 w1385 w1432 w1484 w1516 w1564 w1630 w1650 w1686 w1699 w1737 w1765 w1796 w1822 w1849 w1874 w1912 w1933 w1964 w1985 w2004 w2023 w2042 w2077 w2123 w2148 w2177 w2198 w2217 w2236 w2255 w2288 w2333 w2350 w2384 w2420 w2448 w2469 w2496 w2520 w2543 w2570 w2595 w2614 w2635 w2683 w2707 w2733 _ w2774 w2807 w2828 w2849 w2870 w2892 w2919 w2939 w2966 w2986 w3011 w3030 w3049 w3068 w3087 w3106 w3125 w3144]
            tunnel: w1106 -> [_ _ _ _ _ _ _ _ _ _ _ _ _ _ _ _ _ _ _ _ _ _ _ _ _ _ _ _ _ _ _ _ _ _ _ _ _ _ _ _ _ _ _ _ _ _ _ _ _ _ _ _ _ _ w2795 w2816 w2837 w2858 w2882 _ _ _ _ _ _ _ _ _ _ _ _]
            tunnel: w1104 -> [_ _ _ _ _ _ _ _ _ _ _ _ _ _ _ _ w1789 _ w1834 w1863 w1899 w1925 w1956 _ _ _ _ w2059 w2104 w2142 w2171 _ _ _ _ _ _ _ _ _ _ _ _ _ _ _ _ _ _ _ _ _ _ _ _ _ _ _ _ _ _ _ _ _ _ _ _ _ _ _ _]
            tunnel: w1101 -> [_ _ _ _ _ _ _ _ _ _ _ _ _ _ _ _ _ _ _ _ _ _ _ _ _ _ _ _ _ _ _ _ _ _ _ _ _ _ _ _ _ _ _ _ _ _ _ _ _ _ _ _ _ _ _ _ _ _ _ _ _ w2954 _ _ _ _ _ _ _ _ _]
            tunnel: [w1180 w1199 w1218 w1241 w1301 w1384 w1431 w1483 w1515 w1563 w1629 w1646 w1670 w1696 w1739 w1764 w1795 w1821 w1848 w1873 w1911 w1932 w1963 w1984 w2003 w2022 w2041 w2076 w2122 w2147 w2176 w2197 w2216 w2235 w2254 w2284 w2332 w2349 w2383 w2405 w2447 w2468 w2495 w2519 w2542 w2569 w2594 w2613 w2634 w2681 w2694 w2731 w2752 w2776 w2794 w2815 w2836 w2857 w2879 w2899 w2928 w2948 w2975 w2995 w3020 w3039 w3058 w3077 w3096 w3115 w3134] -> w1095
            tunnel: w1096 -> [w1180 w1199 w1218 w1241 w1301 w1384 w1431 w1483 w1515 w1563 w1629 w1646 _ w1696 w1739 w1764 w1795 w1821 w1848 w1873 w1911 w1932 w1963 w1984 w2003 w2022 w2041 w2076 w2122 w2147 w2176 w2197 w2216 w2235 w2254 w2284 w2332 w2349 w2383 w2405 w2447 w2468 w2495 w2519 w2542 w2569 w2594 w2613 w2634 w2681 w2695 w2731 w2752 w2776 w2794 w2815 w2836 w2857 w2879 w2899 w2928 w2948 w2975 w2995 w3020 w3039 w3058 w3077 w3096 w3115 w3134]
            tunnel: w1094 -> [w1179 w1198 w1217 w1240 w1300 w1383 w1430 w1482 w1514 w1562 w1628 w1645 w1669 w1695 w1731 w1763 w1794 w1820 w1847 w1872 w1910 w1931 w1962 w1983 w2002 w2021 w2040 w2075 w2121 w2146 w2175 w2196 w2215 w2234 w2253 w2283 w2331 w2348 w2382 w2419 w2446 w2467 w2494 w2518 w2541 w2568 w2593 w2612 w2633 w2680 w2706 w2730 w2751 w2779 w2793 w2814 w2835 w2856 w2878 w2898 w2927 w2947 w2974 w2994 w3019 w3038 w3057 w3076 w3095 w3114 w3133]
            tunnel: w1093 -> [w1178 w1197 w1216 w1239 w1299 w1382 w1429 w1481 w1513 w1561 w1627 w1644 w1668 w1694 w1730 w1762 w1793 w1819 w1846 w1871 w1909 w1930 w1961 w1982 w2001 w2020 w2039 w2074 w2120 w2145 w2174 w2195 w2214 w2233 w2252 w2282 w2330 w2347 w2381 w2416 w2445 w2466 w2493 w2517 w2540 w2567 w2592 w2611 w2632 w2679 w2705 w2729 w2750 w2778 w2792 w2813 w2834 w2855 w2877 w2897 w2926 w2946 w2973 w2993 w3018 w3037 w3056 w3075 w3094 w3113 w3132]
            tunnel: [w1179 w1198 w1217 w1240 w1300 w1383 w1430 w1482 w1514 w1562 w1628 w1645 w1669 w1695 w1731 w1763 w1794 w1820 w1847 w1872 w1910 w1931 w1962 w1983 w2002 w2021 w2040 w2075 w2121 w2146 w2175 w2196 w2215 w2234 w2253 w2283 w2331 w2348 w2382 w2418 w2446 w2467 w2494 w2518 w2541 w2568 w2593 w2612 w2633 w2680 w2706 w2730 w2751 w2779 w2793 w2814 w2835 w2856 w2878 w2898 w2927 w2947 w2974 w2994 w3019 w3038 w3057 w3076 w3095 w3114 w3133] -> w1092
            tunnel: [w1178 w1197 w1216 w1239 w1299 w1382 w1429 w1481 w1513 w1561 w1627 w1644 w1668 w1694 w1730 w1762 w1793 w1819 w1846 w1871 w1909 w1930 w1961 w1982 w2001 w2020 w2039 w2074 w2120 w2145 w2174 w2195 w2214 w2233 w2252 w2282 w2330 w2347 w2381 w2417 w2445 w2466 w2493 w2517 w2540 w2567 w2592 w2611 w2632 w2679 w2705 w2729 w2750 w2778 w2792 w2813 w2834 w2855 w2877 w2897 w2926 w2946 w2973 w2993 w3018 w3037 w3056 w3075 w3094 w3113 w3132] -> w1091
            tunnel: w1090 -> [_ _ _ _ _ _ _ _ _ _ w1620 _ _ _ w1742 w1752 _ _ _ _ _ _ _ _ _ _ _ _ w2117 _ _ _ _ _ _ w2280 w2329 _ _ _ _ _ _ _ w2539 _ _ _ _ w2656 _ _ _ _ _ _ _ _ _ _ _ _ _ _ _ _ _ _ _ _ _]
            tunnel: w1089 -> [_ _ _ _ _ _ _ _ _ _ w1621 _ _ _ w1741 w1751 _ _ _ _ _ _ _ _ _ _ _ _ w2116 _ _ _ _ _ _ w2281 w2328 _ _ _ _ _ _ _ w2538 _ _ _ _ w2655 _ _ _ _ _ _ _ _ _ _ _ _ _ _ _ _ _ _ _ _ _]
            tunnel: w1087 -> [_ _ _ _ _ _ _ _ _ _ _ _ _ _ _ _ w1788 _ w1833 w1862 w1898 w1924 w1957 _ _ _ _ w2058 w2103 w2141 w2170 _ _ _ _ _ _ _ _ _ _ _ _ _ _ _ _ _ _ _ _ _ _ _ _ _ _ _ _ _ _ _ _ _ _ _ _ _ _ _ _]
            tunnel: [_ _ _ _ _ _ _ _ _ _ _ _ _ _ _ _ _ _ _ w1866 w1900 w1927 w1960 _ _ _ _ TRUE w2106 w2143 _ _ _ _ _ _ _ _ _ _ _ _ _ _ _ _ _ _ _ _ _ _ _ _ _ _ _ _ _ _ _ _ _ _ _ _ _ _ _ _ _] -> w1086
            tunnel: w1085 -> [_ _ _ _ _ _ _ _ _ _ _ _ _ _ _ _ w1787 _ _ w1865 w1904 w1929 w1958 _ _ _ _ w2066 w2111 w2140 w2173 _ _ _ _ _ _ _ _ _ _ _ _ _ _ _ _ _ _ _ _ _ _ _ _ _ _ _ _ _ _ _ _ _ _ _ _ _ _ _ _]
            tunnel: w1084 -> [_ _ _ _ _ _ _ _ _ _ _ _ _ _ _ _ w1786 _ _ w1864 w1903 w1928 w1959 _ _ _ _ w2065 w2110 w2139 w2172 _ _ _ _ _ _ _ _ _ _ _ _ _ _ _ _ _ _ _ _ _ _ _ _ _ _ _ _ _ _ _ _ _ _ _ _ _ _ _ _]
            tunnel: [_ _ _ _ _ _ _ _ _ _ _ _ _ _ _ _ w1787 _ w1836 w1865 w1904 w1929 w1958 _ _ _ _ w2066 w2111 w2140 w2173 _ _ _ _ _ _ _ _ _ _ _ _ _ _ _ _ _ _ _ _ _ _ _ _ _ _ _ _ _ _ _ _ _ _ _ _ _ _ _ _] -> w1083
            tunnel: [_ _ _ _ _ _ _ _ _ _ _ _ _ _ _ _ w1786 _ w1835 w1864 w1903 w1928 w1959 _ _ _ _ w2065 w2110 w2139 w2172 _ _ _ _ _ _ _ _ _ _ _ _ _ _ _ _ _ _ _ _ _ _ _ _ _ _ _ _ _ _ _ _ _ _ _ _ _ _ _ _] -> w1082
            tunnel: [_ _ _ _ _ _ _ _ _ _ _ _ _ _ _ _ w1789 w1813 w1834 w1863 w1899 w1925 w1956 _ _ _ _ w2059 w2104 w2142 w2171 _ _ _ _ _ _ _ _ _ _ _ _ _ _ _ _ _ _ _ _ _ _ _ _ _ _ _ _ _ _ _ _ _ _ _ _ _ _ _ _] -> w1081
            tunnel: [_ _ _ _ _ _ _ _ _ _ _ _ _ _ _ _ w1788 w1814 w1833 w1862 w1898 w1924 w1957 _ _ _ _ w2058 w2103 w2141 w2170 _ _ _ _ _ _ _ _ _ _ _ _ _ _ _ _ _ _ _ _ _ _ _ _ _ _ _ _ _ _ _ _ _ _ _ _ _ _ _ _] -> w1080
            tunnel: [_ _ _ _ _ _ _ _ _ _ _ _ _ _ _ _ _ _ _ _ w1897 _ _ _ _ _ _ _ w2108 _ _ _ _ _ _ _ _ _ _ _ _ _ _ _ _ _ _ _ _ _ _ _ _ _ _ _ _ _ _ _ _ _ _ _ _ _ _ _ _ _ _] -> w1077
            tunnel: [_ _ _ _ _ _ _ _ _ _ _ _ _ _ _ _ _ _ _ _ w1896 _ _ _ _ _ _ _ w2109 _ _ _ _ _ _ _ _ _ _ _ _ _ _ _ _ _ _ _ _ _ _ _ _ _ _ _ _ _ _ _ _ _ _ _ _ _ _ _ _ _ _] -> w1079
            tunnel: w1074 -> [_ _ _ _ _ _ _ _ _ _ _ _ _ _ _ _ _ _ _ w1861 w1895 w1926 w1955 _ _ _ _ w2061 w2105 w2144 _ _ _ _ _ _ _ _ _ _ _ _ _ _ _ _ _ _ _ _ _ _ _ _ _ _ _ _ _ _ _ _ _ _ _ _ _ _ _ _ _]
            tunnel: [_ _ _ _ _ _ _ _ _ _ _ _ _ _ _ _ _ _ _ w1861 w1895 w1926 w1955 _ _ _ _ w2061 w2107 w2144 _ _ _ _ _ _ _ _ _ _ _ _ _ _ _ _ _ _ _ _ _ _ _ _ _ _ _ _ _ _ _ _ _ _ _ _ _ _ _ _ _] -> w1073
            tunnel: [_ _ _ _ _ _ _ _ _ _ _ _ _ _ _ _ _ w1807 w1832 _ _ _ _ _ _ _ _ _ _ _ _ _ _ _ _ _ _ _ _ _ _ _ _ _ _ _ _ _ _ _ _ _ _ _ _ _ _ _ _ _ _ _ _ _ _ _ _ _ _ _ _] -> w1072
            tunnel: [_ _ _ _ _ _ _ _ _ _ _ _ _ _ _ _ _ _ TRUE ("Recording") _ _ _ _ _ _ _ _ _ _ _ _ _ _ _ _ _ _ _ _ _ _ _ _ _ _ _ _ _ _ _ _ _ _ _ _ _ _ _ _ _ _ _ _ _ _ _ _ _ _ _ _] -> w1069
            tunnel: [_ _ _ _ _ _ _ _ _ _ _ _ _ _ _ _ _ w1807 _ _ _ _ _ _ _ _ _ _ _ _ _ _ _ _ _ _ _ _ _ _ _ _ _ _ _ _ _ _ _ _ _ _ _ _ _ _ _ _ _ _ _ _ _ _ _ _ _ _ _ _ _] -> w1065
            tunnel: [_ _ _ _ _ _ _ _ _ _ _ TRUE _ _ _ _ _ _ _ _ _ _ _ _ _ _ _ _ _ _ _ _ _ _ _ _ _ _ _ _ _ _ _ _ _ _ _ _ _ _ _ _ _ _ _ _ _ _ _ _ _ _ _ _ _ _ _ _ _ _ _] -> w1062
            tunnel: [_ _ _ _ _ _ _ _ _ _ _ w1641 _ _ _ _ _ _ _ _ _ _ _ _ _ _ _ _ _ _ _ _ _ _ _ _ _ _ _ _ _ _ _ _ _ _ _ _ _ _ _ _ _ _ _ _ _ _ _ _ _ _ _ _ _ _ _ _ _ _ _] -> w1060
            tunnel: [_ _ _ _ _ _ _ _ _ _ _ _ _ TRUE _ _ _ _ _ _ _ _ _ _ _ _ _ _ _ _ _ _ _ _ _ _ _ _ _ _ _ _ _ _ _ _ _ _ _ _ _ _ _ _ _ _ _ _ _ _ _ _ _ _ _ _ _ _ _ _ _] -> w1059
            tunnel: [_ _ _ _ _ _ _ _ _ _ _ _ _ w1688 _ _ _ _ _ _ _ _ _ _ _ _ _ _ _ _ _ _ _ _ _ _ _ _ _ _ _ _ _ _ _ _ _ _ _ _ _ _ _ _ _ _ _ _ _ _ _ _ _ _ _ _ _ _ _ _ _] -> w1058
            frame "Start1", Default {
            }
            frame "Start2" {
            }
            frame "Start3" {
            }
            frame "saveSettings1" {
              n603 = call "myRIO_BRig_RT_dataExp_Audio_freq__L.vi"() -> ("output_Audio_freq__L"=w1264:i32)  [unwired: 11 in]
              n604 = call "myRIO_BRig_RT_dataExp_Audio_freq__R.vi"() -> ("output_Audio_freq__R"=w1263:i32)  [unwired: 11 in]
              n605 = call "myRIO_BRig_RT_dataExp_Audio_amp__L.vi"() -> ("output_Audio_amp__L"=w1262:i32)  [unwired: 11 in]
              n606 = call "myRIO_BRig_RT_dataExp_Audio_amp__R.vi"() -> ("output_Audio_amp__R"=w1260:i32)  [unwired: 11 in]
              n607 = call "myRIO_BRig_RT_dataExp_TPB_min__L.vi"() -> ("output_TPB_min__L"=w1272:i32)  [unwired: 11 in]
              n608 = call "myRIO_BRig_RT_dataExp_TPB_min__R.vi"() -> ("output_TPB_min__R"=w1270:i32)  [unwired: 11 in]
              n609 = call "myRIO_BRig_RT_dataExp_TPB_max__L.vi"() -> ("output_TPB_max__L"=w1268:i32)  [unwired: 11 in]
              n610 = call "myRIO_BRig_RT_dataExp_TPB_max__R.vi"() -> ("output_TPB_max__R"=w1266:i32)  [unwired: 11 in]
              n611 = call "myRIO_BRig_RT_dataExp_ItrialUntilReward.vi"() -> ("output_I_trialUntilReward"=w1285:i32)  [unwired: 11 in]
              n612 = call "myRIO_BRig_RT_dataExp_IblockUntilReward.vi"() -> ("output_I_blockUntilReward"=w1281:i32)  [unwired: 11 in]
              n613 = call "myRIO_BRig_RT_dataExp_CueCycles.vi"() -> ("output_CueCycles"=w1280:i32)  [unwired: 11 in]
              n614 = call "myRIO_BRig_RT_dataExp_ENL_min.vi"() -> ("output_ENL_min"=w1278:i32)  [unwired: 11 in]
              n615 = call "myRIO_BRig_RT_dataExp_ENL_max.vi"() -> ("output_ENL_max"=w1276:i32)  [unwired: 11 in]
              n616 = call "myRIO_BRig_RT_dataExp_ENL_penalty.vi"() -> ("output_ENL_penalty"=w1274:i32)  [unwired: 11 in]
              n617 = local read "Audio_Freq__L"() -> (w1238:u8)
              n618 = local read "Audio_Freq__R"() -> (w1236:u8)
              n619 = local read "Audio_Amp__L"() -> (w1261:u16)
              n620 = local read "TpB_Min_L"() -> (w1271:u16)
              n621 = local read "TpB_Min_R"() -> (w1269:u16)
              n622 = local read "TpB_Max_L"() -> (w1267:u16)
              n623 = local read "TpB_Max_R"() -> (w1265:u16)
              n624 = local read "Audio_Amp__R"() -> (w1259:u16)
              n625 = local read "TrialUntilReward"() -> (w1284:bool)
              n626 = local read "CueCycles"() -> (w1279:u16)
              n627 = local read "Tcycle_ENL_min"() -> (w1277:u16)
              n628 = local read "Tcycle_ENL_max"() -> (w1275:u16)
              n629 = local read "Tcycle_ENLPenalty"() -> (w1273:u16)
              n630 = To Unsigned Word Integer(number=w1236) -> (unsigned 16bit integer=w1235:u16)
              n631 = To Unsigned Word Integer(number=w1238) -> (unsigned 16bit integer=w1237:u16)
              n632 = Boolean To (0,1)(Boolean=w1284) -> (0, 1=w1283:i16)
              n633 = To Unsigned Word Integer(number=w1283) -> (unsigned 16bit integer=w1282:u16)
              n634 = local read "BUR_min"() -> (w1253:u16)
              n635 = local read "BUR_max"() -> (w1254:u16)
              n636 = Not Equal To 0?(x=w1253) -> (x != 0?=w1252:bool)
              n637 = Not Equal To 0?(x=w1254) -> (x != 0?=w1251:bool)
              n638 = And(x=w1252, y=w1251) -> (x .and. y?=w1250:bool)
              n639 = Boolean To (0,1)(Boolean=w1250) -> (0, 1=w1255:i16)
              n640 = To Unsigned Word Integer(number=w1255) -> (unsigned 16bit integer=w1249:u16)
              n641 = Replace Array Subset(array=w1287, new element #1=w1282, index #1=w1285, new element #2=w1249, index #2=w1281, new element #3=w1279, index #3=w1280, new element #4=w1277, index #4=w1278, new element #5=w1275, index #5=w1276, new element #6=w1273, index #6=w1274, new element #7=w1271, index #7=w1272, new element #8=w1269, index #8=w1270, new element #9=w1267, index #9=w1268, new element #10=w1265, index #10=w1266, new element #11=w1237, index #11=w1264, new element #12=w1235, index #12=w1263, new element #13=w1261, index #13=w1262, new element #14=w1259, index #14=w1260) -> (w1286:u16[])
            }
            frame "saveSettings2" {
              n642 = call "myRIO_BRig_RT_dataExp_Tcycle_RewardPost.vi"() -> ("output_Tcycle_RewardPost"=w1324:i32)  [unwired: 11 in]
              n643 = call "myRIO_BRig_RT_dataExp_Tcycle_Wrong.vi"() -> ("output_Tcycle_Wrong"=w1322:i32)  [unwired: 11 in]
              n644 = call "myRIO_BRig_RT_dataExp_Tcycle_Timeout.vi"() -> ("output_Tcycle_Timeout"=w1320:i32)  [unwired: 11 in]
              n645 = call "myRIO_BRig_RT_dataExp_Tcycle_Cue_min.vi"() -> ("output_Tcycle_Cue_min"=w1318:i32)  [unwired: 11 in]
              n646 = call "myRIO_BRig_RT_dataExp_Tcycle_Cue_max.vi"() -> ("output_Tcycle_Cue_max"=w1317:i32)  [unwired: 11 in]
              n647 = call "myRIO_BRig_RT_dataExp_Tcycle_CuePenalty.vi"() -> ("output_Tcycle_CuePenalty"=w1316:i32)  [unwired: 11 in]
              n648 = call "myRIO_BRig_RT_dataExp_SolenoidProbability_L.vi"() -> ("output_SolenoidProbability_L"=w1296:i32)  [unwired: 11 in]
              n649 = call "myRIO_BRig_RT_dataExp_SolenoidProbability_R.vi"() -> ("output_SolenoidProbability_R"=w1295:i32)  [unwired: 11 in]
              n650 = call "myRIO_BRig_RT_dataExp_nBlock.vi"() -> ("output_nBlock"=w1333:i32)  [unwired: 11 in]
              n651 = call "myRIO_BRig_RT_dataExp_nTrial.vi"() -> ("output_nTrial"=w1332:i32)  [unwired: 11 in]
              n652 = call "myRIO_BRig_RT_dataExp_runTime_seconds.vi"() -> ("output_RunTime_minutes"=w1331:i32)  [unwired: 11 in]
              n653 = call "myRIO_BRig_RT_dataExp_Tcycle_Selection.vi"() -> ("output_Tcycle_Selection"=w1330:i32)  [unwired: 11 in]
              n654 = call "myRIO_BRig_RT_dataExp_Tcycle_Reward__L.vi"() -> ("output_Tcycle_Reward__L"=w1328:i32)  [unwired: 11 in]
              n655 = call "myRIO_BRig_RT_dataExp_Tcycle_Reward__R.vi"() -> ("output_Tcycle_Reward__R"=w1326:i32)  [unwired: 11 in]
              n656 = local read "Tcycle_RewardPost"() -> (w1323:u16)
              n657 = local read "Tcycle_Wrong"() -> (w1321:u16)
              n658 = local read "Tcycle_Timeout"() -> (w1319:u16)
              n659 = local read "Tcycle_CuePenalty"() -> (w1309:u16)
              n660 = local read "Tcycle_Cue_max"() -> (w1297:u16)
              n661 = local read "Tcycle_Cue_min"() -> (w1298:u16)
              n662 = local read "Tcycle_Selection"() -> (w1329:u16)
              n663 = local read "Tcycle_Reward_L"() -> (w1327:u16)
              n664 = local read "Tcycle_Reward_R"() -> (w1325:u16)
              n665 = local read "SolenoidProbability_R"() -> (w1293:u16)
              n666 = local read "SolenoidProbability_L"() -> (w1294:u16)
              n667 = Replace Array Subset(array=w1335, new element #1=u16 0, index #1=w1333, new element #2=u16 0, index #2=w1332, new element #3=u16 0, index #3=w1331, new element #4=w1329, index #4=w1330, new element #5=w1327, index #5=w1328, new element #6=w1325, index #6=w1326, new element #7=w1323, index #7=w1324, new element #8=w1321, index #8=w1322, new element #9=w1319, index #9=w1320, new element #10=w1298, index #10=w1318, new element #11=w1297, index #11=w1317, new element #12=w1309, index #12=w1316, new element #13=w1294, index #13=w1296, new element #14=w1293, index #14=w1295) -> (w1334:u16[])
            }
            frame "saveSettings3" {
              w1345 = 100.0 ("y")
              n668 = call "myRIO_BRig_RT_dataExp_laser_Freq.vi"() -> ("output_laser_Freq"=w1378:i32)  [unwired: 11 in]
              n669 = call "myRIO_BRig_RT_dataExp_laser_Tpeak.vi"() -> ("output_laser_Tpeak"=w1373:i32)  [unwired: 11 in]
              n670 = call "myRIO_BRig_RT_dataExp_laser_Tshutter.vi"() -> ("output_laser_Tshutter"=w1368:i32)  [unwired: 11 in]
              n671 = call "myRIO_BRig_RT_dataExp_laser_f_millisec2count.vi"() -> ("output_laser_f_millisec2count"=w1363:i32)  [unwired: 11 in]
              n672 = call "myRIO_BRig_RT_dataExp_laser_Power_min.vi"() -> ("output_laser_Power_min"=w1358:i32)  [unwired: 11 in]
              n673 = call "myRIO_BRig_RT_dataExp_laser_Power_max.vi"() -> ("output_laser_Power_max"=w1351:i32)  [unwired: 11 in]
              n674 = call "myRIO_BRig_RT_dataExp_laser_Power_step.vi"() -> ("output_laser_Power_step"=w1350:i32)  [unwired: 11 in]
              n675 = call "myRIO_BRig_RT_dataExp_laser_duration.vi"() -> ("output_laser_duration"=w1353:i32)  [unwired: 11 in]
              n676 = call "myRIO_BRig_RT_dataExp_BUR_min.vi"() -> ("output_BUR_min"=w1400:i32)  [unwired: 11 in]
              n677 = call "myRIO_BRig_RT_dataExp_BUR_max.vi"() -> ("output_BUR_max"=w1398:i32)  [unwired: 11 in]
              n678 = call "myRIO_BRig_RT_dataExp_Audio_sp__L.vi"() -> ("output_Audio_sp__L"=w1395:i32)  [unwired: 11 in]
              n679 = call "myRIO_BRig_RT_dataExp_Audio_sp__R.vi"() -> ("output_Audio_sp__R"=w1394:i32)  [unwired: 11 in]
              n680 = local read "laser_Tshutter"() -> (w1365:dbl)
              n681 = local read "f_millisec2count"() -> (w1360:dbl)
              n682 = local read "laser_Tpeak"() -> (w1370:dbl)
              n683 = local read "laser_power_min"() -> (w1355:dbl)
              n684 = local read "laser_power_max"() -> (w1344:dbl)
              n685 = local read "laser_power_step"() -> (w1343:dbl)
              n686 = local read "laser_Freq"() -> (w1377:dbl)
              n687 = local read "sp_LeftSpout"() -> (w1393:u16)
              n688 = local read "BUR_max"() -> (w1397:u16)
              n689 = local read "sp_RightSpout"() -> (w1392:u16)
              n690 = local read "BUR_min"() -> (w1399:u16)
              n691 = Multiply(x=w1377, y=w1345) -> (x*y=w1376:dbl)
              n692 = Multiply(x=w1370, y=w1345) -> (x*y=w1372:dbl)
              n693 = Multiply(x=w1365, y=w1345) -> (x*y=w1367:dbl)
              n694 = Multiply(x=w1360, y=w1345) -> (x*y=w1362:dbl)
              n695 = Multiply(x=w1355, y=w1345) -> (x*y=w1357:dbl)
              n696 = Multiply(x=w1344, y=w1345) -> (x*y=w1349:dbl)
              n697 = Multiply(x=w1343, y=w1345) -> (x*y=w1347:dbl)
              n698 = Round To Nearest(number=w1376) -> (nearest integer value=w1375:dbl)
              n699 = Round To Nearest(number=w1372) -> (nearest integer value=w1371:dbl)
              n700 = Round To Nearest(number=w1367) -> (nearest integer value=w1366:dbl)
              n701 = Round To Nearest(number=w1362) -> (nearest integer value=w1361:dbl)
              n702 = Round To Nearest(number=w1357) -> (nearest integer value=w1356:dbl)
              n703 = Round To Nearest(number=w1349) -> (nearest integer value=w1348:dbl)
              n704 = Round To Nearest(number=w1347) -> (nearest integer value=w1346:dbl)
              n705 = To Unsigned Word Integer(number=w1375) -> (unsigned 16bit integer=w1374:u16)
              n706 = To Unsigned Word Integer(number=w1371) -> (unsigned 16bit integer=w1369:u16)
              n707 = To Unsigned Word Integer(number=w1366) -> (unsigned 16bit integer=w1364:u16)
              n708 = To Unsigned Word Integer(number=w1361) -> (unsigned 16bit integer=w1359:u16)
              n709 = To Unsigned Word Integer(number=w1356) -> (unsigned 16bit integer=w1354:u16)
              n710 = To Unsigned Word Integer(number=w1348) -> (unsigned 16bit integer=w1342:u16)
              n711 = To Unsigned Word Integer(number=w1346) -> (unsigned 16bit integer=w1341:u16)
              n712 = local read "laser_duration"() -> (w1352:u16)
              n713 = call "myRIO_BRig_RT_dataCurrent_LaserPulse_duration.vi"() -> ("output_LaserPulse_duration"=w1379:i32)  [unwired: 11 in]
              n714 = Replace Array Subset(array=w1401, new element #1=w1399, index #1=w1400, new element #2=w1397, index #2=w1398, new element #3=w1393, index #3=w1395, new element #4=w1392, index #4=w1394, new element #5=w1374, index #5=w1378, new element #6=w1369, index #6=w1373, new element #7=w1364, index #7=w1368, new element #8=w1359, index #8=w1363, new element #9=w1354, index #9=w1358, new element #10=w1342, index #10=w1351, new element #11=w1341, index #11=w1350, new element #12=w1352, index #12=w1353) -> (w1396:u16[])
              n715 = Replace Array Subset(array=w1381, new element=w1352, index=w1379) -> (w1380:u16[])
            }
            frame "saveSettings4_LC_ENL" {
              # "delayOpt"
              # "Count"
              # "Tdelay"
              # "Probability"
              # "OnOff"
              # "Block"
              # "ENL1 All"
              # "delayOpt"
              # "Count"
              # "Tdelay"
              # "Probability"
              # "OnOff"
              # "Block"
              # "ENL1 First"
              n716 = call "myRIO_BRig_RT_dataLC_ENL1_All_Block.vi"() -> ("output_ENL1_All_Block"=w1424:i32)  [unwired: 11 in]
              n717 = call "myRIO_BRig_RT_dataLC_ENL1_All_OnOff.vi"() -> ("output_ENL1_All_OnOff"=w1413:i32)  [unwired: 11 in]
              n718 = call "myRIO_BRig_RT_dataLC_ENL1_All_Probability.vi"() -> ("output_ENL1_All_Probability"=w1412:i32)  [unwired: 11 in]
              n719 = call "myRIO_BRig_RT_dataLC_ENL1_All_Tdelay.vi"() -> ("output_ENL1_All_Tdelay"=w1411:i32)  [unwired: 11 in]
              n720 = call "myRIO_BRig_RT_dataLC_ENL1_All_Count.vi"() -> ("output_ENL1_All_Count"=w1410:i32)  [unwired: 11 in]
              n721 = call "myRIO_BRig_RT_dataLC_ENL1_All_delayOpt.vi"() -> ("output_ENL1_All_delayOpt"=w1409:i32)  [unwired: 11 in]
              n722 = call "myRIO_BRig_RT_dataLC_ENL1_First_Block.vi"() -> ("output_ENL1_First_Block"=w1450:i32)  [unwired: 11 in]
              n723 = call "myRIO_BRig_RT_dataLC_ENL1_First_OnOff.vi"() -> ("output_ENL1_First_OnOff"=w1448:i32)  [unwired: 11 in]
              n724 = call "myRIO_BRig_RT_dataLC_ENL1_First_Probability.vi"() -> ("output_ENL1_First_Probability"=w1444:i32)  [unwired: 11 in]
              n725 = call "myRIO_BRig_RT_dataLC_ENL1_First_Tdelay.vi"() -> ("output_ENL1_First_Tdelay"=w1442:i32)  [unwired: 11 in]
              n726 = call "myRIO_BRig_RT_dataLC_ENL1_First_Count.vi"() -> ("output_ENL1_First_Count"=w1440:i32)  [unwired: 11 in]
              n727 = call "myRIO_BRig_RT_dataLC_ENL1_First_delayOpt.vi"() -> ("output_ENL1_First_delayOpt"=w1426:i32)  [unwired: 11 in]
              n728 = local read "LC_ENL1_First_delayOpt"() -> (w1427:bool)
              n729 = local read "LC_ENL1_First_Count"() -> (w1439:u16)
              n730 = local read "LC_ENL1_First_Probability"() -> (w1443:u16)
              n731 = local read "LC_ENL1_First_Block"() -> (w1449:u16)
              n732 = local read "LC_ENL1_First_Tdelay"() -> (w1441:u16)
              n733 = local read "LC_ENL1_First_OnOff"() -> (w1447:bool)
              n734 = local read "LC_ENL1_All_OnOff"() -> (w1420:bool)
              n735 = local read "LC_ENL1_All_Probability"() -> (w1418:u16)
              n736 = local read "LC_ENL1_All_delayOpt"() -> (w1415:bool)
              n737 = local read "LC_ENL1_All_Tdelay"() -> (w1417:u16)
              n738 = local read "LC_ENL1_All_Block"() -> (w1421:u16)
              n739 = local read "LC_ENL1_All_Count"() -> (w1416:u16)
              n740 = Boolean To (0,1)(Boolean=w1427) -> (0, 1=w1428:i16)
              n741 = Boolean To (0,1)(Boolean=w1447) -> (0, 1=w1446:i16)
              n742 = Boolean To (0,1)(Boolean=w1420) -> (0, 1=w1423:i16)
              n743 = To Unsigned Word Integer(number=w1428) -> (unsigned 16bit integer=w1425:u16)
              n744 = To Unsigned Word Integer(number=w1446) -> (unsigned 16bit integer=w1445:u16)
              n745 = Boolean To (0,1)(Boolean=w1415) -> (0, 1=w1422:i16)
              n746 = To Unsigned Word Integer(number=w1423) -> (unsigned 16bit integer=w1419:u16)
              n747 = To Unsigned Word Integer(number=w1422) -> (unsigned 16bit integer=w1414:u16)
              n748 = Replace Array Subset(array=w1451, new element #1=w1449, index #1=w1450, new element #2=w1445, index #2=w1448, new element #3=w1443, index #3=w1444, new element #4=w1441, index #4=w1442, new element #5=w1439, index #5=w1440, new element #6=w1425, index #6=w1426, new element #7=w1421, index #7=w1424, new element #8=w1419, index #8=w1413, new element #9=w1418, index #9=w1412, new element #10=w1417, index #10=w1411, new element #11=w1416, index #11=w1410, new element #12=w1414, index #12=w1409) -> (w1452:u16[])
            }
            frame "saveSettings5_LC_Cue" {
              # "delayOpt"
              # "Count"
              # "Tdelay"
              # "Probability"
              # "OnOff"
              # "Block"
              # "Cue1 All"
              # "delayOpt"
              # "Count"
              # "Tdelay"
              # "Probability"
              # "OnOff"
              # "Block"
              # "Cue1 First"
              n749 = call "myRIO_BRig_RT_dataLC_Cue1_First_delayOpt.vi"() -> ("output_Cue1_First_delayOpt"=w1479:i32)  [unwired: 11 in]
              n750 = call "myRIO_BRig_RT_dataLC_Cue1_First_Block.vi"() -> ("output_Cue1_First_Block"=w1502:i32)  [unwired: 11 in]
              n751 = call "myRIO_BRig_RT_dataLC_Cue1_First_OnOff.vi"() -> ("output_Cue1_First_OnOff"=w1500:i32)  [unwired: 11 in]
              n752 = call "myRIO_BRig_RT_dataLC_Cue1_First_Probability.vi"() -> ("output_Cue1_First_Probability"=w1496:i32)  [unwired: 11 in]
              n753 = call "myRIO_BRig_RT_dataLC_Cue1_First_Tdelay.vi"() -> ("output_Cue1_First_Tdelay"=w1494:i32)  [unwired: 11 in]
              n754 = call "myRIO_BRig_RT_dataLC_Cue1_First_Count.vi"() -> ("output_Cue1_First_Count"=w1492:i32)  [unwired: 11 in]
              n755 = call "myRIO_BRig_RT_dataLC_Cue1_All_Block.vi"() -> ("output_Cue1_All_Block"=w1476:i32)  [unwired: 11 in]
              n756 = call "myRIO_BRig_RT_dataLC_Cue1_All_OnOff.vi"() -> ("output_Cue1_All_OnOff"=w1475:i32)  [unwired: 11 in]
              n757 = call "myRIO_BRig_RT_dataLC_Cue1_All_Probability.vi"() -> ("output_Cue1_All_Probability"=w1474:i32)  [unwired: 11 in]
              n758 = call "myRIO_BRig_RT_dataLC_Cue1_All_Tdelay.vi"() -> ("output_Cue1_All_Tdelay"=w1473:i32)  [unwired: 11 in]
              n759 = call "myRIO_BRig_RT_dataLC_Cue1_All_Count.vi"() -> ("output_Cue1_All_Count"=w1472:i32)  [unwired: 11 in]
              n760 = call "myRIO_BRig_RT_dataLC_Cue1_All_delayOpt.vi"() -> ("output_Cue1_All_delayOpt"=w1471:i32)  [unwired: 11 in]
              n761 = local read "LC_Cue1_First_delayOpt"() -> (w1478:bool)
              n762 = local read "LC_Cue1_First_Count"() -> (w1491:u16)
              n763 = local read "LC_Cue1_First_Probability"() -> (w1495:u16)
              n764 = local read "LC_Cue1_First_Block"() -> (w1501:u16)
              n765 = local read "LC_Cue1_First_Tdelay"() -> (w1493:u16)
              n766 = local read "LC_Cue1_First_OnOff"() -> (w1499:bool)
              n767 = local read "LC_Cue1_All_OnOff"() -> (w1467:bool)
              n768 = local read "LC_Cue1_All_delayOpt"() -> (w1468:bool)
              n769 = local read "LC_Cue1_All_Probability"() -> (w1464:u16)
              n770 = local read "LC_Cue1_All_Tdelay"() -> (w1463:u16)
              n771 = local read "LC_Cue1_All_Count"() -> (w1462:u16)
              n772 = local read "LC_Cue1_All_Block"() -> (w1466:u16)
              n773 = Boolean To (0,1)(Boolean=w1478) -> (0, 1=w1480:i16)
              n774 = Boolean To (0,1)(Boolean=w1499) -> (0, 1=w1498:i16)
              n775 = Boolean To (0,1)(Boolean=w1467) -> (0, 1=w1470:i16)
              n776 = To Unsigned Word Integer(number=w1480) -> (unsigned 16bit integer=w1477:u16)
              n777 = To Unsigned Word Integer(number=w1498) -> (unsigned 16bit integer=w1497:u16)
              n778 = To Unsigned Word Integer(number=w1470) -> (unsigned 16bit integer=w1465:u16)
              n779 = Boolean To (0,1)(Boolean=w1468) -> (0, 1=w1469:i16)
              n780 = To Unsigned Word Integer(number=w1469) -> (unsigned 16bit integer=w1461:u16)
              n781 = Replace Array Subset(array=w1503, new element #1=w1501, index #1=w1502, new element #2=w1497, index #2=w1500, new element #3=w1495, index #3=w1496, new element #4=w1493, index #4=w1494, new element #5=w1491, index #5=w1492, new element #6=w1477, index #6=w1479, new element #7=w1466, index #7=w1476, new element #8=w1465, index #8=w1475, new element #9=w1464, index #9=w1474, new element #10=w1463, index #10=w1473, new element #11=w1462, index #11=w1472, new element #12=w1461, index #12=w1471) -> (w1504:u16[])
            }
            frame "saveSettings6_LC_Other" {
              # "Trial"
              # "Tdelay"
              # "Probability"
              # "OnOff"
              # "Block"
              # "Wrong"
              # "Trial"
              # "Tdelay"
              # "Probability"
              # "OnOff"
              # "Block"
              # "Reward"
              n782 = call "myRIO_BRig_RT_dataLC_Wrong_Block.vi"() -> ("output_Wrong_Block"=w1534:i32)  [unwired: 11 in]
              n783 = call "myRIO_BRig_RT_dataLC_Wrong_OnOff.vi"() -> ("output_Wrong_OnOff"=w1533:i32)  [unwired: 11 in]
              n784 = call "myRIO_BRig_RT_dataLC_Wrong_Probability.vi"() -> ("output_Wrong_Probability"=w1532:i32)  [unwired: 11 in]
              n785 = call "myRIO_BRig_RT_dataLC_Wrong_Tdelay.vi"() -> ("output_Wrong_Tdelay"=w1531:i32)  [unwired: 11 in]
              n786 = call "myRIO_BRig_RT_dataLC_Wrong_Trial.vi"() -> ("output_Wrong_Trial"=w1530:i32)  [unwired: 11 in]
              n787 = call "myRIO_BRig_RT_dataLC_Reward_Block.vi"() -> ("output_Reward_Block"=w1546:i32)  [unwired: 11 in]
              n788 = call "myRIO_BRig_RT_dataLC_Reward_OnOff.vi"() -> ("output_Reward_OnOff"=w1544:i32)  [unwired: 11 in]
              n789 = call "myRIO_BRig_RT_dataLC_Reward_Probability.vi"() -> ("output_Reward_Probability"=w1540:i32)  [unwired: 11 in]
              n790 = call "myRIO_BRig_RT_dataLC_Reward_Tdelay.vi"() -> ("output_Reward_Tdelay"=w1538:i32)  [unwired: 11 in]
              n791 = call "myRIO_BRig_RT_dataLC_Reward_Trial.vi"() -> ("output_Reward_Trial"=w1536:i32)  [unwired: 11 in]
              n792 = local read "LC_Wrong_OnOff"() -> (w1528:bool)
              n793 = local read "LC_Wrong_Probability"() -> (w1525:u16)
              n794 = local read "LC_Wrong_Block"() -> (w1527:u16)
              n795 = local read "LC_Wrong_Tdelay"() -> (w1524:u16)
              n796 = local read "LC_Wrong_Trial"() -> (w1523:u16)
              n797 = local read "LC_Reward_Probability"() -> (w1539:u16)
              n798 = local read "LC_Reward_Block"() -> (w1545:u16)
              n799 = local read "LC_Reward_Tdelay"() -> (w1537:u16)
              n800 = local read "LC_Reward_OnOff"() -> (w1543:bool)
              n801 = local read "LC_Reward_Trial"() -> (w1535:u16)
              n802 = Boolean To (0,1)(Boolean=w1528) -> (0, 1=w1529:i16)
              n803 = Boolean To (0,1)(Boolean=w1543) -> (0, 1=w1542:i16)
              n804 = To Unsigned Word Integer(number=w1529) -> (unsigned 16bit integer=w1526:u16)
              n805 = To Unsigned Word Integer(number=w1542) -> (unsigned 16bit integer=w1541:u16)
              n806 = Replace Array Subset(array=w1547, new element #1=w1545, index #1=w1546, new element #2=w1541, index #2=w1544, new element #3=w1539, index #3=w1540, new element #4=w1537, index #4=w1538, new element #5=w1535, index #5=w1536, new element #6=w1527, index #6=w1534, new element #7=w1526, index #7=w1533, new element #8=w1525, index #8=w1532, new element #9=w1524, index #9=w1531, new element #10=w1523, index #10=w1530) -> (w1548:u16[])
            }
            frame "setSettings_Audio" {
              # "amp_L"
              # "amp_R"
              # "freq_L"
              # "freq_R"
              n807 = call "myRIO_BRig_RT_dataExp_Audio_amp__L.vi"() -> ("output_Audio_amp__L"=w1573:i32)  [unwired: 11 in]
              n808 = call "myRIO_BRig_RT_dataExp_Audio_amp__R.vi"() -> ("output_Audio_amp__R"=w1572:i32)  [unwired: 11 in]
              n809 = call "myRIO_BRig_RT_dataExp_Audio_freq__L.vi"() -> ("output_Audio_freq__L"=w1571:i32)  [unwired: 11 in]
              n810 = call "myRIO_BRig_RT_dataExp_Audio_freq__R.vi"() -> ("output_Audio_freq__R"=w1570:i32)  [unwired: 11 in]
              n811 = Index Array(array=w1569, index #1=w1573, index #2=w1572, index #3=w1571, index #4=w1570) -> (element #1=w1568:u16, element #2=w1567:u16, element #3=w1560:u16, element #4=w1558:u16)
              n812 = To Unsigned Byte Integer(number=w1560) -> (unsigned 8bit integer=w1559:u8)
              n813 = To Unsigned Byte Integer(number=w1558) -> (unsigned 8bit integer=w1557:u8)
            }
            frame "setSettings_Laser" {
              (unwired) u32 0 ("tDelay_laser_rew")
              # "Wrong tDelay"
              # "Reward tDelay"
              n814 = call "myRIO_BRig_RT_dataLC_Reward_Tdelay.vi"() -> ("output_Reward_Tdelay"=w1600:i32)  [unwired: 11 in]
              n815 = call "myRIO_BRig_RT_dataLC_Wrong_Tdelay.vi"() -> ("output_Wrong_Tdelay"=w1601:i32)  [unwired: 11 in]
              n816 = Index Array(array=w1597, index #1=w1600, index #2=w1601) -> (element #1=w1599:u16, element #2=w1598:u16)
              n817 = call "myRIO_BRig_RT__calc_Tvalley.vi"("input_peakWidth"="laser_Tpeak", "input_freq"="laser_Freq") -> ("output_Tvalley"=w1607:dbl)  [unwired: 9 in]
              n818 = To Double Precision Float(number=w1599) -> (double precision float=w1594:dbl)
              n819 = To Double Precision Float(number=w1598) -> (double precision float=w1591:dbl)
              n820 = Multiply(x="f_millisec2count", y="laser_Tpeak") -> (x*y=w1616:dbl)
              n821 = Multiply(x="f_millisec2count", y=w1607) -> (x*y=w1613:dbl)
              n822 = Multiply(x="f_millisec2count", y="laser_Tshutter") -> (x*y=w1611:dbl)
              n823 = Round Toward +Infinity(x="laser_Tshutter") -> (ceil(x): smallest int >= x=w1602:dbl)
              n824 = Multiply(x="f_millisec2count", y=w1594) -> (x*y=w1595:dbl)
              n825 = Multiply(x="f_millisec2count", y=w1591) -> (x*y=w1592:dbl)
              n826 = To Unsigned Word Integer(number="f_millisec2count") -> (unsigned 16bit integer=w1582:u16)
              n827 = Round Toward +Infinity(x=w1616) -> (ceil(x): smallest int >= x=w1617:dbl)
              n828 = Round Toward +Infinity(x=w1613) -> (ceil(x): smallest int >= x=w1614:dbl)
              n829 = Round Toward +Infinity(x=w1611) -> (ceil(x): smallest int >= x=w1606:dbl)
              n830 = Round Toward +Infinity(x=w1595) -> (ceil(x): smallest int >= x=w1596:dbl)
              n831 = Round Toward +Infinity(x=w1592) -> (ceil(x): smallest int >= x=w1593:dbl)
              n832 = To Unsigned Long Integer(number=w1617) -> (unsigned 32bit integer=w1615:u32)
              n833 = To Unsigned Long Integer(number=w1614) -> (unsigned 32bit integer=w1612:u32)
              n834 = To Unsigned Long Integer(number=w1606) -> (unsigned 32bit integer=w1610:u32)
              n835 = To Unsigned Word Integer(number=w1602) -> (unsigned 16bit integer=w1605:u16)
              n836 = To Unsigned Long Integer(number=w1596) -> (unsigned 32bit integer=w1590:u32)
              n837 = To Unsigned Long Integer(number=w1593) -> (unsigned 32bit integer=w1589:u32)
              n838 = Add(x="laser_duration", y=w1605) -> (x+y=w1586:u16)
              n839 = To Double Precision Float(number=w1586) -> (double precision float=w1585:dbl)
              n840 = Multiply(x=w1585, y="f_millisec2count") -> (x*y=w1587:dbl)
              n841 = call "myRIO_BRig_RT_dataCurrent_LaserPulse_duration.vi"() -> ("output_LaserPulse_duration"=w1618:i32)  [unwired: 11 in]
              n842 = Round Toward +Infinity(x=w1587) -> (ceil(x): smallest int >= x=w1588:dbl)
              n843 = To Unsigned Long Integer(number=w1588) -> (unsigned 32bit integer=w1584:u32)
              n844 = xnode "Read/Write Control"("FPGA VI Reference In"=w1620, "error in"=w1621, "laser_Npeak"=w1615, "laser_Nvalley"=w1612, "laser_Nshutter"=w1610, "laser_selRew_Ndelay"=w1590, "laser_selWro_NDelay"=w1589, "laser_selRew_Ntotal"=w1584, "laser_selWro_Ntotal"=w1584, "k1__counter_per_ms"=w1582) -> ("error out"=→"error out":errorcluster)  [unwired: 1 out]
              n845 = Replace Array Subset(array=w1597, new element=w1586, index=w1618) -> (w1619:u16[])
            }
            frame "initBlock" {
              n846 = call "myRIO_Brig_RT__Case_Exp_State_initBlock.vi"("input_spout"=w1665, "input_dataExp"=w1663, "input_dataCurrent"=w1664) -> ("output_spout"=w1643:enum16{"Left", "Right"}, "output_state"=w1666:T2, "output_dataExp"=w1662:u16[], "output_dataCurrent"=w1648:u16[], "output_TpB_target"=→"TpB_target":u16)  [unwired: 4 in]
              "cSpout" <- w1643
              n847 = call "myRIO_BRig_RT_dataCurrent_iBlock.vi"() -> ("output_iBlock"=w1647:i32)  [unwired: 11 in]
              n848 = Index Array(array=w1648, index=w1647) -> (element=w1641:u16)
              "iBlock" <- w1641
            }
            frame "initBlock2" {
              n849 = local write "nRewards_cur"(u16 0 ("nRewards_cur")) -> ()
              n850 = call "myRIO_BRig_RT__Case_Exp_State_initBlock2.vi"("input_spout"=w1674, "input_dataBlock"=w1675, "input_dataCurrent"=w1673) -> ("idxDataBlock"=w1670:i32, "output_dataBlock"=w1672:u16[][])  [unwired: 7 in]
            }
            frame "initTrial" {
              n851 = call "myRIO_Brig_RT__Case_Exp_State_initTrial.vi"("input_spout"=w1693, "input_dataExp"=w1709, "input_dataCurrent"=w1710) -> ("output_state"=w1711:T2, "output_dataExp"=w1708:u16[], "output_dataCurrent"=w1698:u16[])  [unwired: 6 in]
              n852 = call "myRIO_BRig_RT_dataCurrent_iTrial.vi"() -> ("output_iTrial"=w1697:i32)  [unwired: 11 in]
              n853 = call "myRIO_BRig_RT_dataCurrent_SolenoidReward.vi"() -> ("output_SolenoidReward"=w1692:i32)  [unwired: 11 in]
              n854 = Index Array(array=w1698, index #1=w1697, index #2=w1692) -> (element #1=w1688:u16, element #2=w1691:u16)
              "iTrial" <- w1688
              n855 = Not Equal To 0?(x=w1691) -> (x != 0?=→"SolenoidReward":bool)
            }
            frame "initTrial2" {
              # "trialUntilReward"
              n856 = call "myRIO_BRig_RT__Case_Exp_subState_LC__initTrial.vi"("input_dataTrial"=w1718, "input_spout"=w1727, "input_dataCurrent"=w1716, "input_dataLC"=w1715) -> ("output_LC_Wrong"=w1728:bool, "output_LC_led_Wrong"=w1720:bool, "output_LC_Reward"=w1729:bool, "output_LC_led_Reward"=w1719:bool, "output_dataTrial"=w1717:u16[][])  [unwired: 2 in]
              n857 = Equal?(x=w1727, y=enum16{"Left", "Right"}."Right") -> (x = y?=w1725:bool)
              n858 = call "myRIO_BRig_RT_dataExp_ItrialUntilReward.vi"() -> ("output_I_trialUntilReward"=w1723:i32)  [unwired: 11 in]
              n859 = Index Array(array=w1724, index=w1723) -> (element=w1722:u16)
              n860 = Not Equal To 0?(x=w1722) -> (x != 0?=w1721:bool)
              n861 = xnode "Read/Write Control"("FPGA VI Reference In"=w1742, "error in"=w1741, "SelectionState"=FALSE, "laserResponse_reward"=w1729, "laserResponse_wrong"=w1728, "laserResponse_reward_LED"=w1719, "laserResponse_wrong_LED"=w1720, "Left(F)_or_Right(T)"=w1725, "ignoreWrong"=w1721) -> ("error out"=→"error_initTrial":errorcluster)  [unwired: 1 out]
            }
            frame "initTrial3" {
              n862 = call "myRIO_BRig_RT__Case_Exp_State_initTrial_dataTrial.vi"("input_spout"=w1757, "input_dataCurrent"=w1758, "input_dataExp"=w1756, "input_dataTrial"=w1760) -> ("output_dataTrial"=w1759:u16[][], "output_laserPower"=w1753:u16)  [unwired: 6 in]
              n863 = To Double Precision Float(number=w1753) -> (double precision float=w1755:dbl)
              n864 = Divide(x=w1755, y=100.0 ("x")) -> (x/y=w1749:dbl)
              "output_PortA" <- w1749
              n865 = call "myRIO__convert__Voltage_to_FPGAvalue.vi"("input_voltage"=w1749) -> ("output_PortC"=w1748:i16)  [unwired: 9 in, 1 out]
              n866 = xnode "Read/Write Control"("FPGA VI Reference In"=w1752, "error in"=w1751, "AnaOut_0"=w1748) -> ("error out"=→"error out 4":errorcluster)  [unwired: 1 out]
            }
            frame "initTrial4" {
              n867 = call "myRIO_BRig_RT_dataCurrent_idxDataTrial.vi"() -> ("output_idxDataTrial"=w1783:i32)  [unwired: 11 in]
              n868 = call "myRIO_BRig_RT_dataTrial_activeRecording.vi"() -> ("output_activeRecording"=w1780:i32)  [unwired: 11 in]
              n869 = Index Array(array=w1785, index=w1783) -> (element=w1782:u16)
              n870 = Boolean To (0,1)(Boolean="Recording") -> (0, 1=w1779:i16)
              n871 = To Long Integer(number=w1782) -> (32bit integer=w1781:i32)
              n872 = To Unsigned Word Integer(number=w1779) -> (unsigned 16bit integer=w1778:u16)
              n873 = Replace Array Subset(array=w1784, new element=w1778, index (row)=w1781, index (col)=w1780) -> (w1777:u16[][])
            }
            frame "initTrial_LC_ENL1" {
              w1807 = TRUE ("Recording")
              n874 = call "myRIO_BRig_RT__Case_Exp_State_initTrial_LC_ENL1__v2.vi"("input_dataTrial"=w1810, "input_spout"=w1815, "input_dataBlock"=w1808, "input_dataLC"=w1816, "input_dataCurrent"=w1812) -> ("output_LC__ENL1"=w1814:bool, "output_LC_led__ENL1"=w1813:bool, "output_dataTrial"=w1809:u16[][], "output_dataCurrent"=w1811:u16[])  [unwired: 3 in]
            }
            frame "initTrial_LC_Cue1" {
              n875 = local read "Recording"() -> (w1832:bool)
              n876 = call "myRIO_BRig_RT__Case_Exp_State_initTrial_LC_Cue1__v2.vi"("input_dataTrial"=w1839, "input_spout"=w1842, "input_dataBlock"=w1837, "input_dataLC"=w1843, "input_dataCurrent"=w1841) -> ("output_LC__Cue1"=w1835:bool, "output_LC_led__Cue1"=w1836:bool, "output_dataTrial"=w1838:u16[][], "output_dataCurrent"=w1840:u16[])  [unwired: 3 in]
            }
            frame "ENL1_pre" {
              # "ENL1_n"
              # "Tcycle"
              # "counter"
              n877 = call "myRIO_BRig_RT_dataCurrent_Tcycle_generic.vi"() -> ("output_Tcycle_generic"=w1889:i32)  [unwired: 11 in]
              n878 = call "myRIO_BRig_RT_dataCurrent_count_generic.vi"() -> ("output_count_generic"=w1891:i32)  [unwired: 11 in]
              n879 = call "myRIO_BRig_RT_dataCurrent_ENL.vi"() -> ("output_ENL"=w1888:i32)  [unwired: 11 in]
              n880 = call "myRIO_BRig_RT_dataCurrent_ENL1_n.vi"() -> ("output_ENL1_n"=w1860:i32)  [unwired: 11 in]
              n881 = Index Array(array=w1882, index #1=w1888, index #2=w1860) -> (element #1=w1887:u16, element #2=w1859:u16)
              n882 = Increment(x=w1859) -> (x+1=w1858:u16)
              n883 = Replace Array Subset(array=w1882, new element #1=u16 0 ("new element/subarray"), index #1=w1891, new element #2=w1887, index #2=w1889, new element #3=w1858, index #3=w1860) -> (w1886:u16[])
              n884 = Select(t=myRIO_BRig_RT__Case_Exp_stateList."ENL1Penalty_pre" ("Enum"), s=w1870, f=myRIO_BRig_RT__Case_Exp_stateList."ENL1" ("Enum")) -> (s? t:f=w1867:T2)
            }
            frame "ENL1" {
              n885 = call "myRIO_BRig_RT__Case_Exp_State_ENL1__v2.vi"("input_LC"=w1898, "I_lick"=w1902, "input_LC_led"=w1899, 9:w1894, "input_state"=w1908, "input_dataCurrent"=w1907) -> ("output_trigger_laser_led"=w1897:bool, "output_state"=w1905:T2, "output_dataCurrent"=w1906:u16[], "output_trigger_laser"=w1896:bool)  [unwired: 2 in]
              n886 = Or(x=w1897, y=w1894) -> (x .or. y?=w1900:bool)
            }
            frame "ENL1Penalty_pre" {
              # "Tcycle"
              # "counter"
              n887 = call "myRIO_BRig_RT_dataCurrent_Tcycle_generic.vi"() -> ("output_Tcycle_generic"=w1948:i32)  [unwired: 11 in]
              n888 = call "myRIO_BRig_RT_dataCurrent_count_generic.vi"() -> ("output_count_generic"=w1950:i32)  [unwired: 11 in]
              n889 = call "myRIO_BRig_RT_dataExp_ENL_penalty.vi"() -> ("output_ENL_penalty"=w1943:i32)  [unwired: 11 in]
              n890 = Index Array(array=w1944, index=w1943) -> (element=w1947:u16)
              n891 = Replace Array Subset(array=w1945, new element #1=u16 0 ("new element/subarray"), index #1=w1950, new element #2=w1947, index #2=w1948) -> (w1946:u16[])
            }
            frame "ENL1Penalty" {
              n892 = call "myRIO_BRig_RT__Case_Exp_State_ENL1Penalty.vi"("input_state"=w1973, "input_dataCurrent"=w1977) -> ("output_state"=w1974:T2, "output_dataCurrent"=w1976:u16[])  [unwired: 8 in]
            }
            frame "ENL2_pre" {
            }
            frame "ENL2" {
            }
            frame "ENL2Penalty_pre" {
            }
            frame "ENL2Penalty" {
            }
            frame "Cue1_pre" {
              # "Cue1_n"
              # "Tcycle_Cue1"
              # "0 = L, 1 = R, 2 = both"
              # "sp_R"
              # "sp_L"
              # "Tcycle"
              # "counter"
              n893 = Equal?(x=w2088, y=enum16{"Left", "Right"}."Left") -> (x = y?=w2087:bool)
              n894 = call "myRIO_BRig_RT_dataExp_Audio_sp__L.vi"() -> ("output_Audio_sp__L"=w2086:i32)  [unwired: 11 in]
              n895 = call "myRIO_BRig_RT_dataExp_Audio_sp__R.vi"() -> ("output_Audio_sp__R"=w2085:i32)  [unwired: 11 in]
              n896 = call "myRIO_BRig_RT_dataCurrent_Tcycle_generic.vi"() -> ("output_Tcycle_generic"=w2098:i32)  [unwired: 11 in]
              n897 = call "myRIO_BRig_RT_dataCurrent_count_generic.vi"() -> ("output_count_generic"=w2100:i32)  [unwired: 11 in]
              n898 = Select(t=w2086, s=w2087, f=w2085) -> (s? t:f=w2084:i32)
              n899 = call "myRIO_BRig_RT_dataCurrent_Cue1_n.vi"() -> ("output_Cue1_n"=w2062:i32)  [unwired: 11 in]
              n900 = call "myRIO_BRig_RT_dataCurrent_Tcycle_cue.vi"() -> ("output_Tcycle_cue"=w2071:i32)  [unwired: 11 in]
              n901 = Index Array(array=w2090, index=w2084) -> (element=w2082:u16)
              n902 = Index Array(array=w2072, index #1=w2071, index #2=w2062) -> (element #1=w2073:u16, element #2=w2064:u16)
              n903 = Increment(x=w2064) -> (x+1=w2063:u16)
              n904 = Not Equal To 0?(x=w2082) -> (x != 0?=w2080:bool)
              n905 = Not Equal?(x=w2082, y=u16 1) -> (x != y?=w2081:bool)
              n906 = Replace Array Subset(array=w2072, new element #1=u16 0 ("new element/subarray"), index #1=w2100, new element #2=w2073, index #2=w2098, new element #3=w2063, index #3=w2062) -> (w2097:u16[])
              n907 = Select(t=myRIO_BRig_RT__Case_Exp_stateList."Cue1Penalty_pre" ("Enum"), s=w2068, f=myRIO_BRig_RT__Case_Exp_stateList."Cue1" ("Enum")) -> (s? t:f=w2069:T2)
            }
            frame "Cue1" {
              n908 = call "myRIO_BRig_RT__Case_Exp_State_Cue1__v2.vi"("input_LC"=w2110, "I_lick"=w2113, "input_LC_led"=w2111, 9:w2105, "input_state"=w2115, "input_dataCurrent"=w2133) -> ("output_trigger_laser_led"=w2108:bool, "output_state"=w2114:T2, "output_dataCurrent"=w2132:u16[], "output_trigger_laser"=w2109:bool)  [unwired: 2 in]
              n909 = Or(x=w2108, y=w2105) -> (x .or. y?=w2107:bool)
              n910 = Equal?(x=myRIO_BRig_RT__Case_Exp_stateList."Selection_pre", y=w2114) -> (x = y?=w2118:bool)
              n911 = xnode "Read/Write Control"("FPGA VI Reference In"=w2117, "error in"=w2116, "SelectionState"=w2118) -> ()  [unwired: 2 out]
            }
            frame "Cue1Penalty_pre" {
              # "Tcycle"
              # "counter"
              n912 = call "myRIO_BRig_RT_dataCurrent_Tcycle_generic.vi"() -> ("output_Tcycle_generic"=w2164:i32)  [unwired: 11 in]
              n913 = call "myRIO_BRig_RT_dataCurrent_count_generic.vi"() -> ("output_count_generic"=w2166:i32)  [unwired: 11 in]
              n914 = call "myRIO_BRig_RT_dataExp_Tcycle_CuePenalty.vi"() -> ("output_Tcycle_CuePenalty"=w2163:i32)  [unwired: 11 in]
              n915 = Index Array(array=w2158, index=w2163) -> (element=w2162:u16)
              n916 = Replace Array Subset(array=w2160, new element #1=u16 0 ("new element/subarray"), index #1=w2166, new element #2=w2162, index #2=w2164) -> (w2159:u16[])
            }
            frame "Cue1Penalty" {
              # "reset laserOccurred"
              n917 = call "myRIO_BRig_RT__Case_Exp_State_Cue1Penalty.vi"("input_state"=w2190, "input_dataCurrent"=w2191) -> ("output_state"=w2188:T2, "output_dataCurrent"=w2189:u16[])  [unwired: 8 in]
            }
            frame "Cue2_pre" {
              n918 = call "myRIO_BRig_RT__Case_Exp_subState_LC__Cue2.vi"("input_spout"=w2208, "input_dataCurrent"=w2209, "input_dataLC"=w2207) -> ()  [unwired: 6 in, 2 out]
            }
            frame "Cue2" {
            }
            frame "Cue2Penalty_pre" {
            }
            frame "Cue2Penalty" {
            }
            frame "Selection_pre" {
              # "Tcycle"
              # "counter"
              n919 = xnode "Read/Write Control"("FPGA VI Reference In"=w2280, "error in"=w2281) -> ("error out"=→"error_Selection_pre":errorcluster, "SelectReward"=w2273:bool, "SelectWrong"=w2275:bool)  [unwired: 1 out]
              n920 = call "myRIO_BRig_RT_dataCurrent_Tcycle_generic.vi"() -> ("output_Tcycle_generic"=w2302:i32)  [unwired: 11 in]
              n921 = call "myRIO_BRig_RT_dataCurrent_count_generic.vi"() -> ("output_count_generic"=w2304:i32)  [unwired: 11 in]
              n922 = call "myRIO_BRig_RT_dataExp_Tcycle_Selection.vi"() -> ("output_Tcycle_Selection"=w2301:i32)  [unwired: 11 in]
              n923 = Index Array(array=w2298, index=w2301) -> (element=w2300:u16)
              n924 = Replace Array Subset(array=w2296, new element #1=u16 0 ("new element/subarray"), index #1=w2304, new element #2=w2300, index #2=w2302) -> (w2299:u16[])
              n925 = Or(x=w2273, y=w2275) -> (x .or. y?=w2274:bool)
              n926 = Select(t=myRIO_BRig_RT__Case_Exp_stateList."SelectReward_pre" ("Enum"), s=w2273, f=myRIO_BRig_RT__Case_Exp_stateList."SelectWrong_pre" ("Enum")) -> (s? t:f=w2279:T2)
              n927 = Select(t=w2279, s=w2274, f=myRIO_BRig_RT__Case_Exp_stateList."Selection" ("Enum")) -> (s? t:f=w2276:T2)
            }
            frame "Selection" {
              # "counter\nSelection"
              # "increment"
              # "get Tcycle"
              # "get count"
              n928 = xnode "Read/Write Control"("FPGA VI Reference In"=w2329, "error in"=w2328) -> ("error out"=→"error_Selection":errorcluster, "SelectReward"=w2325:bool, "SelectWrong"=w2326:bool)  [unwired: 1 out]
              n929 = call "myRIO_BRig_RT_dataCurrent_Tcycle_generic.vi"() -> ("output_Tcycle_generic"=w2322:i32)  [unwired: 11 in]
              n930 = call "myRIO_BRig_RT_dataCurrent_count_generic.vi"() -> ("output_count_generic"=w2315:i32)  [unwired: 11 in]
              n931 = Index Array(array=w2323, index #1=w2322, index #2=w2315) -> (element #1=w2314:u16, element #2=w2321:u16)
              n932 = call "myRIO_BRig_RT__increment_u16.vi"() -> ("output_increment__u16"=w2320:u16)  [unwired: 11 in]
              n933 = Add(x=w2321, y=w2320) -> (x+y=w2316:u16)
              n934 = Greater?(x=w2314, y=w2316) -> (0:w2308:bool)
              n935 = Select(t=w2319, s=w2308, f=myRIO_BRig_RT__Case_Exp_stateList."SelectTimeout_pre" ("Enum")) -> (s? t:f=w2309:T2)
              n936 = Select(t=w2316, s=w2308, f=w2314) -> (s? t:f=w2312:u16)
              n937 = call "myRIO_BRig_RT_dataCurrent_count_selection.vi"() -> ("output_count_generic"=w2313:i32)  [unwired: 11 in]
              n938 = Select(t=myRIO_BRig_RT__Case_Exp_stateList."SelectReward_pre" ("Enum"), s=w2325, f=myRIO_BRig_RT__Case_Exp_stateList."SelectWrong_pre" ("Enum")) -> (s? t:f=w2324:T2)
              n939 = Replace Array Subset(array=w2323, new element #1=w2312, index #1=w2315, new element #2=w2312, index #2=w2313) -> (w2318:u16[])
              n940 = Or(x=w2325, y=w2326) -> (x .or. y?=w2307:bool)
              n941 = Select(t=w2324, s=w2307, f=w2309) -> (s? t:f=w2327:T2)
            }
            frame "SelectReward_pre" {
              # "iState"
              # "Tcycle\nReward"
              # "nRewTrials"
              # "Tcycle\nGeneric"
              # "counter"
              n942 = call "myRIO_BRig_RT_dataCurrent_nRewTrials.vi"() -> ("output_nRewTrials"=w2361:i32)  [unwired: 11 in]
              n943 = Equal?(x=w2370, y=enum16{"Left", "Right"}."Left") -> (x = y?=w2371:bool)
              n944 = Index Array(array=w2362, index=w2361) -> (element=w2360:u16)
              n945 = call "myRIO_BRig_RT_dataExp_Tcycle_Reward__L.vi"() -> ("output_Tcycle_Reward__L"=w2374:i32)  [unwired: 11 in]
              n946 = call "myRIO_BRig_RT_dataExp_Tcycle_Reward__R.vi"() -> ("output_Tcycle_Reward__R"=w2375:i32)  [unwired: 11 in]
              n947 = Increment(x=w2360) -> (x+1=w2359:u16)
              n948 = Select(t=w2374, s=w2371, f=w2375) -> (s? t:f=w2373:i32)
              n949 = call "myRIO_BRig_RT__Case_Exp_subState_LC__Reward.vi"("input_spout"=w2370, "input_dataCurrent"=w2362, "input_dataLC"=w2369) -> ()  [unwired: 6 in, 2 out]
              n950 = call "myRIO_BRig_RT_dataCurrent_count_generic.vi"() -> ("output_count_generic"=w2364:i32)  [unwired: 11 in]
              n951 = call "myRIO_BRig_RT_dataCurrent_Tcycle_generic.vi"() -> ("output_Tcycle_generic"=w2365:i32)  [unwired: 11 in]
              n952 = Index Array(array=w2376, index=w2373) -> (element=w2366:u16)
              n953 = call "myRIO_BRig_RT_dataCurrent_iState.vi"() -> ("output_iState"=w2354:i32)  [unwired: 11 in]
              n954 = Replace Array Subset(array=w2362, new element #1=w2359, index #1=w2361, new element #2=u16 0 ("new element/subarray"), index #2=w2364, new element #3=w2366, index #3=w2365, new element #4=u16 1 ("new element/subarray"), index #4=w2354) -> (w2377:u16[])
            }
            frame "SelectReward" {
              n955 = call "myRIO_BRig_RT__Case_Exp_State_Reward.vi"("input_dataCurrent"=w2398, "input_state"=w2395, "input_spout"=w2393) -> ("output_dataCurrent"=w2397:u16[], "output_state"=w2396:T2, "output__L"=w2391:bool, "output__R"=w2392:bool)  [unwired: 9 in]
            }
            frame "SelectRewardPost_pre" {
              # "nRewards"
              # "nRewTrials"
              # "Tcycle"
              # "counter"
              n956 = call "myRIO_BRig_RT_dataBlock_nRewards__L.vi"() -> ("output_nRewards__L"=w2414:i32)  [unwired: 11 in]
              n957 = call "myRIO_BRig_RT_dataBlock_nRewards__R.vi"() -> ("output_nRewards__R"=w2413:i32)  [unwired: 11 in]
              n958 = call "myRIO_BRig_RT_dataCurrent_Tcycle_generic.vi"() -> ("output_Tcycle_generic"=w2433:i32)  [unwired: 11 in]
              n959 = call "myRIO_BRig_RT_dataCurrent_count_generic.vi"() -> ("output_count_generic"=w2435:i32)  [unwired: 11 in]
              n960 = case shown="\"Left\", Default" w2407 {
                tunnel: w2419 -> [w2440 w2444]
                tunnel: [w2439 w2444] -> w2418
                tunnel: [w2441 w2442] -> w2417
                tunnel: w2416 -> [w2441 w2443]
                frame "Left", Default {
                  n961 = Increment(x=w2440) -> (x+1=w2439:u16)
                }
                frame "Right" {
                  n962 = Increment(x=w2443) -> (x+1=w2442:u16)
                }
              }
              "nRewards_Left" <- w2418
              "nRewards_Right" <- w2417
              n963 = Equal?(x=w2407, y=enum16{"Left", "Right"}."Left") -> (x = y?=w2406:bool)
              n964 = Select(t=w2414, s=w2406, f=w2413) -> (s? t:f=w2412:i32)
              n965 = call "myRIO_BRig_RT_dataExp_Tcycle_RewardPost.vi"() -> ("output_Tcycle_RewardPost"=w2429:i32)  [unwired: 11 in]
              n966 = call "myRIO_BRig_RT_dataCurrent_nRewTrials.vi"() -> ("output_nRewTrials"=w2415:i32)  [unwired: 11 in]
              n967 = Index Array(array=w2430, index=w2429) -> (element=w2432:u16)
              n968 = Index Array(array=w2409, index=w2415) -> (element=w2404:u16)
              n969 = Replace Array Subset(array=w2409, new element #1=u16 0 ("new element/subarray"), index #1=w2435, new element #2=w2432, index #2=w2433) -> (w2431:u16[])
              n970 = Replace Array Subset(array=w2411, new element=w2404, index (row)=w2405, index (col)=w2412) -> (w2410:u16[][])
              n971 = local write "nRewards_cur"(w2404) -> ()
            }
            frame "SelectRewardPost" {
              n972 = call "myRIO_BRig_RT__Case_Exp_State_RewardPost.vi"("input_state"=w2459, "input_dataCurrent"=w2462) -> ("output_state"=w2460:T2, "output_dataCurrent"=w2461:u16[])  [unwired: 8 in]
            }
            frame "SelectWrong_pre" {
              # "iState"
              # "Tcycle"
              # "counter"
              n973 = call "myRIO_BRig_RT_dataCurrent_Tcycle_generic.vi"() -> ("output_Tcycle_generic"=w2487:i32)  [unwired: 11 in]
              n974 = call "myRIO_BRig_RT_dataCurrent_count_generic.vi"() -> ("output_count_generic"=w2489:i32)  [unwired: 11 in]
              n975 = call "myRIO_BRig_RT_dataExp_Tcycle_Wrong.vi"() -> ("output_Tcycle_Wrong"=w2485:i32)  [unwired: 11 in]
              n976 = call "myRIO_BRig_RT__Case_Exp_subState_LC__Wrong.vi"("input_spout"=w2481, "input_dataCurrent"=w2482, "input_dataLC"=w2479) -> ()  [unwired: 6 in, 2 out]
              n977 = Index Array(array=w2483, index=w2485) -> (element=w2486:u16)
              n978 = call "myRIO_BRig_RT_dataCurrent_iState.vi"() -> ("output_iState"=w2473:i32)  [unwired: 11 in]
              n979 = Replace Array Subset(array=w2482, new element #1=u16 0 ("new element/subarray"), index #1=w2489, new element #2=w2486, index #2=w2487, new element #3=u16 2 ("new element/subarray"), index #3=w2473) -> (w2484:u16[])
            }
            frame "SelectWrong" {
              n980 = call "myRIO_BRig_RT__Case_Exp_State_Wrong.vi"("input_state"=w2503, "input_dataCurrent"=w2512) -> ("output_state"=w2500:T2, "output_dataCurrent"=w2511:u16[])  [unwired: 8 in]
              n981 = Not Equal?(x=w2503, y=w2500) -> (x != y?=w2502:bool)
              n982 = Select(t=myRIO_BRig_RT__Case_Exp_stateList."SelectWrong_post" ("Enum"), s=w2502, f=w2500) -> (s? t:f=w2499:T2)
            }
            frame "SelectWrong_post" {
            }
            frame "SelectTimeout_pre" {
              # "iState"
              # "Tcycle"
              # "counter"
              n983 = xnode "Read/Write Control"("FPGA VI Reference In"=w2539, "error in"=w2538, "SelectionState"=FALSE) -> ("error out"=→"error out 3":errorcluster)  [unwired: 1 out]
              n984 = call "myRIO_BRig_RT_dataCurrent_Tcycle_generic.vi"() -> ("output_Tcycle_generic"=w2561:i32)  [unwired: 11 in]
              n985 = call "myRIO_BRig_RT_dataCurrent_count_generic.vi"() -> ("output_count_generic"=w2559:i32)  [unwired: 11 in]
              n986 = call "myRIO_BRig_RT_dataExp_Tcycle_Timeout.vi"() -> ("output_Tcycle_Timeout"=w2563:i32)  [unwired: 11 in]
              n987 = call "myRIO_BRig_RT__Case_Exp_subState_LC__Timeout.vi"("input_spout"=w2554, "input_dataCurrent"=w2555, "input_dataLC"=w2553) -> ()  [unwired: 6 in, 2 out]
              n988 = Index Array(array=w2557, index=w2563) -> (element=w2562:u16)
              n989 = call "myRIO_BRig_RT_dataCurrent_iState.vi"() -> ("output_iState"=w2547:i32)  [unwired: 11 in]
              n990 = Replace Array Subset(array=w2555, new element #1=u16 0 ("new element/subarray"), index #1=w2559, new element #2=w2562, index #2=w2561, new element #3=u16 3 ("new element/subarray"), index #3=w2547) -> (w2558:u16[])
            }
            frame "SelectTimeout" {
              n991 = call "myRIO_BRig_RT__Case_Exp_State_Timeout.vi"("input_dataLC"=w2582, "input_LC"=w2583, "input_state"=w2573, "input_dataCurrent"=w2588) -> ("output_state"=w2574:T2, "output_dataCurrent"=w2587:u16[])  [unwired: 5 in, 1 out]
              n992 = Not Equal?(x=w2573, y=w2574) -> (x != y?=w2577:bool)
              n993 = Select(t=myRIO_BRig_RT__Case_Exp_stateList."SelectTimeout_post" ("Enum"), s=w2577, f=w2574) -> (s? t:f=w2575:T2)
            }
            frame "SelectTimeout_post" {
            }
            frame "endTrial1" {
              # "Update dataBlock"
              n994 = call "myRIO_BRig_RT__Case_Exp_State_endTrial1.vi"("input_spout"=w2621, "input_dataBlock"=w2620, "input_dataCurrent"=w2618) -> ("output_dataBlock"=w2619:u16[][], "output_dataCurrent"=w2617:u16[])  [unwired: 7 in]
            }
            frame "endTrial2" {
              # "update dataTrial"
              n995 = call "myRIO_BRig_RT__Case_Exp_State_endTrial2.vi"("input_spout"=w2640, "input_dataTrial"=w2644, "input_dataCurrent"=w2642) -> ("output_dataTrial"=w2643:u16[][], "output_dataCurrent"=w2641:u16[])  [unwired: 7 in]
            }
            frame "endTrial3" {
              w2670 = myRIO_BRig_RT__Case_Exp_stateList."endBlock" ("Enum")
              # "nRewTrials"
              # "iTrial"
              # "I_blockUntilReward"
              # "TPB"
              # "end block?"
              n996 = local read "STOP_endTrial"() -> (w2668:bool)
              n997 = local read "STOP_abort"() -> (w2667:bool)
              n998 = xnode "Read/Write Control"("FPGA VI Reference In"=w2656, "error in"=w2655, "SelectionState"=FALSE) -> ("error out"=→"error out 2":errorcluster)  [unwired: 1 out]
              n999 = local read "START"() -> (w2665:bool)
              n1000 = call "myRIO_BRig_RT_dataExp_IblockUntilReward.vi"() -> ("output_I_blockUntilReward"=w2677:i32)  [unwired: 11 in]
              n1001 = Index Array(array=w2661, index=w2677) -> (element=w2657:u16)
              n1002 = Not(x=w2665) -> (.not. x?=w2666:bool)
              n1003 = Not Equal To 0?(x=w2657) -> (x != 0?=w2675:bool)
              n1004 = Compound Arithmetic op=OR(w2668, w2666, w2667) -> (w2669:bool)
              n1005 = call "myRIO_BRig_RT_dataCurrent_nRewTrials.vi"() -> ("output_nRewTrials"=w2673:i32)  [unwired: 11 in]
              n1006 = call "myRIO_BRig_RT_dataCurrent_iTrial.vi"() -> ("output_iTrial"=w2674:i32)  [unwired: 11 in]
              n1007 = Select(t=w2673, s=w2675, f=w2674) -> (s? t:f=w2672:i32)
              n1008 = call "myRIO_BRig_RT_dataCurrent_TpB.vi"() -> ("output_TpB"=w2676:i32)  [unwired: 11 in]
              n1009 = Index Array(array=w2662, index #1=w2676, index #2=w2672) -> (element #1=w2663:u16, element #2=w2664:u16)
              n1010 = Less Or Equal?(x=w2663, y=w2664) -> (x <= y?=w2660:bool)
              n1011 = Select(t=w2670, s=w2660, f=myRIO_BRig_RT__Case_Exp_stateList."empty_endTrial1" ("Enum")) -> (s? t:f=w2671:T2)
              n1012 = Select(t=w2670, s=w2669, f=w2671) -> (s? t:f=w2658:T2)
            }
            frame "endBlock" {
              # "R"
              # "L"
              # "idxDataBlock"
              n1013 = Equal?(x=w2701, y=enum16{"Left", "Right"}."Left") -> (x = y?=w2700:bool)
              n1014 = call "myRIO_BRig_RT_dataCurrent_idxDataBlockL.vi"() -> ("output_idxDataBlock__L"=w2704:i32)  [unwired: 11 in]
              n1015 = call "myRIO_BRig_RT_dataCurrent_idxDataBlockR.vi"() -> ("output_idxDataBlock__R"=w2703:i32)  [unwired: 11 in]
              n1016 = Increment(x=w2695) -> (x+1=w2694:i32)
              n1017 = Select(t=w2704, s=w2700, f=w2703) -> (s? t:f=w2698:i32)
              n1018 = To Unsigned Word Integer(number=w2694) -> (unsigned 16bit integer=w2696:u16)
              n1019 = local read "START"() -> (w2724:bool)
              n1020 = local read "STOP_endBlock"() -> (w2719:bool)
              n1021 = local read "STOP_endTrial"() -> (w2722:bool)
              n1022 = local read "STOP_abort"() -> (w2721:bool)
              n1023 = Replace Array Subset(array=w2699, new element=w2696, index=w2698) -> (w2697:u16[])
              n1024 = Not(x=w2724) -> (.not. x?=w2723:bool)
              n1025 = Compound Arithmetic op=OR(w2723, w2719, w2722, w2721) -> (w2720:bool)
              n1026 = Select(t=myRIO_BRig_RT__Case_Exp_stateList."endExp" ("Enum"), s=w2720, f=myRIO_BRig_RT__Case_Exp_stateList."empty_endBlock1" ("Enum")) -> (s? t:f=w2728:T2)
            }
            frame "endExp" {
            }
            frame "commConnect" {
              n1027 = call "myRIO_BRig_RT_comm_webdav_connect.vi"("input_password"="Host Password", "input_username"="Host UserName") -> ("output_Iconnected"=w2749:bool, "output_hSession"=w2767:T6)  [unwired: 7 in, 1 out]
              "Connected To Host?" <- w2749
              n1028 = case shown="False" w2749 {
                frame False {
                  n1029 = One Button Dialog(message="Connection Failed!\nData not being saved!") -> ()  [unwired: 1 in, 1 out]
                }
                frame True {
                }
              }
            }
            frame "commUpload_pre" {
              n1030 = Select(t=myRIO_BRig_RT__Case_Exp_stateList."commUpload_dataBlock" ("Enum"), s=w2774, f=myRIO_BRig_RT__Case_Exp_stateList."endTrial3") -> (s? t:f=w2772:T2)
            }
            frame "commUpload_dataBlock" {
              n1031 = call "myRIO_BRig_RT_comm_webdav_uploadFile__data.vi"("input_fileName_prefix"=w2795, "input_fileName"="dataBlock" ("input_filename"), "input_hSession"=w2797) -> ()  [unwired: 8 in, 1 out]
            }
            frame "commUpload_dataCurrent" {
              n1032 = call "myRIO_BRig_RT_comm_webdav_uploadFile__data.vi"("input_fileName_prefix"=w2816, "input_fileName"="dataCurrent" ("input_filename"), "input_hSession"=w2818) -> ()  [unwired: 8 in, 1 out]
            }
            frame "commUpload_dataExp" {
              n1033 = call "myRIO_BRig_RT_comm_webdav_uploadFile__data.vi"("input_fileName_prefix"=w2837, "input_fileName"="dataExp" ("input_filename"), "input_hSession"=w2839) -> ()  [unwired: 8 in, 1 out]
            }
            frame "commUpload_dataLC" {
              n1034 = call "myRIO_BRig_RT_comm_webdav_uploadFile__data.vi"("input_fileName_prefix"=w2858, "input_fileName"="dataLC" ("input_filename"), "input_hSession"=w2860) -> ()  [unwired: 8 in, 1 out]
            }
            frame "commUpload_dataTrial" {
              n1035 = call "myRIO_BRig_RT_comm_webdav_uploadFile__data.vi"("input_fileName_prefix"=w2882, "input_fileName"="dataTrial" ("input_filename"), "input_hSession"=w2884) -> ()  [unwired: 8 in, 1 out]
            }
            frame "saveData_dataBlock" {
              # "idxDataBlockR"
              # "idxDataBlockL"
              n1036 = call "myRIO_BRig_RT_dataCurrent_idxDataBlockL.vi"() -> ("output_idxDataBlock__L"=w2908:i32)  [unwired: 11 in]
              n1037 = call "myRIO_BRig_RT_dataCurrent_idxDataBlockR.vi"() -> ("output_idxDataBlock__R"=w2909:i32)  [unwired: 11 in]
              n1038 = Index Array(array=w2910, index #1=w2908, index #2=w2909) -> (element #1=w2907:u16, element #2=w2906:u16)
              n1039 = Greater?(x=w2907, y=w2906) -> (0:w2905:bool)
              n1040 = Select(t=w2907, s=w2905, f=w2906) -> (s? t:f=w2903:u16)
              n1041 = Increment(x=w2903) -> (x+1=w2902:u16)
              n1042 = To Long Integer(number=w2902) -> (32bit integer=w2901:i32)
              n1043 = Array Subset(array=w2904, length (row)=w2901) -> (w2900:u16[][])  [unwired: 3 in]
              n1044 = call "myRIO_BRig_RT_comm_webdav_saveArrayToFile__2D_u16.vi"("Array"=w2900, "input_filename"="dataBlock") -> ()  [unwired: 10 in]
            }
            frame "saveData_dataCurrent" {
              n1045 = call "myRIO_BRig_RT_comm_webdav_saveArrayToFile__1D_u16.vi"("Array"=w2929, "input_filename"="dataCurrent") -> ()  [unwired: 10 in]
            }
            frame "saveData_dataExp" {
              # "runTime"
              n1046 = Get Date/Time In Seconds() -> (seconds since 1Jan1904=w2957:timestamp)
              n1047 = To Double Precision Float(number=w2957) -> (double precision float=w2956:dbl)
              n1048 = call "myRIO_BRig_RT_dataExp_runTime_seconds.vi"() -> ("output_RunTime_minutes"=w2955:i32)  [unwired: 11 in]
              n1049 = Subtract(x=w2956, y=w2954) -> (x-y=w2951:dbl)
              n1050 = To Unsigned Word Integer(number=w2951) -> (unsigned 16bit integer=w2950:u16)
              n1051 = Replace Array Subset(array=w2949, new element=w2950, index=w2955) -> (w2952:u16[])
              n1052 = call "myRIO_BRig_RT_comm_webdav_saveArrayToFile__1D_u16.vi"("Array"=w2952, "input_filename"="dataExp") -> ()  [unwired: 10 in]
            }
            frame "saveData_dataLC" {
              n1053 = call "myRIO_BRig_RT_comm_webdav_saveArrayToFile__1D_u16.vi"("Array"=w2976, "input_filename"="dataLC") -> ()  [unwired: 10 in]
            }
            frame "saveData_dataTrial" {
              # "idxTrial"
              n1054 = call "myRIO_BRig_RT_dataCurrent_idxDataTrial.vi"() -> ("output_idxDataTrial"=w3001:i32)  [unwired: 11 in]
              n1055 = Index Array(array=w3002, index=w3001) -> (element=w2998:u16)
              n1056 = Increment(x=w2998) -> (x+1=w2997:u16)
              n1057 = To Long Integer(number=w2997) -> (32bit integer=w2996:i32)
              n1058 = Array Subset(array=w2999, length (row)=w2996) -> (w3000:u16[][])  [unwired: 3 in]
              n1059 = call "myRIO_BRig_RT_comm_webdav_saveArrayToFile__2D_u16.vi"("Array"=w3000, "input_filename"="dataTrial") -> ()  [unwired: 10 in]
            }
            frame "empty_endBlock1" {
            }
            frame "empty_endBlock2" {
            }
            frame "empty_endTrial1" {
            }
            frame "empty_endTrial2" {
            }
            frame "empty_endTrial3" {
            }
            frame "empty_endTrial4" {
            }
            frame "empty_endTrial5" {
            }
          }
          n1060 = Select(t=w1069, s=w1072, f=w1070) -> (s? t:f=w1071:bool)
          n1061 = case shown="True" w1146 {
            tunnel: w1143 -> [w1169 w1177]
            tunnel: w1145 -> [_ w1173]
            tunnel: w1144 -> [_ w1172]
            tunnel: w1046 -> [_ w1171]
            tunnel: w1113 -> [_ w1170]
            tunnel: [w1169 w1176] -> w1142
            tunnel: w1141 -> [w1168 w1175]
            tunnel: [w1168 w1174] -> w1140
            frame False {
            }
            frame True {
              n1062 = call "myRIO_BRig_RT__Case_Exp__recordLick.vi"("intput_state__trialEnd"=w1170, "intput_state__trialStart"=w1171, "input_lick__R"=w1172, "input_lick__L"=w1173, "input_dataCurrent"=w1175, "input_dataLick"=w1177) -> ("output_dataCurrent"=w1174:u16[], "output_dataLick"=w1176:u16[][])  [unwired: 4 in]
            }
          }
          n1063 = Or(x=w1115, y=w1116) -> (x .or. y?=w1102:bool)
          n1064 = Or(x=w1119, y=w1099) -> (x .or. y?=w1088:bool)
          n1065 = Or(x=w1098, y=w1120) -> (x .or. y?=w1114:bool)
          n1066 = Or(x=w1118, y=w1117) -> (x .or. y?=w1103:bool)
          n1067 = Or(x=w1147, y="STOP_abort") -> (x .or. y?=w1149:bool)
          n1068 = Or(x=w1077, y=w1078) -> (x .or. y?=w1075:bool)
          n1069 = Or(x=w1079, y=w1078) -> (x .or. y?=w1076:bool)
          n1070 = Select(t=w1058, s=w1059, f=w1057) -> (s? t:f=w1048:u16)
          n1071 = Select(t=w1060, s=w1062, f=w1061) -> (s? t:f=w1049:u16)
          n1072 = Select(t=u16 0, s=w1065, f=w1064) -> (s? t:f=w1047:u16)
          n1073 = xnode "Read/Write Control"("FPGA VI Reference In"=w1090, "error in"=w1089, "A1_SR"=w1103, "A3_SL"=w1102, "A6_Act"=w1071, "audioTrigger_L"=w1088, "audioAmp_L"=w1129, "audioFreq_L_kHz"=w1097, "audioTrigger_R"=w1114, "audioAmp_R"=w1130, "audioFreq_R_kHz"=w1131, "laserledMTrig"=w1075, "laserMTrig"=w1076) -> ("FPGA VI Reference Out"=w1139:refnum<k20>, "error out"=w1138:errorcluster, "AnaIn_0"=w1045:i16, "AnaIn_1"=w1044:i16)
          n1074 = local write "tempAI0"(w1045) -> ()
          n1075 = call "myRIO_BRig_RT_dataAnalog_enterData__PortC.vi"("input_iState"=w1046, "input_AI0"=w1045, "input_iEvent"=w1047, "input_AI1"=w1044, "input_iTrial"=w1048, "input_iBlock"=w1049, "input_index"=w1050, "input_dataAnalog"=w1068) -> ("output_dataAnalog"=w1067:u16[][])  [unwired: 3 in]
          n1076 = call "myRIO_BRig_RT_TCP.vi"("input_hTCP"=w1055, "input_AI1"=w1044, "input_AI0"=w1045, "input_I_connected_TCP"=w1051, "input_index"=w1050, "input_iBlock"=w1049, "input_iTrial"=w1048, "input_error"=w1053, "input_iEvent"=w1047, "input_iState"=w1046) -> ("output_hTCP"=w1054:refnum<k5>, "output_error"=w1052:errorcluster)  [unwired: 4 in]
          n1077 = node-c288() -> ()  [unwired: 1 in, 1 out]
          n1078 = Increment(x=w1047) -> (x+1=w1056:u16)
          n1079 = Increment(x=w1050) -> (x+1=w1066:i32)
          "cState" <- w1046
        }
        n1080 = node-c288(w994) -> ()  [unwired: 1 out]
        n1081 = flat-sequence {
          tunnel: w990 -> [w1039]
          tunnel: w989 -> [w1038]
          tunnel: [w1037] -> w982
          tunnel: [w1036] -> w981
          tunnel: [w1042] -> w983
          tunnel: [w1043] -> w988
          tunnel: w982 -> [w1043]
          tunnel: w981 -> [w1042]
          frame #0 {
            w1033 = u8 0
            w1034 = u16 0 ("AudioLeft_phase_inc")
            w1035 = FALSE
            n1082 = xnode "Read/Write Control"("FPGA VI Reference In"=w1039, "error in"=w1038, "Counts_Reset"=TRUE, "audioTrigger_L"=w1035, "audioFreq_L_kHz"=w1033, "audioAmp_L"=w1034, "audioTrigger_R"=w1035, "audioFreq_R_kHz"=w1033, "audioAmp_R"=w1034, "A3_SL"=w1035, "A1_SR"=w1035, "A6_Act"=w1035) -> ("FPGA VI Reference Out"=w1037:refnum<k20>, "error out"=w1036:errorcluster)
          }
          frame #1 {
            w1041 = FALSE ("START")
            n1083 = local write "START"(w1041) -> ()
            n1084 = local write "STOP_endTrial"(w1041) -> ()
            n1085 = local write "STOP_endBlock"(w1041) -> ()
          }
        }
        n1086 = stacked-sequence {
          tunnel: w966 -> [w1013 _]
          tunnel: w964 -> [w1014 _]
          tunnel: w963 -> [_ w1019]
          tunnel: w962 -> [_ w1018]
          tunnel: w961 -> [_ w1017]
          tunnel: w960 -> [w1007 _]
          tunnel: w933 -> [w1004 _]
          tunnel: w932 -> [w1003 _]
          frame #0 {
            n1087 = call "myRIO_BRig_RT_dataCurrent_idxDataLick.vi"() -> ("output_idxDataLick"=w1008:i32)  [unwired: 11 in]
            n1088 = Index Array(array=w1007, index=w1008) -> (element=w1010:u16)
            n1089 = Array Subset(array=w1004, length (row)=w1003) -> (w1005:u16[][])  [unwired: 3 in]
            n1090 = Increment(x=w1010) -> (x+1=w1011:u16)
            n1091 = call "myRIO_BRig_RT_comm_webdav_saveArrayToFile__1D_u16.vi"("Array"=w1014, "input_filename"="dataMTrig") -> ()  [unwired: 10 in]
            n1092 = To Long Integer(number=w1011) -> (32bit integer=w1009:i32)
            n1093 = Array Subset(array=w1013, length (row)=w1009) -> (w1012:u16[][])  [unwired: 3 in]
            n1094 = call "myRIO_BRig_RT_comm_webdav_saveArrayToFile__2D_u16.vi"("Array"=w1012, "input_filename"="dataLick") -> ()  [unwired: 10 in]
            n1095 = call "myRIO_BRig_RT_comm_webdav_saveArrayToFile__2D_u16.vi"("Array"=w1005, "input_filename"="dataAnalog") -> ()  [unwired: 10 in]
          }
          frame #1 {
            n1096 = case shown="True" w1019 {
              tunnel: w1018 -> [_ w1021]
              tunnel: w1017 -> [_ w1020]
              frame False {
              }
              frame True {
                n1097 = stacked-sequence {
                  tunnel: w1021 -> [w1023 w1030 w1032]
                  tunnel: w1020 -> [w1024 w1029 _]
                  frame #0 {
                    n1098 = call "myRIO_BRig_RT_comm_webdav_uploadFile__announce.vi"("input_addText"=TRUE, "input_fileName_prefix"=w1024, "intput_fileName"="curExp_end", "intput_hSession"=w1023) -> ("output_Isuccess"=w1022:bool)  [unwired: 6 in, 1 out]
                    n1099 = case shown="True" w1022 {
                      frame False {
                        n1100 = One Button Dialog(message="!!! Warning !!! Your data is located at C:\\BehaviorRig\\commTransfer") -> ()  [unwired: 1 in, 1 out]
                      }
                      frame True {
                        n1101 = Wait (ms)(milliseconds to wait=u32 20) -> ()  [unwired: 1 out]
                      }
                    }
                  }
                  frame #1 {
                    n1102 = call "myRIO_BRig_RT__endExp_sendData.vi"("input_fileName_prefix"=w1029, "input_hSession"=w1030) -> ()  [unwired: 8 in, 2 out]
                  }
                  frame #2 {
                    n1103 = local write "Connected To Host?"(FALSE ("Connected To Host?")) -> ()
                    n1104 = call <vilib>:"Close Session.vi"("session handle"=w1032) -> ()  [unwired: 14 in, 1 out]
                  }
                }
              }
            }
          }
        }
      }
    }
    n1105 = local read "STOP_abort"() -> (w43:bool)
  }
  n1106 = case shown="True" w3 {
    tunnel: w2 -> [_ w3156]
    tunnel: w1 -> [_ w3155]
    frame False {
    }
    frame True {
      n1107 = call "myRIO__TCP_disconnect_forWrite.vi"("input_error"=w3155, "input_hTCP"=w3156) -> ()  [unwired: 9 in, 1 out]
    }
  }
  n1108 = xnode "Read/Write Control"("FPGA VI Reference In"=w15, "error in"=w14, "FPGA_Stop"=TRUE) -> ("FPGA VI Reference Out"=w20:refnum<k20>, "error out"=w21:errorcluster)
  n1109 = xnode "Close FPGA VI Reference"("FPGA VI Reference In"=w20, "error in"=w21) -> ("error out"=w19:errorcluster)
  n1110 = call <vilib>:"Reset myRIO.vi"("error in (no error)"=w19) -> ()  [unwired: 10 in, 1 out]
